vi "Oxford-1820-Main.vi"() -> ()   [LabVIEW 2016]
uses:
  <instrlib>/Mercury iXX/Public/Controls/Unit String.ctl
  <instrlib>/Mercury iXX/Public/Libraries/Heater/Controls/Heater Device (Read).ctl
  <instrlib>/Mercury iXX/Public/Controls/Manufacturing Data.ctl
  <instrlib>/Mercury iXX/Public/Libraries/Heater/Controls/Heater Signals Cluster.ctl
  <instrlib>/Mercury iXX/Public/Libraries/Level Meter/Controls/Level Meter (Read).ctl
  <instrlib>/Mercury iXX/Public/Libraries/Level Meter/Controls/Nitrogen Configuration.ctl
  <instrlib>/Mercury iXX/Public/Libraries/Level Meter/Controls/Frequency Configuration.ctl
  <instrlib>/Mercury iXX/Public/Libraries/Level Meter/Controls/Signals.ctl
  <instrlib>/Mercury iXX/Public/Libraries/Level Meter/Controls/Helium Configuration.ctl
  <instrlib>/Mercury iXX/Public/Libraries/Level Meter/Controls/Resistance Configuration.ctl
  <instrlib>/Mercury iXX/Public/Libraries/Level Meter/Controls/Pre-Pulse.ctl
  <instrlib>/Mercury iXX/Public/Libraries/Level Meter/Controls/Pulse.ctl
  <instrlib>/Mercury iXX/Public/Libraries/Auxiliary/Controls/AUX Device (Read).ctl
  <instrlib>/Mercury iXX/Public/Libraries/Auxiliary/Controls/AUX Signals (Read).ctl
  <instrlib>/Mercury iXX/Public/Libraries/Magnet/Controls/Device (Read).ctl
  <instrlib>/Mercury iXX/Public/Libraries/Magnet/Controls/Signals (Read).ctl
  <instrlib>/Mercury iXX/Public/Libraries/Magnet/Controls/Identifier.ctl
  <instrlib>/Mercury iXX/Public/Libraries/Temperature/Controls/Calibration Cluster.ctl
  <instrlib>/Mercury iXX/Public/Libraries/Temperature/Controls/Calibration Interpolation.ctl
  <instrlib>/Mercury iXX/Public/Libraries/Temperature/Controls/Excitation Cluster.ctl
  <instrlib>/Mercury iXX/Public/Libraries/Temperature/Controls/Excitation Type.ctl
  <instrlib>/Mercury iXX/Public/Libraries/Pressure/Controls/Pressure Signals Cluster.ctl
  <instrlib>/Mercury iXX/Mercury iXX.lvlib
  <instrlib>/Mercury iXX/Public/Controls/Comms Transport Layer.ctl
  <instrlib>/Mercury iXX/Public/Libraries/Pressure/Open/Open Pressure Device.vi
  <instrlib>/Mercury iXX/Public/Libraries/Pressure.lvlib
  <instrlib>/Mercury iXX/Public/Libraries/Pressure/Configuration/Read/Pressure Device (Read).vi
  <instrlib>/Mercury iXX/Public/Libraries/System/Read/Display Automatic Dimming (Read).vi
  <instrlib>/Mercury iXX/Public/Libraries/System.lvlib
  <instrlib>/Mercury iXX/Public/Libraries/System/Read/Display Automatic Dimming Time (Read).vi
  <instrlib>/Mercury iXX/Public/Libraries/System/Read/Display Brightness (Read).vi
  <instrlib>/Mercury iXX/Public/Libraries/System/Read/Mode (Read).vi
  <instrlib>/Mercury iXX/Public/Libraries/System/Read/Serial Number (Read).vi
  <instrlib>/Mercury iXX/Public/Libraries/System/Read/FVer (Read).vi
  <instrlib>/Mercury iXX/Public/Libraries/System/Read/HVer (Read).vi
  <instrlib>/Mercury iXX/Public/Libraries/System/Set/DateTime (Set).vi
  <instrlib>/Mercury iXX/Public/Libraries/Temperature/Signals/Read/Temperature (Read).vi
  <instrlib>/Mercury iXX/Public/Libraries/Temperature.lvlib
  <instrlib>/Mercury iXX/Public/Libraries/Temperature/Configuration/Read/Calibration Cold Limit (Read).vi
  <instrlib>/Mercury iXX/Public/Libraries/Temperature/Configuration/Read/Calibration Hot Limit (Read).vi
  <instrlib>/Mercury iXX/Public/Libraries/Temperature/Configuration/Read/Excitation Type (Read).vi
  <instrlib>/Mercury iXX/Public/Libraries/Temperature/Configuration/Read/Temperature Sensor (Read).vi
  <instrlib>/Mercury iXX/Public/Libraries/Temperature/Configuration/Read/Temperature Device (Read).vi
  <instrlib>/Mercury iXX/Public/Libraries/Temperature/Configuration/Read/Nickname (Read).vi
  <instrlib>/Mercury iXX/Public/Libraries/Temperature/Configuration/Read/Excitation Magnitude (Read).vi
  <instrlib>/Mercury iXX/Public/Libraries/Temperature/Configuration/Read/Serial Number (Read).vi
  <instrlib>/Mercury iXX/Public/Libraries/System/Read/Catalogue (Read).vi
  <instrlib>/Mercury iXX/Public/Libraries/System/Read/Flash Space (Read).vi
  <instrlib>/Mercury iXX/Public/Libraries/System/Read/DateTime (Read).vi
  <instrlib>/Mercury iXX/Public/Libraries/System/Read/Time (Read).vi
  <instrlib>/Mercury iXX/Public/Libraries/System/Read/Date (Read).vi
  <instrlib>/Mercury iXX/Public/Libraries/System/Open/Open System.vi
  <instrlib>/Mercury iXX/Public/Libraries/Temperature/Open/Open Temperature Device.vi
  <instrlib>/Mercury iXX/Public/Libraries/Auxiliary/Open/Open Auxiliary Device.vi
  <instrlib>/Mercury iXX/Public/Libraries/Auxiliary.lvlib
  <instrlib>/Mercury iXX/Public/Libraries/Auxiliary/Signals/Read/Percent Open (Read).vi
  <instrlib>/Mercury iXX/Public/Libraries/Magnet/Open/Open Magnet Device.vi
  <instrlib>/Mercury iXX/Public/Libraries/Magnet.lvlib
  <instrlib>/Mercury iXX/Public/Libraries/Magnet/Configuration/Read/PSU Action Status (Read).vi
  <instrlib>/Mercury iXX/Public/Libraries/Magnet/Configuration/Read/Magnet Device (Read).vi
  <instrlib>/Mercury iXX/Public/Libraries/Temperature/Signals/Read/Voltage (Read).vi
  <instrlib>/Mercury iXX/Private/Controls/Query Dynamic Reference.ctl
  <instrlib>/Mercury iXX/Public/Controls/Mercury Reference.ctl
  <instrlib>/Mercury iXX/Public/Libraries/Level Meter/Open/Open Level Meter Device.vi
  <instrlib>/Mercury iXX/Public/Libraries/Level Meter.lvlib
  <instrlib>/Mercury iXX/Public/Libraries/Level Meter/Signals/Read/Probe Level Nitrogen (Read).vi
  <instrlib>/Mercury iXX/Public/Libraries/Level Meter/Signals/Read/Probe Level Helium (Read).vi
  <instrlib>/Mercury iXX/Public/Libraries/Magnet/Signals/Read/Switch Heater Status (Read).vi
  <instrlib>/Mercury iXX/Public/Libraries/Magnet/Signals/Read/Current (Read).vi
  <instrlib>/Mercury iXX/Public/Libraries/Magnet/Configuration/Set/PSU Action Status (Set).vi
  <instrlib>/Mercury iXX/Public/Libraries/Magnet/Controls/PSU Actions.ctl
  <instrlib>/Mercury iXX/Public/Libraries/Magnet/Controls/Switch Heater.ctl
  SMOs/Instrument.Oxford1820/Instrument.Oxford1820.lvclass
  <instrlib>/Mercury iXX/Public/Libraries/Lambda/Configuration/Set/Lambda Percentage Flow (Set).vi
  <instrlib>/Mercury iXX/Public/Libraries/Lambda.lvlib
  <instrlib>/Mercury iXX/Public/Libraries/Lambda/Open/Open Lambda Device.vi
  <instrlib>/Mercury iXX/Public/Controls/Response String.ctl
  <instrlib>/Mercury iXX/Public/Libraries/Temperature/Signals/Read/Resistance (Read).vi
  <instrlib>/Mercury iXX/Public/Libraries/Temperature/Configuration/Set/Excitation Magnitude (Set).vi
  <instrlib>/Mercury iXX/Public/Libraries/Magnet/Signals/Read/Voltage (Read).vi
  SMOs/Instrument.Oxford1820/Typedefs/Status.ctl
  SMOs/Instrument.Oxford1820/Typedefs/Actions.ctl
  <instrlib>/Mercury iXX/Public/Libraries/System/Controls/User Mode.ctl
  <instrlib>/Mercury iXX/Public/Libraries/System/Set/Mode (Set).vi
  <instrlib>/Mercury iXX/Public/Libraries/Heater/Signals/Read/Power (Read).vi
  <instrlib>/Mercury iXX/Public/Libraries/Heater.lvlib
  <instrlib>/Mercury iXX/Public/Libraries/Heater/Signals/Read/Current (Read).vi
  <instrlib>/Mercury iXX/Public/Libraries/Auxiliary/Signals/Read/Position (Read).vi
  <instrlib>/Mercury iXX/Public/Libraries/Level Meter/Signals/Read/Probe Count Nitrogen (Read).vi
  <instrlib>/Mercury iXX/Public/Libraries/Magnet/Signals/Read/Current Rate (Read).vi
  <userlib>/_OpenG.lib/error/error.llb/Filter Error Codes (Array)__ogtk.vi
  <instrlib>/Mercury iXX/Public/Libraries/Heater/Configuration/Read/Nickname (Read).vi
  <instrlib>/Mercury iXX/Public/Libraries/Heater/Configuration/Read/Voltage Limit (Read).vi
  <instrlib>/Mercury iXX/Public/Libraries/Heater/Configuration/Read/Serial Number (Read).vi
  <instrlib>/Mercury iXX/Public/Libraries/Heater/Configuration/Read/Heater Device (Read).vi
  <instrlib>/Mercury iXX/Public/Libraries/Heater/Open/Open Heater Device.vi
  <instrlib>/Mercury iXX/Public/Libraries/Heater/Signals/Read/Voltage (Read).vi
  <instrlib>/Mercury iXX/Public/Libraries/Heater/Configuration/Read/Maximum Power (Read).vi
  <instrlib>/Mercury iXX/Public/Libraries/Heater/Configuration/Read/Nominal Resistance (Read).vi
  <instrlib>/Mercury iXX/Public/Libraries/Auxiliary/Configuration/Read/Stepper Speed (Read).vi
  <instrlib>/Mercury iXX/Public/Libraries/Auxiliary/Configuration/Read/Valve Gearing (Read).vi
  <instrlib>/Mercury iXX/Public/Libraries/Auxiliary/Configuration/Read/Temperature Error Voltage Sensitivity (Read).vi
  <instrlib>/Mercury iXX/Public/Libraries/Auxiliary/Configuration/Read/Temperature Error Sensitivity (Read).vi
  <instrlib>/Mercury iXX/Public/Libraries/Auxiliary/Configuration/Read/Gas Flow Scaling (Read).vi
  <instrlib>/Mercury iXX/Public/Libraries/Auxiliary/Configuration/Read/Minimum Gas Flow (Read).vi
  <instrlib>/Mercury iXX/Public/Libraries/Auxiliary/Configuration/Read/Serial Number (Read).vi
  <instrlib>/Mercury iXX/Public/Libraries/Auxiliary/Configuration/Read/Aux Device (Read).vi
  <instrlib>/Mercury iXX/Public/Libraries/Pressure/Signals/Read/Voltage (Read).vi
  <instrlib>/Mercury iXX/Public/Libraries/Pressure/Signals/Read/Current (Read).vi
  <instrlib>/Mercury iXX/Public/Libraries/Pressure/Configuration/Read/Nickname (Read).vi
  <instrlib>/Mercury iXX/Public/Libraries/Level Meter/Signals/Read/Probe Resistance Helium (Read).vi
  <instrlib>/Mercury iXX/Public/Libraries/Level Meter/Configuration/Read/Nitrogen Pulse Count Period (Read).vi
  <instrlib>/Mercury iXX/Public/Libraries/Level Meter/Configuration/Read/Nitrogen Freq at 100 (Read).vi
  <instrlib>/Mercury iXX/Public/Libraries/Level Meter/Configuration/Read/Helium Pulse Duration (Read).vi
  <instrlib>/Mercury iXX/Public/Libraries/Level Meter/Configuration/Read/Helium Pulse Mag (Read).vi
  <instrlib>/Mercury iXX/Public/Libraries/Level Meter/Configuration/Read/Helium Probe Resistance (Read).vi
  <instrlib>/Mercury iXX/Public/Libraries/Level Meter/Configuration/Read/Serial Number (Read).vi
  <instrlib>/Mercury iXX/Public/Libraries/Level Meter/Configuration/Read/Level Meter Device (Read).vi
  <instrlib>/Mercury iXX/Public/Libraries/Magnet/Configuration/Read/Software Voltage Limit (Read).vi
  <instrlib>/Mercury iXX/Public/Libraries/Magnet/Configuration/Read/Switch Present (Read).vi
  <instrlib>/Mercury iXX/Public/Libraries/Magnet/Configuration/Read/Current to Field Factor (Read).vi
  <instrlib>/Mercury iXX/Public/Libraries/Magnet/Configuration/Read/Current Limit (Read).vi
  <instrlib>/Mercury iXX/Public/Libraries/Magnet/Configuration/Read/Output Configuration (Read).vi
  <instrlib>/Mercury iXX/Public/Libraries/Magnet/Configuration/Read/Bipolar Output (Read).vi
  <instrlib>/Mercury iXX/Public/Libraries/Magnet/Configuration/Read/Serial Number (Read).vi
  <instrlib>/Mercury iXX/Public/Libraries/Magnet/Signals/Read/Target Field (Read).vi
  <instrlib>/Mercury iXX/Public/Libraries/Magnet/Signals/Read/Target Field Rate (Read).vi
  <instrlib>/Mercury iXX/Public/Libraries/Magnet/Signals/Read/Field (Read).vi
  <instrlib>/Mercury iXX/Public/Libraries/Magnet/Signals/Read/Persistant Field (Read).vi
  <instrlib>/Mercury iXX/Public/Libraries/Magnet/Configuration/Set/Switch Heater Current (Set).vi
  <instrlib>/Mercury iXX/Public/Libraries/Magnet/Signals/Read/Persistant Current (Read).vi
  <instrlib>/Mercury iXX/Public/Libraries/Magnet/Signals/Set/Switch Heater No Check (Set).vi
  <instrlib>/Mercury iXX/Public/Libraries/Magnet/Signals/Set/Target Field (Set).vi
  <instrlib>/Mercury iXX/Public/Libraries/Magnet/Signals/Set/Target Field Rate (Set).vi
  <instrlib>/Mercury iXX/Public/Libraries/Lambda/Configuration/Set/Lambda Flow Auto (Set).vi
  <instrlib>/Mercury iXX/Public/Libraries/Level Meter/Configuration/Set/Pulse Slow-Fast (Set).vi
panel:
  out "LPF ON":timestamp
  in  "Tab Control":T1(tab)
  in  "Enable RS232 Panel":bool
  out "LEDs":bool[](array[boolean])
  out "Iteration Time":dbl
  in  "Percentage Open":dbl=100.0 format="%#_13g"
  out "PS Heat on or off (sec)":dbl format="%<%H:%M:%S>t"
  out "LPF on (min)":dbl=5373.0 format="%<%H:%M:%S>t"
  out "Magnet Status 2":string
  in  "OK":bool
  out "LPF Resistance":dbl=4.2075 format="%_3f ohms"
  out "Magnet Resistance":dbl=3.8705 format="%_3f ohms"
  out "ETA":timestamp format="%<%I:%M:%S %p\n%m/%d/%y>T"
  in  "Open Needle Valve":bool
  in  "Close Needle Valve":bool
  in  "Lambda":bool
  out "LPF Pressure":dbl format="%_5f mB"
  out "LPF Needle Valve (%)":dbl format="%_6g"
  out "LPF Temperature":dbl=4.2075 format="%_2f K"
  out "Magnet Temperature":dbl=3.8705 format="%_2f K"
  out "He LVL Chart":dbl(slide)=52.0833 scale=0.0..100.0
  out "N2 LVL Chart":dbl(slide)=61.3025 scale=0.0..100.0
  in  "Remote Mode":bool
  out "Power Supply Field (T)":dbl=0.0001 format="%#.5f"
  out "Magnet Field (T)":dbl format="%.5f"
  out "Voltage (V)":dbl=-0.0003 format="%.5f"
  out "Current (A)":dbl=0.0006 format="%.5f"
  out "N2 LEVEL":dbl=61.3025 format="%.0f %"
  out "He LEVEL":dbl=52.0833 format="%.0f %"
  in  "Fast/Slow Fill":bool
  out "Magnet Field (T)":dbl(knob) caption="Voltage (V)" scale=-20.0..20.0
  out "SWITCH HEATER":bool
  in  "PS Heat":bool
  in  "Clamp":bool
  in  "To Set":bool
  in  "To Zero":bool
  in  "Hold":bool
  out "Magnet Status":string="Clamped"
  out "Target Field Rate (T/min)":dbl=1.0 format="%.5f"
  out "Target Field (T)":dbl format="%#.5f"
  in  "Target Rate (T/min)":dbl=0.1 format="%.5f"
  in  "Target Field (T)":dbl format="%#.5f"
  in  "Send to IPS":bool
  out "Voltage (V)":dbl(knob)=-0.0003 scale=-10.0..10.0
  out "Current (A)":dbl(knob)=0.0006 scale=-180.0..180.0
  in  "Mercury Functions":T2(tab)=enum."ITC: Temperature"
  out "time stamp":timestamp=timestamp(3543841780 s since 1904-01-01)
  out "Free Space":i32=166384 caption="Free Space (KB)"
  out "Set Date Response":string="VALID"
  out "String":string="NORM" caption="User Mode"
  out "Date":string="2016:04:18"
  out "Time":string="11:29:40"
  out "Hardware Version":string="65"
  out "Firmware Version":string="2.2.6.20"
  out "Serial Number":string="154650110"
  out "ITC Devices":string[](array[string])=["DB4.G1:AUX", "DB8.P1:PRES", "MB0.H1:HTR", "MB1.T1:TEMP"]
  out "S/W Version(s)":string[](array[string])=["2.2.6.20\n"]
  out "Serial Number(s)":string[](array[string])=["154650110"]
  out "# of Instruments":i32=1
  out "Automatic Dimming":string="OFF"
  out "Dimming Time":string="5"
  out "Display Brightness":string="100"
  in  "ITC IP Address":string="130.49.180.101"
  out "Excitation Magnitude":dbl=5.0
  out "Sensor Type":string="NTC"
  out "Excitation Type":string="UNIP"
  out "Hot Limit":dbl=1000.0
  out "H Unit":T3="K"
  out "Cold Limit":dbl=1000.0
  out "C Unit":T3="K"
  out "Unit":T3
  out "Voltage":dbl=0.005
  out "V Unit":T3="V"
  out "Temperature":dbl=4.2075
  out "T Unit":T3="K"
  out "Temp S/N":string="154650110"
  out "T Nickname":string="Mag_AB_MB1"
  out "ITC Calibration":T4
  out "ITC Excitation":T6
  out "ITC Manufacturing":T8
  out "Heater Device Settings":T9={"Manufacturing"={"Hardware Version"="65", "Firmware Version"="2.3", "Serial Number"="154650110"}, "Nickname"="MB0.H1", "Voltage Limit"="1", "Nominal Resistance"="10", "Maximum Power"="0.1000", "Heater Signals"={"Voltage"="0.0507V", "Current"="-0.0000A", "Power"="0.0000W"}, "Status"="2"}
  out "Htr C Unit":T3="A"
  out "Htr P Unit":T3="W"
  out "Htr V Unit":T3="V"
  out "Htr Current":dbl=-0.0
  out "Htr Power":dbl
  out "Htr Voltage":dbl=0.0507
  out "Power Unit":T3
  out "Volt Unit":T3
  out "Res Unit":T3
  out "Maximum Power":dbl=0.1
  out "Htr Resistance":dbl=10.0
  out "Htr Voltage Limit":dbl=1.0
  out "Htr S/N":string="154650110"
  out "Htr Nickname":string="MB0.H1"
  out "Nickname":string="Lam_P_DB8"
  out "Current":dbl=-0.0
  out "Voltage":dbl=-8.219999999999999e-05
  out "Manufacturing":T8
  out "Pressure Signals":T11
  out "Auxiliary Device Details":T12={"Manufacturing"={"Hardware Version"="65", "Firmware Version"="3.1", "Serial Number"="154650084"}, "Min Flow"=0.0, "Scaling Factor"=50.0, "Temp Err"=9.0, "Temp V Err"=11.0, "Gear"=2, "Speed"=2, "Signals"={"Position"=0.0, "% Open"=0.0, "I0"="ON", "I1"="OFF", "I2"="OFF", "I3"="OFF", "O0"="OFF", "O1"="OFF", "O2"="OFF", "O3"="OFF"}, "Nickname"="DB4.G1", "Status"="0"} {"Signals"."% Open" min=0.0 max=100.0 step=0.1 format="%.4f"; "Signals"."Position" max=20.0 step=1.0 format="%.4f"; "Speed" max=7 step=1; "Gear" max=7 step=1; "Temp V Err" min=0.0 max=20.0 step=0.1; "Temp Err" min=0.0 max=20.0 step=0.1; "Scaling Factor" min=0.0 max=99.0 step=0.1; "Min Flow" min=0.0 max=20.0 step=0.1}
  out "Aux S/N":string="154650084"
  out "Min Flow":dbl caption="Minimum Gas Flow" format="%#.1f"
  out "Scaling Factor":dbl=50.0 caption="Gas Flow Scaling Factor" format="%#.1f"
  out "Temp Err":dbl=9.0 caption="Temperature Error Sensitivity" format="%#.1f"
  out "Temp V Err":dbl=11.0 caption="Temperature Voltage Error Sensitivity" format="%#.1f"
  out "Gear":u32=2 caption="Valve Gearing"
  out "Speed":u32=2 caption="Stepper Speed"
  out "Unit 2":T3
  out "Unit 3":T3
  out "Unit 4":T3
  out "Unit 5":T3
  out "Unit 6":T3
  out "Unit 7":T3
  out "Position":u32
  out "% Open":dbl caption="Percentage Open (%)"
  out "Unit":T3
  out "Unit":T3="%"
  out "time stamp 2":timestamp=timestamp(3543841781 s since 1904-01-01)
  out "Free Space 2":i32=166316 caption="Free Space (KB)"
  out "Set Date Response 2":string="VALID"
  out "String 2":string="NORM" caption="User Mode"
  out "Date 2":string="2016:04:18"
  out "Time 2":string="11:29:45"
  out "Hardware Version 2":string="65"
  out "Firmware Version 2":string="2.2.6.20"
  out "Serial Number 2":string="153350063"
  out "IPS Devices":string[](array[string])=["DB3.L1:LVL", "GRPX:PSU", "GRPY:PSU", "GRPZ:PSU", "MB1.T1:TEMP", "PSU.M1:PSU", "PSU.M2:PSU", "PSU.M3:PSU"]
  out "S/W Version(s) 2":string[](array[string])=["2.2.6.20\n"]
  out "Serial Number(s) 2":string[](array[string])=["153350063"]
  out "# of Instruments 2":i32=1
  out "Automatic Dimming 2":string="OFF"
  out "Dimming Time 2":string="5"
  out "Display Brightness 2":string="100"
  in  "IPS IP Address":string="130.49.180.102"
  out "LVL Device DetailSettings":T14={"Manufacturing"={"Hardware Version"="65", "Firmware Version"="2.2", "Serial Number"="152450013"}, "Nitrogen Configuration"={"Frequency Configuration"={"Freq 0%"=0.0, "Freq 100%"=0.0}, "Pulse Period"=0.0}, "Signals"={"Helium Signals"={"Resistance"=75.5626, "Level"=52.0833}, "Nitrogen Signals"={"Count"=8800.0, "Freq"=487361.0, "Level"=61.3445}}, "Nickname"="DB3.L1", "Status"="0", "Helium Configuration"={"Resistance Configuration"={"Res 0%"=0.0, "Res 100%"=0.0}, "Pre-Pulse"={"Magnitude"=0.0, "Duration"=0.0}, "Pulse"={"Magnitude"=0.0, "Duration"=0.0, "Delay"=0.0}}}
  out "LVL S/N":string="152450013"
  out "LVL P Magnitude":dbl=125.0 caption="Pulse Magnitude (mA)"
  out "LVL P Duration":dbl=5.0 caption="Pulse Duration (s)"
  out "N Freq 100%":dbl=7880.0 caption="Frequency at 100% (Hz)"
  out "N Pulse Period":dbl=1000.0 caption="Pulse Period (ms)"
  out "He Res Config":T19={"Res 0%"=149.0, "Res 100%"=8.0}
  out "He Resistance":dbl=75.5626 caption="Resistance (Ohms)"
  out "He Level":dbl=52.0833 caption="Helium Level (%)"
  out "N Counter":u32 caption="Counter"
  out "N Level":dbl=61.3445 caption="Nitrogen Level (%)"
  out "Excitation Magnitude 2":dbl=5.0
  out "Sensor Type 2":string="NTC"
  out "Excitation Type 2":string="UNIP"
  out "Hot Limit 2":dbl=1000.0
  out "H Unit 2":T3="K"
  out "Cold Limit 2":dbl=1000.0
  out "C Unit 2":T3="K"
  out "Unit 12":T3
  out "Voltage 2":dbl=0.005
  out "V Unit 2":T3="V"
  out "Temperature 2":dbl=3.8706
  out "T Unit 2":T3="K"
  out "Temp S/N 2":string="153350063"
  out "T Nickname 2":string="MB1.T1"
  out "IPS Calibration":T4
  out "IPS Excitation":T6
  out "IPS Manufacturing":T8
  out "Magnet Device Details":T22={"Manufacturing"={"Hardware Version"="NOT_FOUND", "Firmware Version"="NOT_FOUND", "Serial Number"="NOT_FOUND"}, "Nickname"="GRPZ", "Bipolar Output"="ON", "String"="PARA", "Current Limit"=174.0, "AtoB"=8.688, "Inductance"=39.406, "Switch Present"="PSU.M1", "Swh Htr Current"=86.0, "SW VLIM"=9.0, "V Trans Time"=1000.0, "Magnet PSU Signals"={"Voltage"=-0.0002, "Current"=0.0002, "Current Rate"=100.0, "Field"=0.0001, "Field Rate"=11.5101, "Persistant Current"=0.0003, "Persistant Field"=0.0, "Target Current"=0.0, "Target Field"=0.0, "Target Current Rate"=8.688, "Target Field Rate"=1.0, "Switch Heater Status (SWHT)"="OFF", "Switch Heater Status (SWHN)"="OFF"}, "PSU Action"="CLMP", "Status"="40000000", "Level Limit"=0.0, "Temperature Limit"=999.0} {"Temperature Limit" format="%#.1f"; "Level Limit" format="%#.1f"; "V Trans Time" format="%#.1f"; "SW VLIM" format="%#.1f"; "Swh Htr Current" format="%#.1f"; "Inductance" format="%#.1f"; "AtoB" format="%#.1f"; "Current Limit" format="%#.1f"}
  out "Mag S/N":string="NOT_FOUND"
  out "Bipolar Output":string="ON"
  out "Out Config":string="PARA" caption="Output Configuration"
  out "Current Limit":dbl=174.0 caption="Current Limit (A)" format="%#.1f"
  out "AtoB":dbl=8.688 caption="Current Field Factor (A/T)" format="%#.1f"
  out "Switch Present":string="PSU.M1"
  out "SW VLIM":dbl=9.0 caption="Software Voltage Limit (V)" format="%#.1f"
  out "Unit 8":T3
  out "Unit 9":T3
  out "Unit 10":T3
  out "Current Rate":dbl=100.0
  out "PSU Act Stat":string="CLMP" caption="PSU Action Status"
  out "Unit 11":T3="A/min"
  in  "Device Identifier":T24="GRPZ"
  out "M3 Voltage":dbl
  out "M3 Current":dbl
  out "M2 Voltage":dbl
  out "M2 Current":dbl
  out "M1 Voltage":dbl
  out "M1 Current":dbl
  out "Error List":T25(array[cluster])
  out "PS ON/OFF":timestamp format="%<%I:%M:%S %p>T"
  in  "Heater Current":bool
  in  "Swh Htr Current (mA)":dbl=90.0 format="%#_13g"
  # "v2017/10/10"
  # "Voltage (V)"
  # "Magnet (T)"
  # "Current (A)"
  # "Slow Rates\nCurrent Range (A)     Field Range (T)    Rate (T/min)\n0       -- 100        0    -- 11.5       0.91\n100     -- 150        11.5 -- 17.2       0.23\n150     -- 155.467    17.2 -- 18         0.11\n155.567 -- 172.471    18   -- 20         0.11"
  # "Fast Rates\nCurrent Range (A)     Field Range (T)    Rate (T/min)\n0       -- 155.467    0    -- 18         1.0\n155.567 -- 172.471    18   -- 20         0.25"
  # "ITC: 101\nIPS: 102\nIPS VR: 67"
  # "ITC: 101\nIPS: 102\nIPS VR: 67"
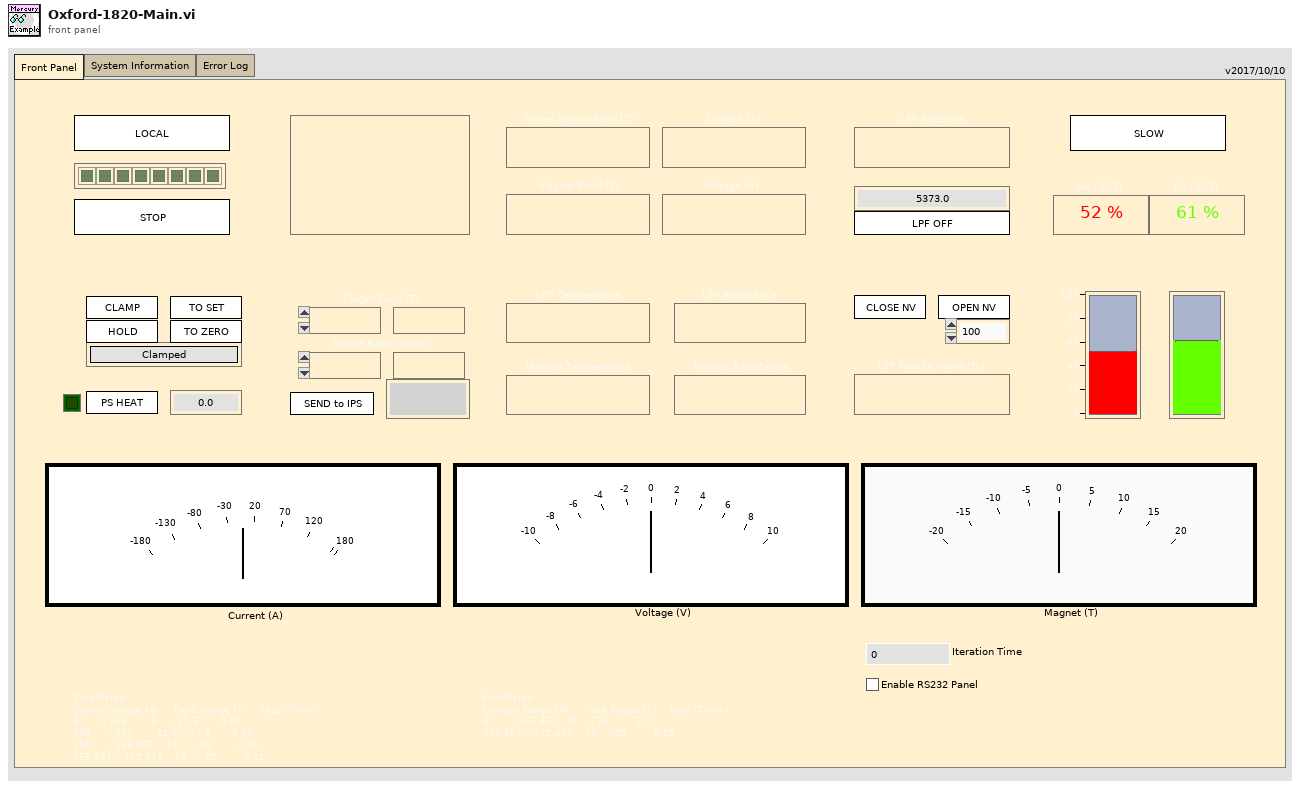
[diagram p1: front panel]
types:
  T1 = enum32{"Front Panel", "System Information", "Error Log"}
  T2 = enum32{"ITC: System", "ITC: Temperature", "ITC: Heater", "ITC: Pressure", "ITC: Auxiliary", "IPS: System", "IPS: Level Meter", "IPS: Temperature", "IPS: Magnet"}
  T3 = typedef "Mercury iXX.lvlib/Unit String.ctl" = string
  T4 = typedef "Mercury iXX.lvlib/Temperature.lvlib/Calibration Cluster.ctl" = cluster{"Filename":string, "Interpolation":T5, "Scaling Factor":string, "Offset Factor":string, "Hot Limit":string, "Cold Limit":string, "Last Calibration":string, "Reference":string}
  T5 = typedef "Mercury iXX.lvlib/Temperature.lvlib/Calibration Interpolation.ctl" = string
  T6 = typedef "Mercury iXX.lvlib/Temperature.lvlib/Excitation Cluster.ctl" = cluster{"Excitation Type":T7, "Magnitude":string}
  T7 = typedef "Mercury iXX.lvlib/Temperature.lvlib/Excitation Type.ctl" = string
  T8 = typedef "Mercury iXX.lvlib/Manufacturing Data.ctl" = cluster{"Hardware Version":string, "Firmware Version":string, "Serial Number":string}
  T9 = typedef "Mercury iXX.lvlib/Heater.lvlib/Heater Device (Read).ctl" = cluster{"Manufacturing":T8, "Nickname":string, "Voltage Limit":string, "Nominal Resistance":string, "Maximum Power":string, "Heater Signals":T10, "Status":string}
  T10 = typedef "Mercury iXX.lvlib/Heater.lvlib/Heater Signals Cluster.ctl" = cluster{"Voltage":string, "Current":string, "Power":string}
  T11 = typedef "Mercury iXX.lvlib/Pressure.lvlib/Pressure Signals Cluster.ctl" = cluster{"Voltage":string, "Current":string, "Power":string, "Pressure":string}
  T12 = typedef "Mercury iXX.lvlib/Auxiliary.lvlib/AUX Device (Read).ctl" = cluster{"Manufacturing":T8, "Min Flow":dbl, "Scaling Factor":dbl, "Temp Err":dbl, "Temp V Err":dbl, "Gear":u32, "Speed":u32, "Signals":T13, "Nickname":string, "Status":string}
  T13 = typedef "Mercury iXX.lvlib/Auxiliary.lvlib/AUX Signals (Read).ctl" = cluster{"Position":dbl, "% Open":dbl, "I0":string, "I1":string, "I2":string, "I3":string, "O0":string, "O1":string, "O2":string, "O3":string}
  T14 = typedef "Mercury iXX.lvlib/Level Meter.lvlib/Level Meter (Read).ctl" = cluster{"Manufacturing":T8, "Nitrogen Configuration":T15, "Signals":T17, "Nickname":string, "Status":string, "Helium Configuration":T18}
  T15 = typedef "Mercury iXX.lvlib/Level Meter.lvlib/Nitrogen Configuration.ctl" = cluster{"Frequency Configuration":T16, "Pulse Period":dbl}
  T16 = typedef "Mercury iXX.lvlib/Level Meter.lvlib/Frequency Configuration.ctl" = cluster{"Freq 0%":dbl, "Freq 100%":dbl}
  T17 = typedef "Mercury iXX.lvlib/Level Meter.lvlib/Signals.ctl" = cluster{"Helium Signals":cluster{"Resistance":dbl, "Level":dbl}, "Nitrogen Signals":cluster{"Count":dbl, "Freq":dbl, "Level":dbl}}
  T18 = typedef "Mercury iXX.lvlib/Level Meter.lvlib/Helium Configuration.ctl" = cluster{"Resistance Configuration":T19, "Pre-Pulse":T20, "Pulse":T21}
  T19 = typedef "Mercury iXX.lvlib/Level Meter.lvlib/Resistance Configuration.ctl" = cluster{"Res 0%":dbl, "Res 100%":dbl}
  T20 = typedef "Mercury iXX.lvlib/Level Meter.lvlib/Pre-Pulse.ctl" = cluster{"Magnitude":dbl, "Duration":dbl}
  T21 = typedef "Mercury iXX.lvlib/Level Meter.lvlib/Pulse.ctl" = cluster{"Magnitude":dbl, "Duration":dbl, "Delay":dbl}
  T22 = typedef "Mercury iXX.lvlib/Magnet.lvlib/Device (Read).ctl" = cluster{"Manufacturing":T8, "Nickname":string, "Bipolar Output":string, "String":string, "Current Limit":dbl, "AtoB":dbl, "Inductance":dbl, "Switch Present":string, "Swh Htr Current":dbl, "SW VLIM":dbl, "V Trans Time":dbl, "Magnet PSU Signals":T23, "PSU Action":string, "Status":string, "Level Limit":dbl, "Temperature Limit":dbl}
  T23 = typedef "Mercury iXX.lvlib/Magnet.lvlib/Signals (Read).ctl" = cluster{"Voltage":dbl, "Current":dbl, "Current Rate":dbl, "Field":dbl, "Field Rate":dbl, "Persistant Current":dbl, "Persistant Field":dbl, "Target Current":dbl, "Target Field":dbl, "Target Current Rate":dbl, "Target Field Rate":dbl, "Switch Heater Status (SWHT)":string, "Switch Heater Status (SWHN)":string}
  T24 = typedef "Mercury iXX.lvlib/Magnet.lvlib/Identifier.ctl" = string
  T25 = cluster{"time":timestamp, "code":i32, "source":string}[]
  T26 = enum32{"invalid app kind", "Development System", "Run Time System", "Student Edition", "Embedded LabVIEW", "Evaluation", "Custom"}
  T27 = cluster{"time":timestamp, "code":i32, "source":string}
  T28 = enum32{"Invalid", "Standard", "Closed", "Hidden", "Minimized", "Maximized"}
  T29 = typedef "Instrument.Oxford1820.lvclass/Status.ctl" = cluster{"Magnet Field":dbl, "PS Field":dbl, "Target Field":dbl, "Target Field Rate":dbl, "Voltage":dbl, "Current":dbl, "Switch":bool, "Mercury State":string}
  T30 = cluster{"Magnet Field":dbl, "PS Field":dbl, "Target Field":dbl, "Target Field Rate":dbl, "Voltage":dbl, "Current":dbl}
  T31 = typedef "Instrument.Oxford1820.lvclass/Actions.ctl" = cluster{"Hold":bool, "Clamp":bool, "To Set":bool, "To Zero":bool, "Send to IPS":bool, "PS Heat":bool, "Lambda":bool}
  T32 = typedef "Mercury iXX.lvlib/System.lvlib/User Mode.ctl" = string
  T33 = typedef "Mercury iXX.lvlib/Magnet.lvlib/Switch Heater.ctl" = string
  T34 = typedef "Mercury iXX.lvlib/Response String.ctl" = string
  T35 = typedef "Mercury iXX.lvlib/Mercury Reference.ctl" = cluster{"Comms":refnum<visa-resource-name>, "Device ID":string[], "Comms Layer":T36, "Command":string, "Query reference":T37}
  T36 = typedef "Mercury iXX.lvlib/Comms Transport Layer.ctl" = enum16{"Ethernet TCP/IP", "USB", "ISOBus - RS-232", "GPIB"}
  T37 = typedef "Mercury iXX.lvlib/Query Dynamic Reference.ctl" = refnum<vi>
  T38 = cluster{"Core":cluster{"Current VI Reference":refnum<vi>, "Close Panel on Exit?":bool}, "Mercury ITC Ref":T35, "Mercury IPS Ref":T35, "sentinel":bool, "Error Log":cluster{"time":timestamp, "code":i32, "source":string}[], "read ITC T?":bool, "counter":i32, "LEDs":bool[]}
  T39 = typedef "Filtered Error Details - Cluster__ogtk.ctl" = cluster{"code":i32, "source":string}
  T40 = cluster{"Current VI Reference":refnum<vi>, "Close Panel on Exit?":bool}
  T41 = typedef "Mercury iXX.lvlib/Temperature.lvlib/Temperature Sensor Type.ctl" = string
  T42 = typedef "Mercury iXX.lvlib/Temperature.lvlib/Temperature Device (Read).ctl" = cluster{"Manufacturing":T8, "Temperature Sensor Type":T41, "Excitation":T6, "Calibration":T4, "Control Loop":T43, "Temperature Signals":T44, "Nickname":string, "Status":string}
  T43 = typedef "Mercury iXX.lvlib/Temperature.lvlib/Loop Cluster.ctl" = cluster{"Heater":string, "Auxiliary":string, "Heater Auto":string, "Percentage Heat":string, "Temperature Set Point":string, "PID Auto (from file)":string, "P Value":string, "I Value":string, "D Value":string, "Auto PID Table Filename":string, "Flow Auto":string, "Target Heater Table":string, "Sweep mode":string, "Sweep Table Filename":string, "Percentage Flow":string}
  T44 = typedef "Mercury iXX.lvlib/Temperature.lvlib/Temperature Signals Cluster.ctl" = cluster{"Voltage":string, "Current":string, "Power":string, "Resistance":string, "Temperature":string, "Sensitivity":string, "Reference":string}
  T45 = typedef "Mercury iXX.lvlib/Pressure.lvlib/Pressure Device (Read).ctl" = cluster{"Manufacturing":T8, "Temperature Sensor Type":T46, "Calibration":T47, "Control Loop":T49, "Pressure Signals":T11, "Nickname":string, "Status":string}
  T46 = typedef "Mercury iXX.lvlib/Pressure.lvlib/Pressure Sensor Type.ctl" = string
  T47 = typedef "Mercury iXX.lvlib/Pressure.lvlib/Calibration Cluster.ctl" = cluster{"Filename":string, "Interpolation":T48, "Scaling Factor":string, "Offset Factor":string, "High Limit":string, "Low Limit":string, "Last Calibration":string}
  T48 = typedef "Mercury iXX.lvlib/Pressure.lvlib/Calibration Interpolation.ctl" = string
  T49 = typedef "Mercury iXX.lvlib/Pressure.lvlib/Loop Cluster.ctl" = cluster{"Heater":string, "Auxiliary":string, "Heater Auto":string, "Percentage Heat":string, "Pressure Set Point":string, "PID Auto (from file)":string, "P Value":string, "I Value":string, "D Value":string, "Auto PID Table Filename":string, "Flow Auto":string, "Target Heater Table":string, "Sweep mode":string, "Sweep Table Filename":string, "Percentage Flow":string}
  T50 = typedef "Mercury iXX.lvlib/Magnet.lvlib/Output Configuration.ctl" = string
  T51 = typedef "Mercury iXX.lvlib/Magnet.lvlib/PSU Actions.ctl" = string
  T52 = typedef "Instrument.Oxford1820.lvclass/Targets.ctl" = cluster{"Field (T)":dbl, "Field Rate (T/min)":dbl}
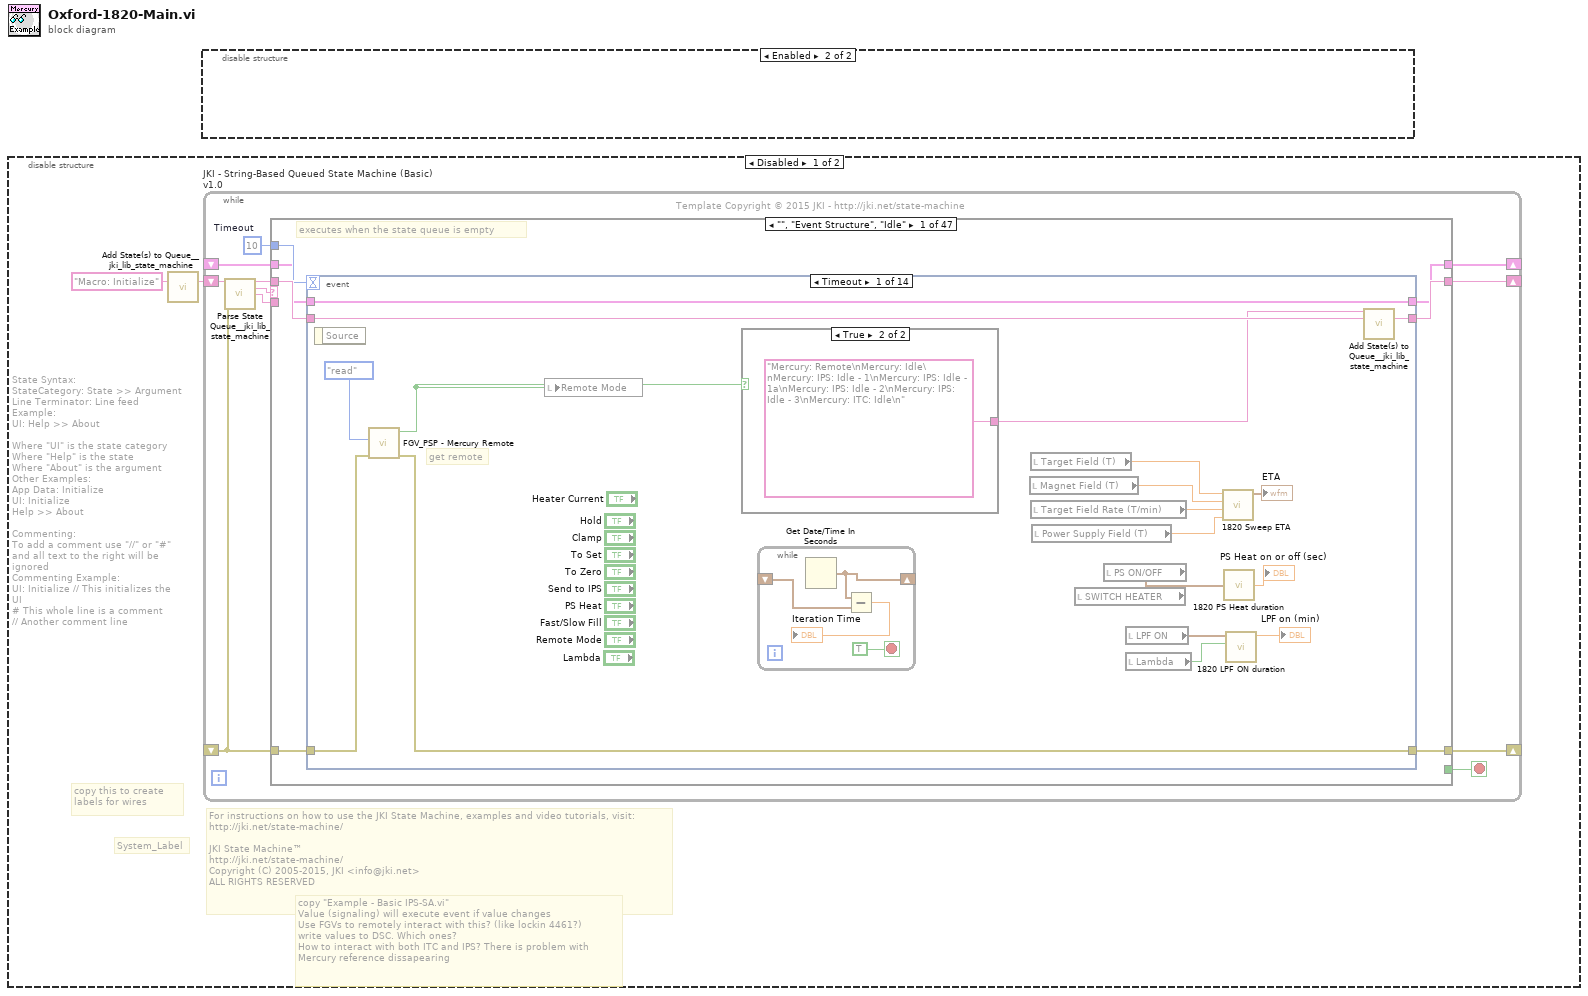
[diagram p0: block diagram]
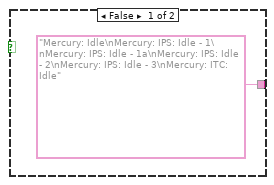
[diagram p2: hidden frame]
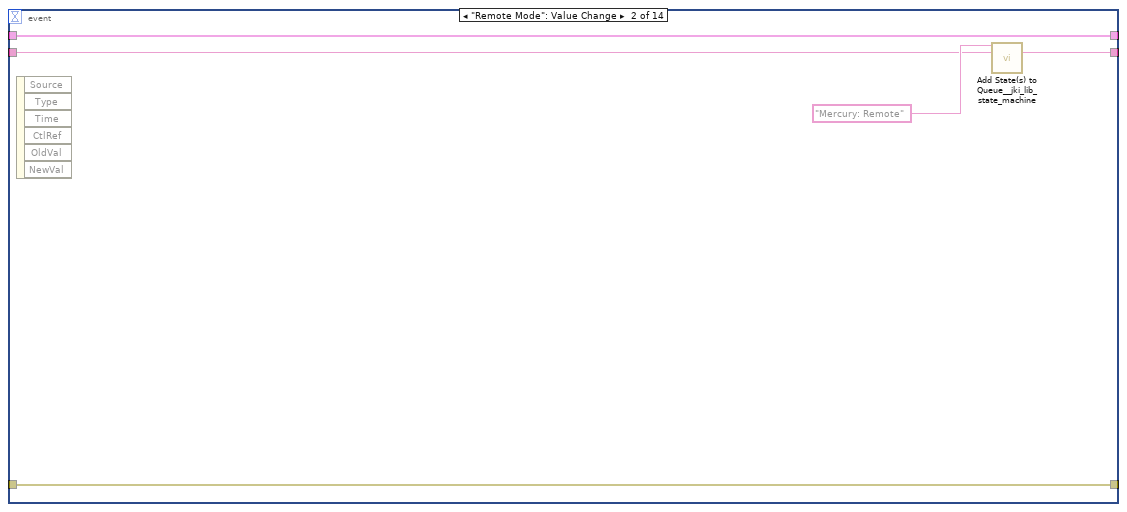
[diagram p3: hidden frame]
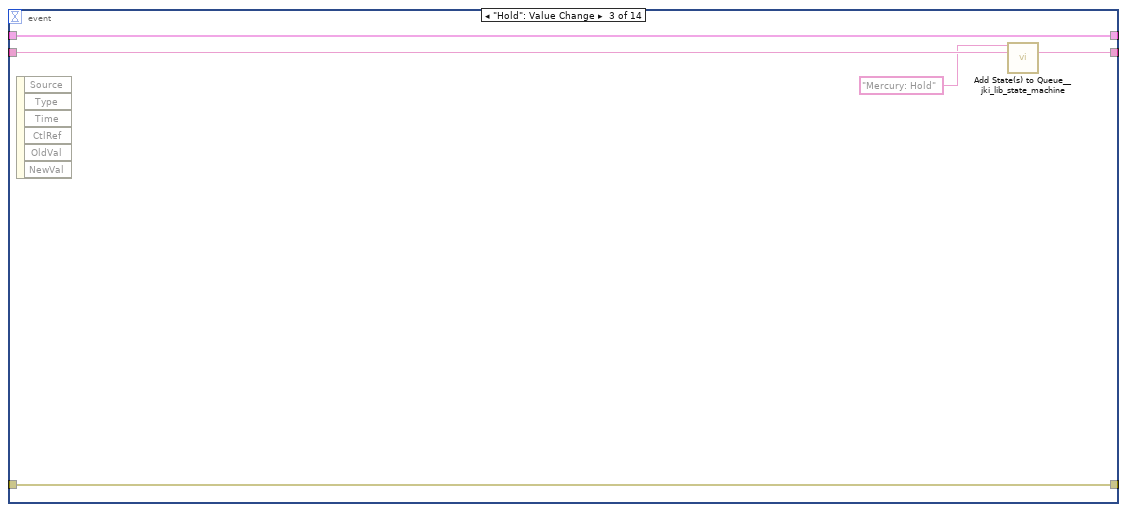
[diagram p4: hidden frame]
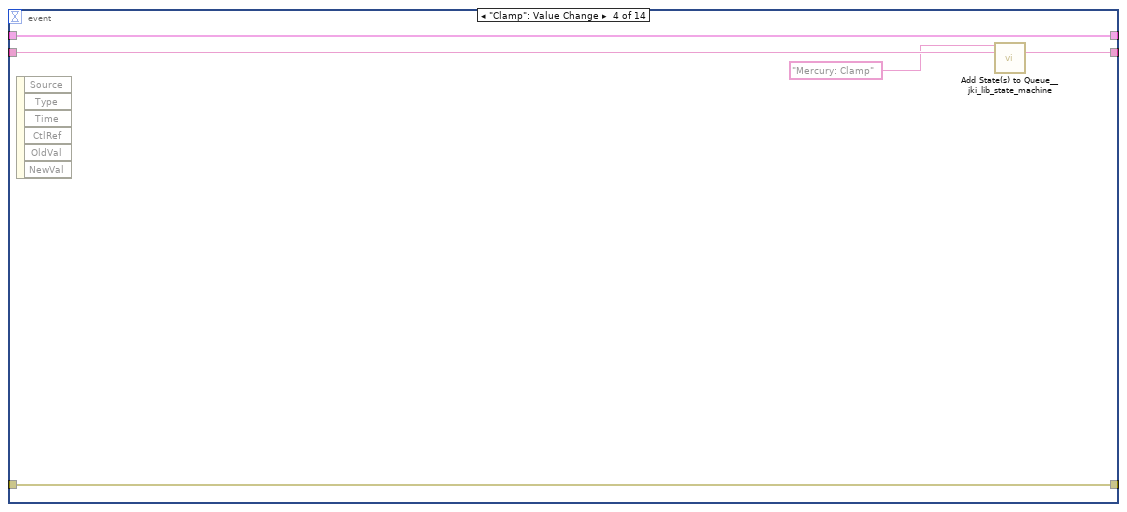
[diagram p5: hidden frame]
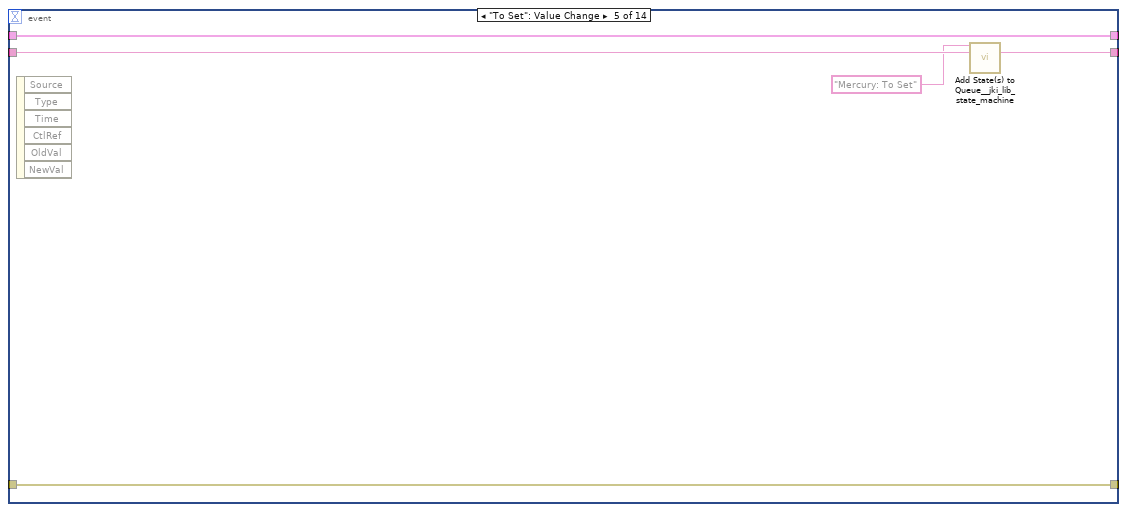
[diagram p6: hidden frame]
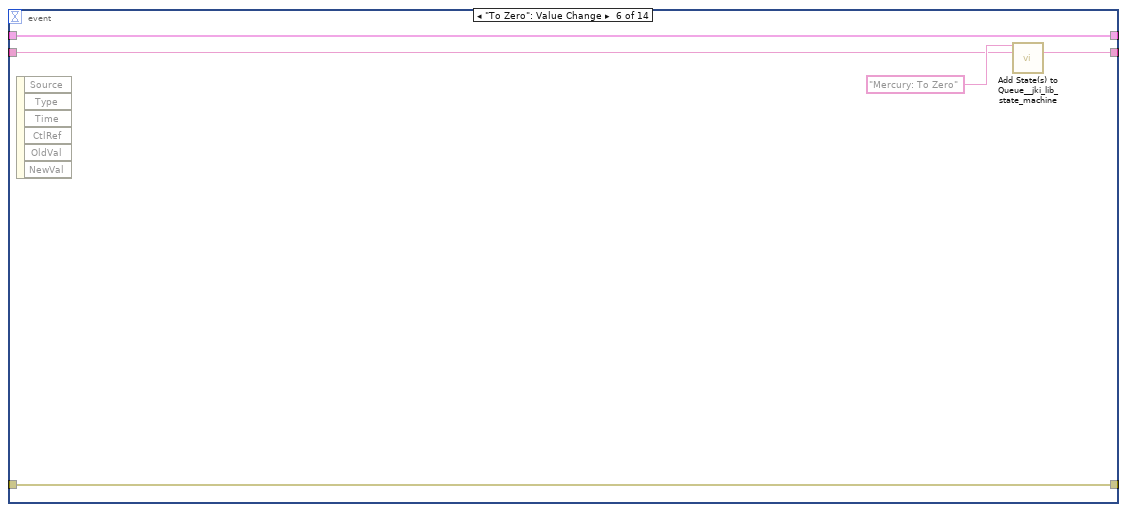
[diagram p7: hidden frame]
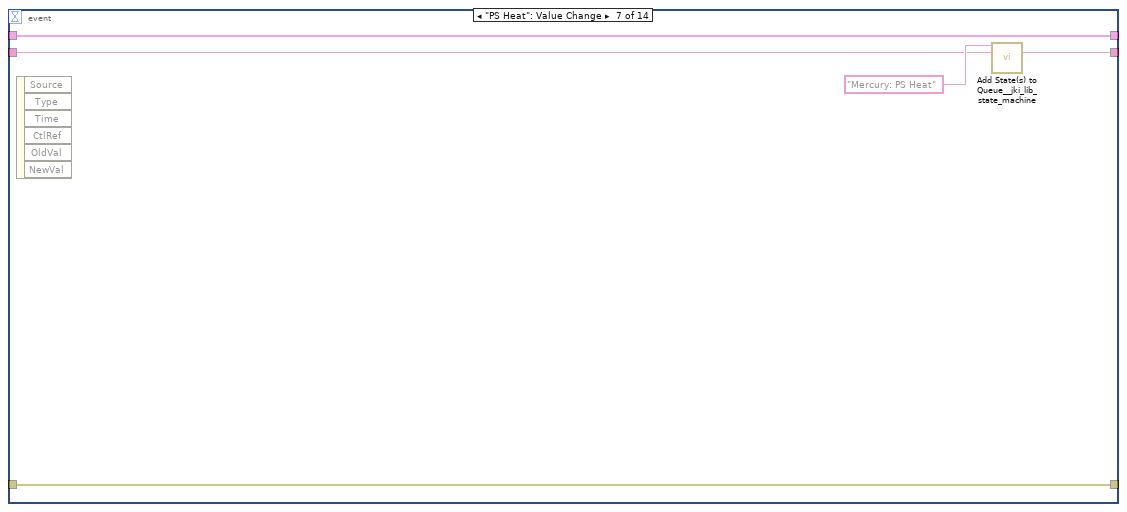
[diagram p8: hidden frame]
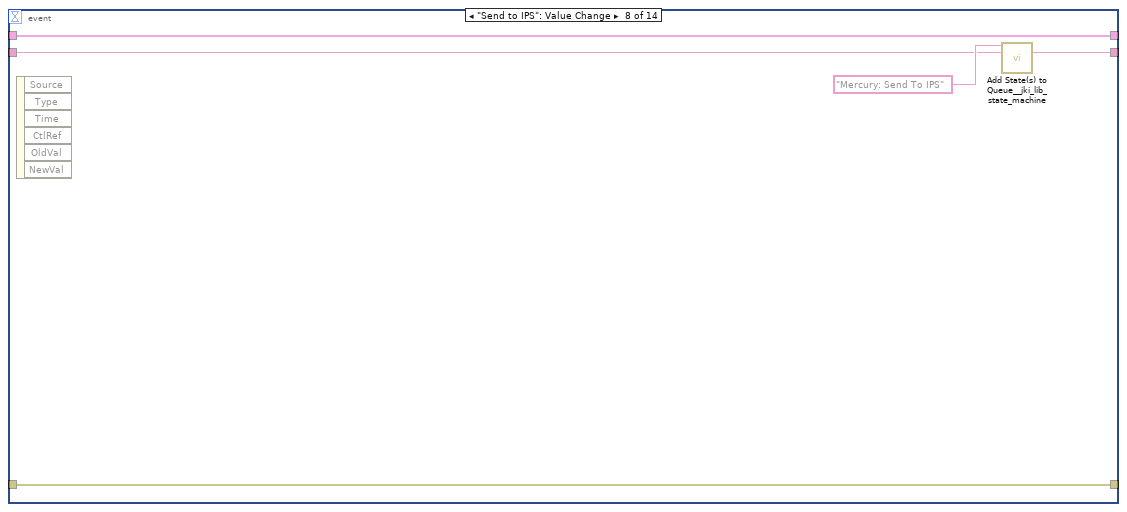
[diagram p9: hidden frame]
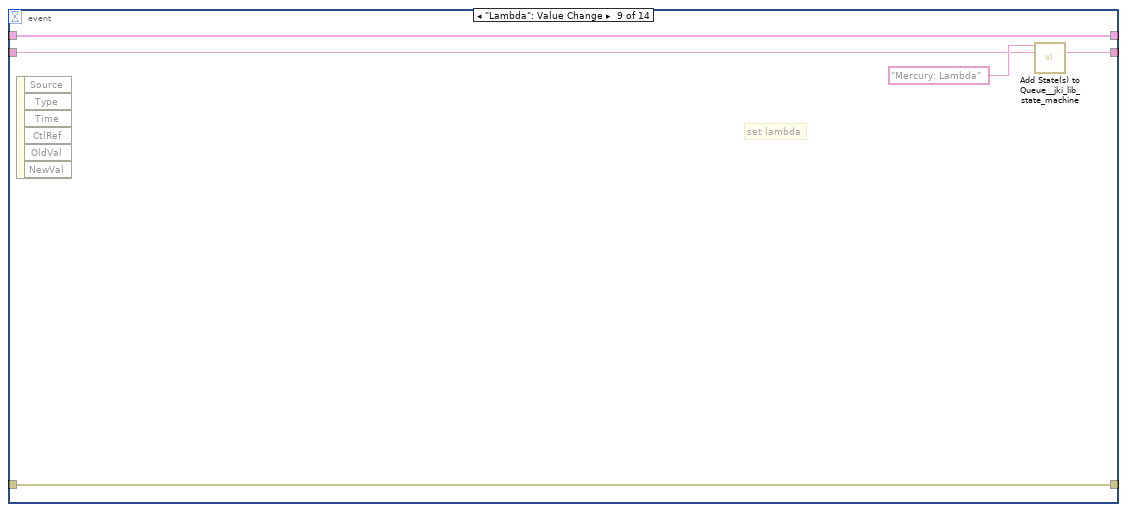
[diagram p10: hidden frame]
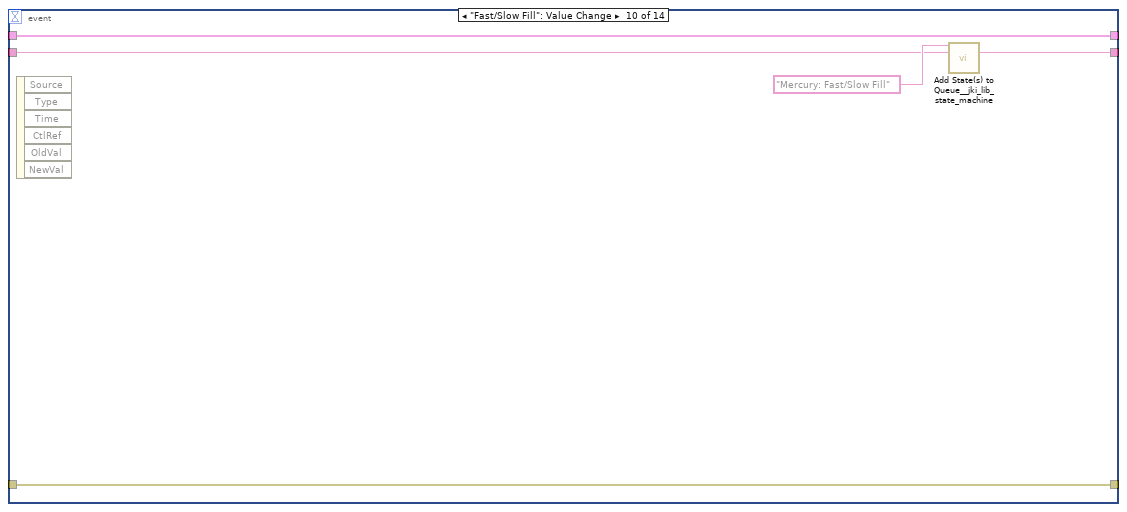
[diagram p11: hidden frame]
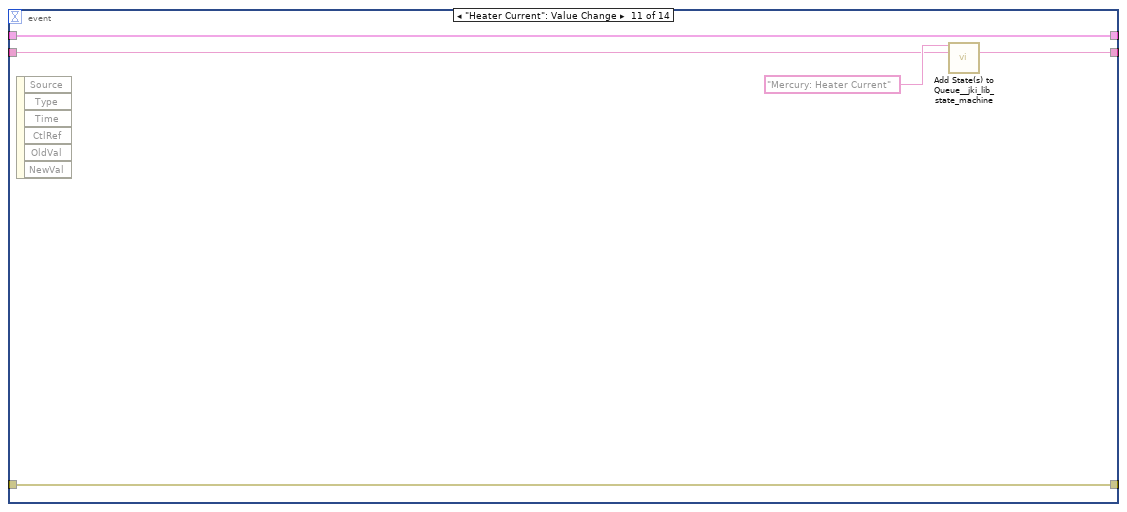
[diagram p12: hidden frame]
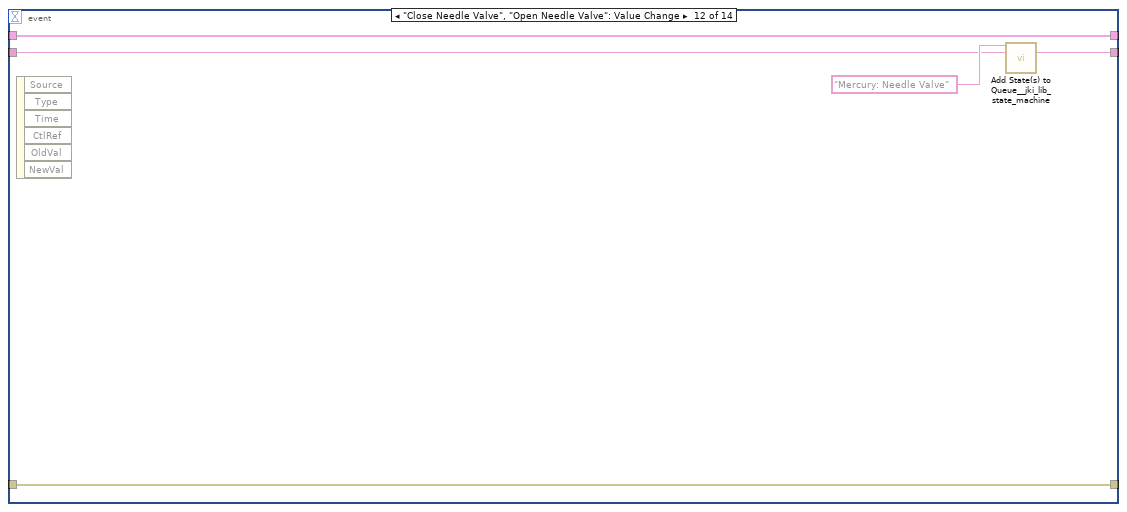
[diagram p13: hidden frame]
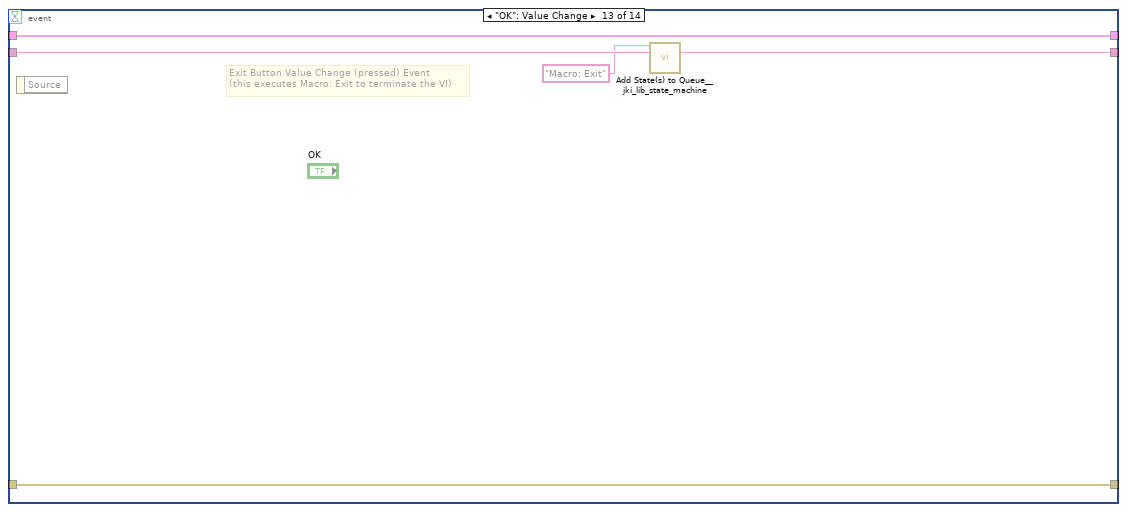
[diagram p14: hidden frame]
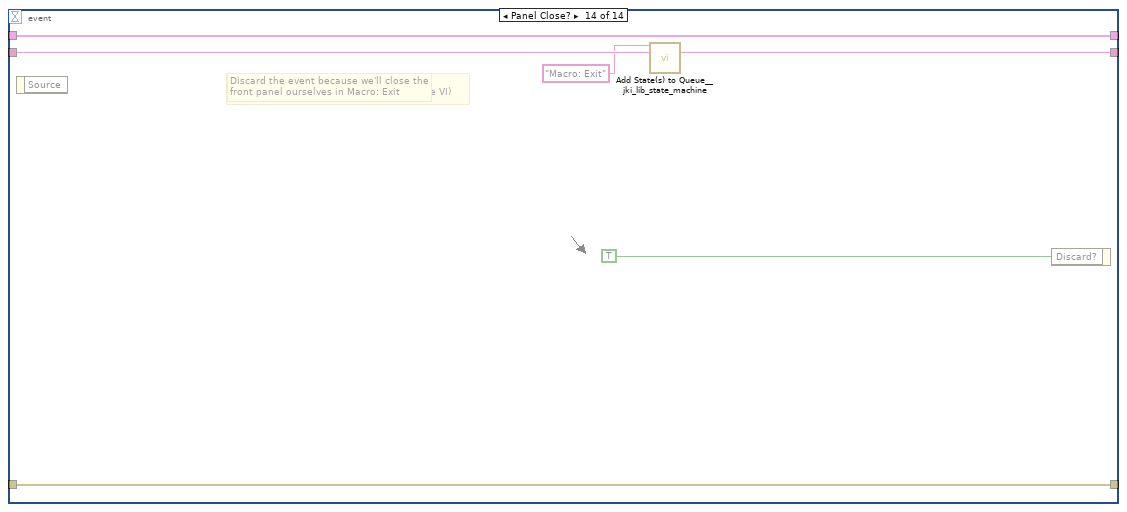
[diagram p15: hidden frame]
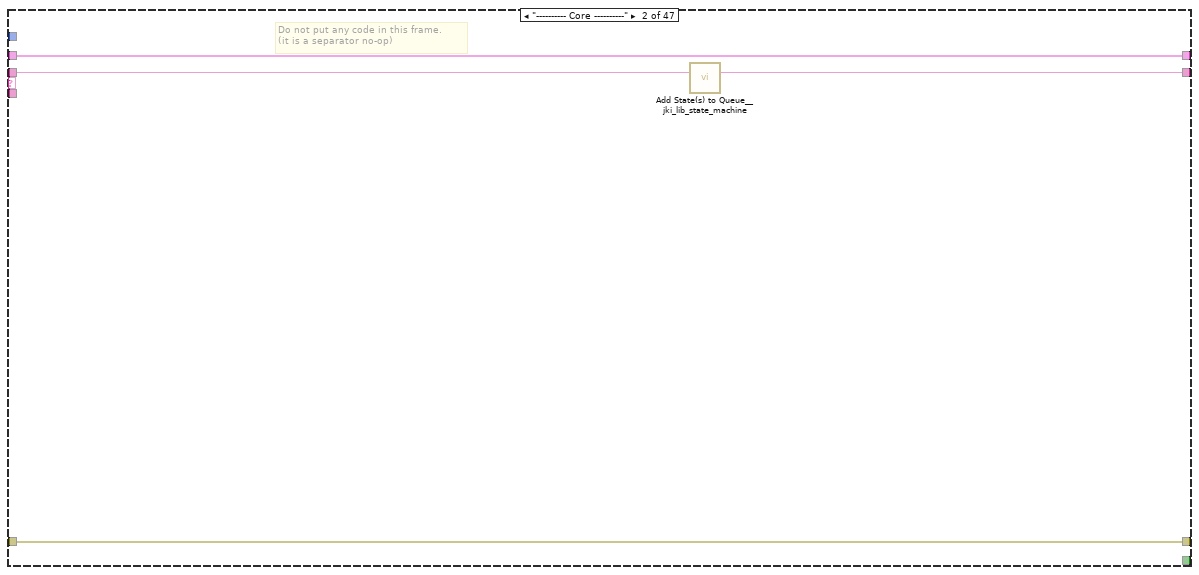
[diagram p16: hidden frame]
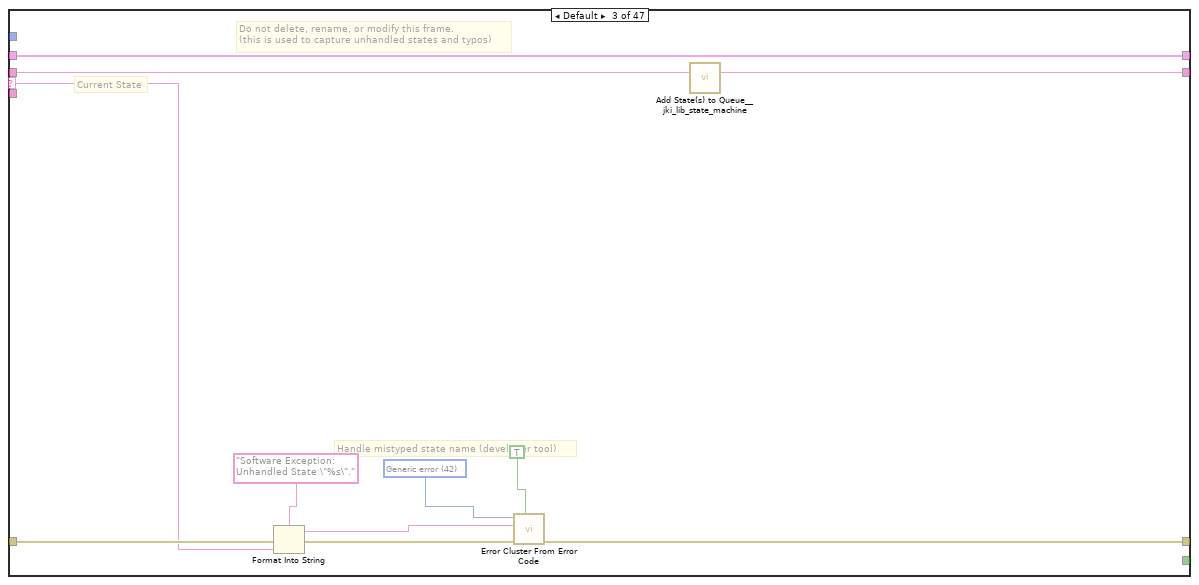
[diagram p17: hidden frame]
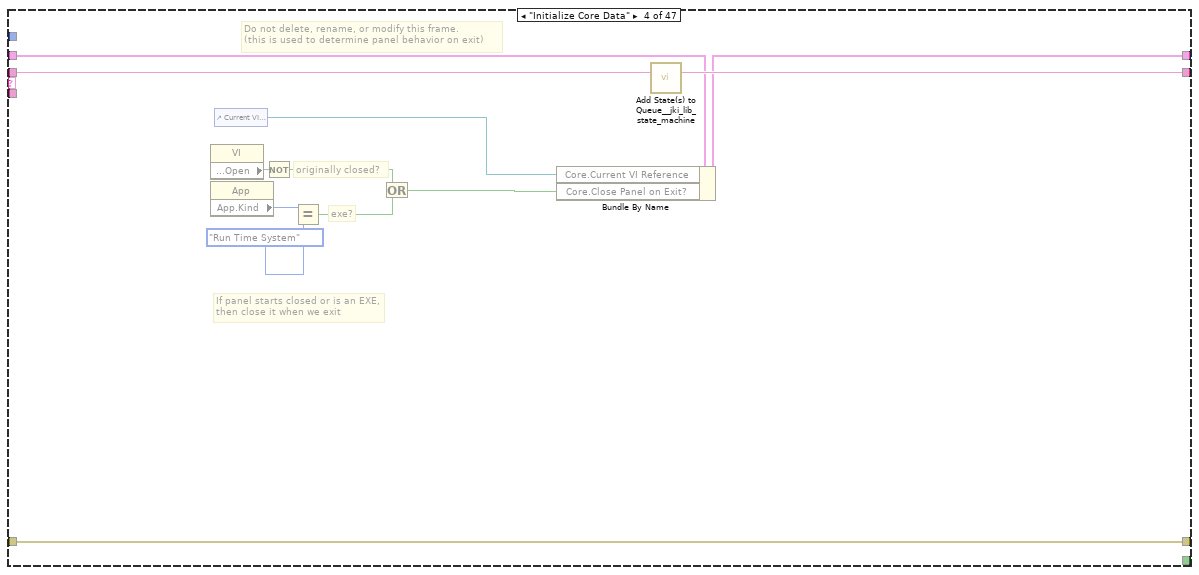
[diagram p18: hidden frame]
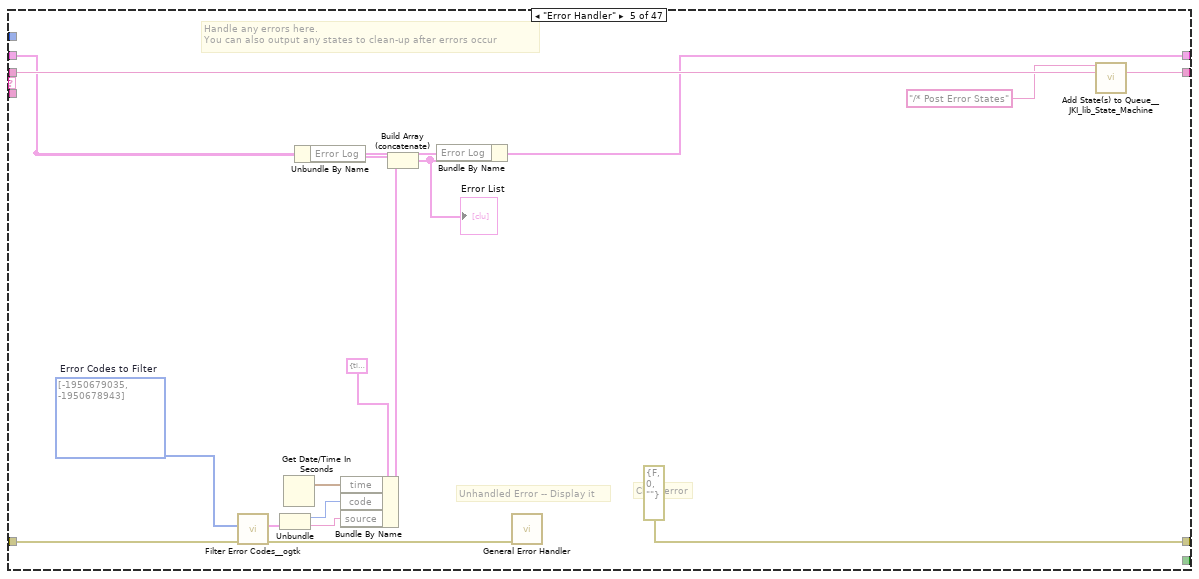
[diagram p19: hidden frame]
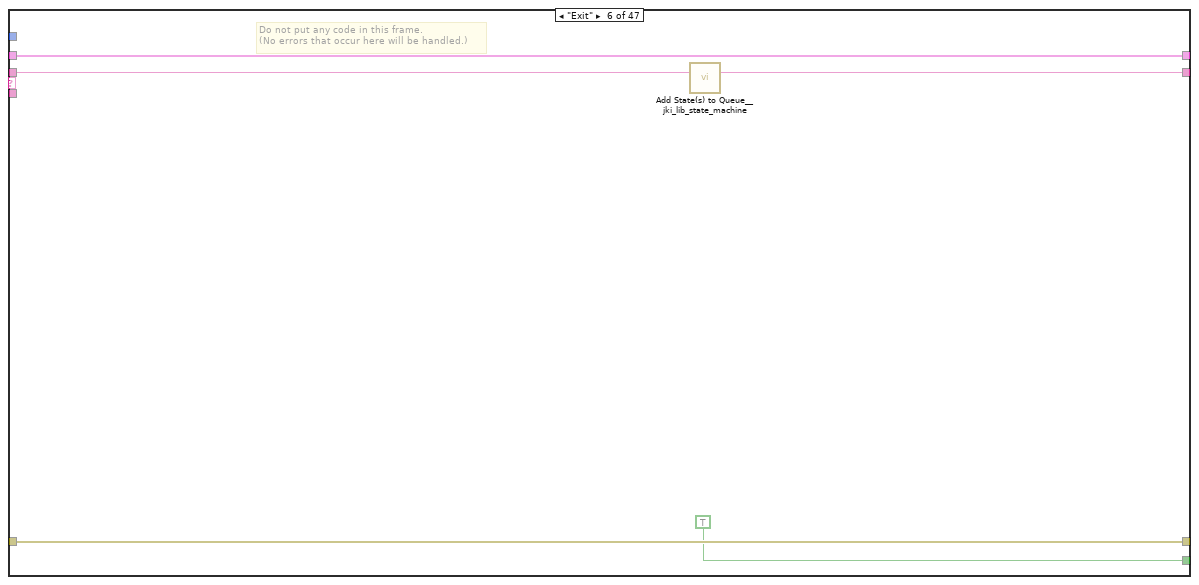
[diagram p20: hidden frame]
diagram:
  n1 = disable-structure shown="Disabled" {
    frame Disabled {
      # "copy \"Example - Basic IPS-SA.vi\"\nValue (signaling) will execute event if value changes\nUse FGVs to remotely interact with this? (like lockin 4461?)\nwrite values to DSC. Which ones?\nHow to interact with both ITC and IPS? There is problem with \nMercury reference dissapearing"
      # "For instructions on how to use the JKI State Machine, examples and video tutorials, visit:\nhttp://jki.net/state-machine/\n\nJKI State Machine™\nhttp://jki.net/state-machine/\nCopyright (C) 2005-2015, JKI <info@jki.net>\nALL RIGHTS RESERVED"
      # "State Syntax:\nStateCategory: State >> Argument\nLine Terminator: Line feed\nExample:\nUI: Help >> About\n\nWhere \"UI\" is the state category\nWhere \"Help\" is the state\nWhere \"About\" is the argument\nOther Examples:\nApp Data: Initialize\nUI: Initialize\nHelp >> About\n\nCommenting:\nTo add a comment use \"//\" or \"#\" and all text to the right will be ignored\nCommenting Example:\nUI: Initialize // This initializes the UI\n# This whole line is a comment\n// Another comment line"
      # "copy this to create labels for wires"
      # "System_Label"
      n2 = call <vilib>:"Add State(s) to Queue__jki_lib_state_machine.vi"("State(s) in (\"\")"="Macro: Initialize") -> ("States Out"=w2:string)  [unwired: 14 in]
      n3 = while "JKI - String-Based Queued State Machine (Basic) v1.0" {
        shift-right: [w6] -> _
        shift-left: _ -> [w5]
        shift-right: [w9] -> _
        shift-left: _ -> [w3]
        shift-right: [w8] -> _
        shift-left: w2 -> [w10]
        stop <- w7 stop-if-true
        w4 = 10  # Timeout
        # "Template Copyright © 2015 JKI - http://jki.net/state-machine"
        n4 = call <vilib>:"Parse State Queue__jki_lib_state_machine.vi"("State Queue"=w10, "Error In (no error)"=w3) -> ("Remaining States"=w12:string, "Current State"=w13:string, "Arguments"=w11:string)  [unwired: 11 in]
        n5 = case shown="\"\", \"Event Structure\", \"Idle\"" w13 {
          selector: w13 -> [_ _ w115 _ _ _ _ _ _ _ _ _ _ _ _ _ _ _ _ _ _ _ _ _ _ _ _ _ _ _ _ _ _ _ _ _ _ _ _ _ _ _ _ _ _ _ _]
          tunnel: w12 -> [w20 w114 w119 w137 w154 w159 w163 w176 w182 w186 w196 w206 w217 w243 w250 w265 w269 w293 w342 w388 w430 w477 w500 w545 w586 w633 w674 w679 w701 w767 w804 w862 w878 w905 w909 w914 w957 w990 w1022 w1041 w1060 w1079 w1101 w1169 w1190 w1211 w1229]
          tunnel: w11 -> [_ _ _ _ _ _ _ _ _ _ _ w201 w211 _ _ _ _ _ _ _ _ _ _ _ _ _ _ _ _ _ _ _ _ _ _ _ _ _ _ _ _ _ _ _ _ _ _]
          tunnel: w5 -> [w16 w111 w117 w128 w140 w157 w160 _ w177 w183 w187 w204 w213 w240 w248 w263 w266 w288 w340 w387 w394 w437 w486 w543 w585 w632 w673 w676 w683 w735 w803 w819 w877 w904 w908 w911 w955 w980 w1017 w1031 w1050 w1069 w1087 w1154 w1180 w1196 w1217]
          tunnel: [w14 w112 w121 w134 errorcluster {"status"=FALSE, "code"=0, "source"=""} ("error out") w156 w161 w170 w178 w184 w191 w202 w214 w241 w247 w253 w267 w271 w302 w343 w391 w440 w487 w507 w552 w605 w640 w677 w686 w736 w775 w815 w875 w889 w907 w912 w923 w974 w999 w1026 w1044 w1063 w1088 w1147 w1174 w1198 w1216] -> w9
          tunnel: [w19 w113 w118 w136 w153 w158 w162 w175 w181 w185 w195 w205 w216 w242 w249 w264 w268 w292 w341 w389 w431 w478 w501 w544 w587 w634 w675 w678 w702 w768 w805 w863 w879 w906 w910 w913 w958 w991 w1023 w1042 w1061 w1080 w1102 w1170 w1191 w1212 w1230] -> w8
          tunnel: [_ _ _ _ _ TRUE _ _ _ _ _ _ _ _ _ _ _ _ _ _ _ _ _ _ _ _ _ _ _ _ _ _ _ _ _ _ _ _ _ _ _ _ _ _ _ _ _] -> w7
          tunnel: [w18 w111 w117 w135 w139 w157 w160 w174 w177 w183 w188 w204 w213 w240 w248 w263 w266 w287 w340 w387 w394 w437 w486 w543 w585 w632 w673 w676 w682 w735 w803 w819 w877 w904 w908 w911 w955 w980 w1017 w1031 w1050 w1069 w1087 w1154 w1180 w1196 w1217] -> w6
          tunnel: w4 -> [w17 _ _ _ _ _ _ _ _ _ _ _ _ _ _ _ _ _ _ _ _ _ _ _ _ _ _ _ _ _ _ _ _ _ _ _ _ _ _ _ _ _ _ _ _ _ _]
          tunnel: w3 -> [w15 w112 w120 w134 w149 w156 w161 w170 w179 w184 w193 w203 w215 w241 w247 w255 w267 w280 w304 w354 w397 w439 w481 w509 w554 w592 w635 w677 w698 w766 w801 w852 w876 w883 w907 w912 w952 w985 w1014 w1036 w1055 w1074 w1089 w1164 w1181 w1199 w1215]
          frame "", "Event Structure", "Idle" {
            # "executes when the state queue is empty"
            n6 = event shown="[0] Timeout" {
              selector: _ -> [_ _ _ _ _ _ _ _ _ _ _ _ _ _]
              dyn-events: _ -> [_ _ _ _ _ _ _ _ _ _ _ _ _ _]
              timeout: w17 -> [_ _ _ _ _ _ _ _ _ _ _ _ _ _]
              tunnel: w20 -> [w38 w48 w54 w59 w63 w68 w73 w77 w83 w87 w92 w96 w104 w110]
              tunnel: [w37 w47 w53 w58 w62 w67 w72 w76 w82 w86 w91 w95 w103 w109] -> w19
              tunnel: [w21 w46 w50 w55 w60 w65 w70 w75 w80 w89 w94 w99 w101 w107] -> w18
              tunnel: w16 -> [w21 w46 w50 w55 w60 w65 w70 w75 w80 w89 w94 w99 w101 w107]
              tunnel: w15 -> [w24 w45 w51 w57 w64 w66 w71 w79 w81 w85 w90 w98 w102 w108]
              tunnel: [w23 w45 w51 w57 w64 w66 w71 w79 w81 w85 w90 w98 w102 w108] -> w14
              event Timeout {
                # "get remote"
                n7 = event-data() -> ()  [unwired: 1 in, 1 out]
                n8 = call "FGV_PSP - Mercury Remote.vi"("error in"=w24, "Function"=enum16{"write", "read"}."read") -> ("error out"=w23:errorcluster, "Remote"=w22:bool)  [unwired: 4 in]
                n9 = local write "Remote Mode"(w22) -> ()
                n10 = case shown="True" w22 {
                  tunnel: ["Mercury: Idle\nMercury: IPS: Idle - 1\nMercury: IPS: Idle - 1a\nMercury: IPS: Idle - 2\nMercury: IPS: Idle - 3\nMercury: ITC: Idle" ("State(s) at Back (\"\")") "Mercury: Remote\nMercury: Idle\nMercury: IPS: Idle - 1\nMercury: IPS: Idle - 1a\nMercury: IPS: Idle - 2\nMercury: IPS: Idle - 3\nMercury: ITC: Idle\n" ("State(s) at Back (\"\")")] -> w27
                  frame False {
                  }
                  frame True {
                  }
                }
                n11 = while {
                  shift-right: [w41] -> _
                  shift-left: _ -> [w42]
                  stop <- TRUE stop-if-true
                  n12 = Get Date/Time In Seconds() -> (seconds since 1Jan1904=w41:timestamp)
                  n13 = Subtract(x=w41, y=w42) -> (x-y=→"Iteration Time":dbl)
                }
                n14 = local read "Magnet Field (T)"() -> (w34:dbl)
                n15 = local read "Target Field (T)"() -> (w33:dbl)
                n16 = local read "Target Field Rate (T/min)"() -> (w36:dbl)
                n17 = local read "Power Supply Field (T)"() -> (w32:dbl)
                n18 = local read "SWITCH HEATER"() -> ()  [unwired: 1 out]
                n19 = local read "PS ON/OFF"() -> (w29:timestamp)
                n20 = local read "LPF ON"() -> (w31:timestamp)
                n21 = local read "Lambda"() -> (w26:bool)
                n22 = call "1820 Sweep ETA.vi"("Power Supply Field (T)"=w32, "Target Field Rate (T/min)"=w36, "Magnet Field (T)"=w34, "Target Field (T)"=w33) -> ("ETA timestamp"=→"ETA":timestamp)  [unwired: 5 in, 2 out]
                n23 = call "1820 PS Heat duration.vi"("time stamp"=w29) -> ("PS Heat on (HH:MM:SS)"=→"PS Heat on or off (sec)":dbl)
                n24 = call "1820 LPF ON duration.vi"("Lambda"=w26, "LPF ON"=w31) -> ("LPF on (HH:MM:SS)"=→"LPF on (min)":dbl)  [unwired: 9 in]
                n25 = call <vilib>:"Add State(s) to Queue__jki_lib_state_machine.vi"("State(s) in Front (\"\")"=w27, "State(s) in (\"\")"=w38) -> ("States Out"=w37:string)  [unwired: 13 in]
              }
              event "Remote Mode": Value Change {
                n26 = event-data() -> ()  [unwired: 1 in, 6 out]
                n27 = call <vilib>:"Add State(s) to Queue__jki_lib_state_machine.vi"("State(s) in Front (\"\")"="Mercury: Remote", "State(s) in (\"\")"=w48) -> ("States Out"=w47:string)  [unwired: 13 in]
              }
              event "Hold": Value Change {
                n28 = event-data() -> ()  [unwired: 1 in, 6 out]
                n29 = call <vilib>:"Add State(s) to Queue__jki_lib_state_machine.vi"("State(s) in Front (\"\")"="Mercury: Hold" ("State(s) in Front (\"\")"), "State(s) in (\"\")"=w54) -> ("States Out"=w53:string)  [unwired: 13 in]
              }
              event "Clamp": Value Change {
                n30 = event-data() -> ()  [unwired: 1 in, 6 out]
                n31 = call <vilib>:"Add State(s) to Queue__jki_lib_state_machine.vi"("State(s) in Front (\"\")"="Mercury: Clamp" ("State(s) in Front (\"\")"), "State(s) in (\"\")"=w59) -> ("States Out"=w58:string)  [unwired: 13 in]
              }
              event "To Set": Value Change {
                n32 = event-data() -> ()  [unwired: 1 in, 6 out]
                n33 = call <vilib>:"Add State(s) to Queue__jki_lib_state_machine.vi"("State(s) in Front (\"\")"="Mercury: To Set" ("State(s) in Front (\"\")"), "State(s) in (\"\")"=w63) -> ("States Out"=w62:string)  [unwired: 13 in]
              }
              event "To Zero": Value Change {
                n34 = event-data() -> ()  [unwired: 1 in, 6 out]
                n35 = call <vilib>:"Add State(s) to Queue__jki_lib_state_machine.vi"("State(s) in Front (\"\")"="Mercury: To Zero" ("State(s) in Front (\"\")"), "State(s) in (\"\")"=w68) -> ("States Out"=w67:string)  [unwired: 13 in]
              }
              event "PS Heat": Value Change {
                n36 = event-data() -> ()  [unwired: 1 in, 6 out]
                n37 = call <vilib>:"Add State(s) to Queue__jki_lib_state_machine.vi"("State(s) in Front (\"\")"="Mercury: PS Heat" ("State(s) in Front (\"\")"), "State(s) in (\"\")"=w73) -> ("States Out"=w72:string)  [unwired: 13 in]
              }
              event "Send to IPS": Value Change {
                n38 = event-data() -> ()  [unwired: 1 in, 6 out]
                n39 = call <vilib>:"Add State(s) to Queue__jki_lib_state_machine.vi"("State(s) in Front (\"\")"="Mercury: Send To IPS" ("State(s) in Front (\"\")"), "State(s) in (\"\")"=w77) -> ("States Out"=w76:string)  [unwired: 13 in]
              }
              event "Lambda": Value Change {
                # "set lambda"
                n40 = event-data() -> ()  [unwired: 1 in, 6 out]
                n41 = call <vilib>:"Add State(s) to Queue__jki_lib_state_machine.vi"("State(s) in Front (\"\")"="Mercury: Lambda" ("State(s) in Front (\"\")"), "State(s) in (\"\")"=w83) -> ("States Out"=w82:string)  [unwired: 13 in]
              }
              event "Fast/Slow Fill": Value Change {
                n42 = event-data() -> ()  [unwired: 1 in, 6 out]
                n43 = call <vilib>:"Add State(s) to Queue__jki_lib_state_machine.vi"("State(s) in Front (\"\")"="Mercury: Fast/Slow Fill" ("State(s) in Front (\"\")"), "State(s) in (\"\")"=w87) -> ("States Out"=w86:string)  [unwired: 13 in]
              }
              event "Heater Current": Value Change {
                n44 = event-data() -> ()  [unwired: 1 in, 6 out]
                n45 = call <vilib>:"Add State(s) to Queue__jki_lib_state_machine.vi"("State(s) in Front (\"\")"="Mercury: Heater Current" ("State(s) in Front (\"\")"), "State(s) in (\"\")"=w92) -> ("States Out"=w91:string)  [unwired: 13 in]
              }
              event "Close Needle Valve", "Open Needle Valve": Value Change {
                n46 = event-data() -> ()  [unwired: 1 in, 6 out]
                n47 = call <vilib>:"Add State(s) to Queue__jki_lib_state_machine.vi"("State(s) in Front (\"\")"="Mercury: Needle Valve" ("State(s) in Front (\"\")"), "State(s) in (\"\")"=w96) -> ("States Out"=w95:string)  [unwired: 13 in]
              }
              event "OK": Value Change {
                # "Exit Button Value Change (pressed) Event\n(this executes Macro: Exit to terminate the VI)"
                n48 = event-data() -> ()  [unwired: 1 in, 1 out]
                n49 = call <vilib>:"Add State(s) to Queue__jki_lib_state_machine.vi"("State(s) in Front (\"\")"="Macro: Exit", "State(s) in (\"\")"=w104) -> ("States Out"=w103:string)  [unwired: 13 in]
              }
              event Panel Close? {
                # "Discard the event because we'll close the front panel ourselves in Macro: Exit"
                # "Close Panel button (pressed) Event\n(this executes Macro: Exit to terminate the VI)"
                n50 = event-data() -> ()  [unwired: 1 in, 1 out]
                n51 = call <vilib>:"Add State(s) to Queue__jki_lib_state_machine.vi"("State(s) in Front (\"\")"="Macro: Exit", "State(s) in (\"\")"=w110) -> ("States Out"=w109:string)  [unwired: 13 in]
                n52 = event-data("Discard?"=TRUE) -> ()  [unwired: 1 in, 1 out]
              }
            }
          }
          frame "---------- Core ----------" {
            # "Do not put any code in this frame.\n(it is a separator no-op)"
            n53 = call <vilib>:"Add State(s) to Queue__jki_lib_state_machine.vi"("State(s) in (\"\")"=w114) -> ("States Out"=w113:string)  [unwired: 14 in]
          }
          frame Default {
            w124 = 42 items=["No error", "Argument error", "Memory is full", "Out of zone", "End of file", "File already open", "Generic file I/O error", "File not found", "File permission error", "Disk is full", "Duplicate path", "Too many files open", "System feature not enabled", "Resource file not found", "Cannot add resource", "Resource not found", "Image not found", "Image memory error", "Pen does not exist", "Config type invalid", "Config token not found", "Config parse error", "Config memory error", "Bad external code format", "Bad external code offset", "External code not present", "Null window", "Destroy window error", "Null menu", "Print aborted", "Bad print record", "Print driver error", "Windows error during printing", "Memory error during printing", "Print dialog error", "Generic print error", "Invalid device refnum", "Device not found", "Device parameter error", "Device unit error", "Cannot open device", "Device call aborted", "Generic error", "Cancelled by user", "Object ID too low", "Object ID too high", "Object not in heap", "Unknown heap", "Unknown object (invalid DefProc)", "Unknown object (DefProc not in table)", "Message out of range", "Invalid (null) method", "Unknown message", "Manager call not supported", "Bad address", "Network operation in progress", "Network operation timed out", "Connection is busy", "Network attribute not supported", "Network error", "Address in use", "System out of memory", "Connection aborted", "Connection refused", "Not connected", "Already connected", "Connection closed", "Initialization error (interapplication manager)", "Bad occurrence", "Wait on unbound occurrence handler", "Occurrence queue overflow", "Datalog type conflict", "Unused", "Unrecognized type (interapplication manager)", "Memory corrupt", "Failed to make temporary DLL", "Old CIN version", "Drag socket not found", "Failed to load drop-object", "Failed to register OLE object", "Failed to release OLE object", "Format specifier type mismatch", "Unknown format specifier", "Too few format specifiers", "Too many format specifiers", "Scan failed", "Newer CIN version", "Error converting to variant", "Runtime menu error", "Password tampered", "Variant attribute not found", "Incompatible variant data type", "Event data is not available", "Event Store is not present", "Occurrence is not found", "Event Queue is not created", "Event info is not available", "Refnum passed is NULL", "Error retrieving Class GUID", "Error retrieving CoClass GUID", "Error retrieving TypeLib GUID.", "Bad built application magic bytes.", "Specific driver is different from the specific driver associated with the Logical Name.", "There is no session opened to the class driver.", "Max Error", "MAX - Error with config objects", "MAX - Error loading configuration", "MAX - Group not supported"]
            # "Current State"
            # "Do not delete, rename, or modify this frame.\n(this is used to capture unhandled states and typos)"
            # "Handle mistyped state name (developer tool)"
            n54 = Format Into String(format string="Software Exception: Unhandled State \"%s\"." ("message"), error in=w120, w115) -> (resulting string=w123:string, error out=w122:errorcluster)  [unwired: 1 in]
            n55 = call <vilib>:"Error Cluster From Error Code.vi"("show call chain? (False)"=TRUE, "error in (no error)"=w122, "error message (\"\")"=w123, "error code (0)"=w124) -> ("error out"=w121:errorcluster)  [unwired: 5 in]
            n56 = call <vilib>:"Add State(s) to Queue__jki_lib_state_machine.vi"("State(s) in (\"\")"=w119) -> ("States Out"=w118:string)  [unwired: 14 in]
          }
          frame "Initialize Core Data" {
            # "Do not delete, rename, or modify this frame.\n(this is used to determine panel behavior on exit)"
            # "originally closed?"
            # "exe?"
            # "If panel starts closed or is an EXE, then close it when we exit"
            n57 = property class="VI"() -> ("Front Panel.Open"=w133:bool)  [unwired: 2 in, 2 out]
            n58 = property class="App"() -> ("App.Kind"=w132:T26)  [unwired: 2 in, 2 out]
            n59 = control-ref of="Current VI Reference"() -> (w126:refnum<vi>)
            n60 = Not(x=w133) -> (.not. x?=w130:bool)
            n61 = Equal?(x=w132, y=T26."Run Time System" ("Application:Kind")) -> (x = y?=w129:bool)
            n62 = Or(x=w130, y=w129) -> (x .or. y?=w127:bool)
            n63 = Bundle By Name(cluster=w128, "Core.Current VI Reference"=w126, "Core.Close Panel on Exit?"=w127) -> (w135:T38)
            n64 = call <vilib>:"Add State(s) to Queue__jki_lib_state_machine.vi"("State(s) in (\"\")"=w137) -> ("States Out"=w136:string)  [unwired: 14 in]
          }
          frame "Error Handler" {
            w148 = i32[] [-1950679035, -1950678943]  # Error Codes to Filter
            # "Unhandled Error -- Display it"
            # "Handle any errors here.\nYou can also output any states to clean-up after errors occur"
            # "Clear error"
            n65 = call-poly <userlib>:"Filter Error Codes__ogtk.vi"("Error In"=w149, "Error Codes to Filter"=w148) -> ("Error Out"=w150:errorcluster, "Filtered Error Details"=w147:T39)  [unwired: 7 in, 1 out]
            n66 = Unbundle(w147) -> ("code"=w145:i32, "source"=w146:string)
            n67 = Get Date/Time In Seconds() -> (seconds since 1Jan1904=w144:timestamp)
            n68 = Unbundle By Name(w140) -> ("Error Log"=w142:T25)
            n69 = Bundle By Name(cluster=T27 {"time"=timestamp(0 s since 1904-01-01), "code"=0, "source"=""} ("output cluster"), "time"=w144, "code"=w145, "source"=w146) -> (w141:T27)
            n70 = Build Array (concatenate)(w142, w141) -> (w138:T25)
            "Error List" <- w138
            n71 = Bundle By Name(cluster=w140, "Error Log"=w138) -> (w139:T38)
            n72 = call <vilib>:"General Error Handler.vi"("error in (no error)"=w150) -> ()  [unwired: 10 in, 5 out]
            n73 = call <vilib>:"Add State(s) to Queue__JKI_lib_State_Machine.vi"("State(s) in Front (\"\")"="/* Post Error States", "State(s) in (\"\")"=w154) -> ("States Out"=w153:string)  [unwired: 13 in]
          }
          frame "Exit" {
            # "Do not put any code in this frame.\n(No errors that occur here will be handled.)"
            n74 = call <vilib>:"Add State(s) to Queue__jki_lib_state_machine.vi"("State(s) in (\"\")"=w159) -> ("States Out"=w158:string)  [unwired: 14 in]
          }
          frame "---------- Data ----------" {
            # "Do not put any code in this frame.\n(It is a separator no-op. You can make a copy of this frame to create a new Data frame)"
            n75 = call <vilib>:"Add State(s) to Queue__jki_lib_state_machine.vi"("State(s) in (\"\")"=w163) -> ("States Out"=w162:string)  [unwired: 14 in]
          }
          frame "Data: Initialize" {
            w164 = bool[] [FALSE, FALSE, FALSE, FALSE, FALSE, FALSE, FALSE, FALSE]  # LEDs
            w165 = 0  # counter
            w167 = TRUE  # read ITC T?
            w168 = T35 {"Comms"="", "Device ID"=[], "Comms Layer"=enum."Ethernet TCP/IP", "Command"="", "Query reference"=refnum}  # Mercury ITC Ref
            w169 = T25 []  # Error Log
            w171 = TRUE  # sentinel
            w172 = T35 {"Comms"="", "Device ID"=[], "Comms Layer"=enum."Ethernet TCP/IP", "Command"="", "Query reference"=refnum}  # Mercury IPS Ref
            w173 = T40 {"Current VI Reference"=refnum, "Close Panel on Exit?"=FALSE}  # Core
            # "read FGV in timeout"
            # "do not delete - used by framework"
            # "Data names and types of shift register data are defined by this bundle."
            # "Initialize the shift-register data, here.\n(data names are defined by what you wire into the bundle function)"
            n76 = call <vilib>:"Add State(s) to Queue__jki_lib_state_machine.vi"("State(s) in (\"\")"=w176) -> ("States Out"=w175:string)  [unwired: 14 in]
            n77 = call "1820 State History.vi"("initialize?"=TRUE) -> ()  [unwired: 9 in, 2 out]
            n78 = Bundle("Core"=w173, "Mercury ITC Ref"=w168, "Mercury IPS Ref"=w172, "sentinel"=w171, "Error Log"=w169, "read ITC T?"=w167, "counter"=w165, "LEDs"=w164) -> (w174:T38)  [unwired: 1 in]
          }
          frame "Data: Cleanup" {
            # "Cleanup any data and references, here.\n(this is called automatically, by the Macro: Exit)"
            n79 = Unbundle By Name(w177) -> ("Core.Current VI Reference"=w180:refnum<vi>)
            n80 = Close Reference(reference=w180, error in (no error)=w179) -> (error out=w178:errorcluster)
            n81 = call <vilib>:"Add State(s) to Queue__jki_lib_state_machine.vi"("State(s) in (\"\")"=w182) -> ("States Out"=w181:string)  [unwired: 14 in]
          }
          frame "---------- UI ----------" {
            # "Do not put any code in this frame.\n(It is a separator no-op. You can make a copy of this frame to create a new UI frame)"
            n82 = call <vilib>:"Add State(s) to Queue__jki_lib_state_machine.vi"("State(s) in (\"\")"=w186) -> ("States Out"=w185:string)  [unwired: 14 in]
          }
          frame "UI: Initialize" {
            w189 = bool[] [TRUE, FALSE, TRUE, FALSE, TRUE, FALSE, TRUE, FALSE] ("LEDs")
            w192 = FALSE
            # "start in local mode"
            # "Initialize the User Interface, here.\n(this is called automatically, by the Macro: Init)"
            n83 = disable-structure shown="Enabled" {
              frame Disabled {
                n84 = Open Application Reference() -> (0:w198:errorcluster, 3:w197:refnum<vi>)  [unwired: 4 in]
                n85 = Open VI Reference(vi path=path "") -> ()  [unwired: 5 in, 2 out]
                n86 = property class="App"(reference=w197, error in=w198, "WebSrvr.Active"=TRUE ("Web Server:Server Active")) -> ()  [unwired: 2 out]
                n87 = call "MNK_Dashboard_v2.vi"() -> ()  [unwired: 12 in]
              }
              frame Enabled {
              }
            }
            n88 = call <userlib>:"Fit VI window to Largest Dec__ogtk.vi"("error in (no error)"=w193) -> ("error out"=w190:errorcluster)  [unwired: 5 in, 1 out]
            n89 = local write "Remote Mode"(w192) -> ()
            n90 = call <vilib>:"Add State(s) to Queue__jki_lib_state_machine.vi"("State(s) in (\"\")"=w196) -> ("States Out"=w195:string)  [unwired: 14 in]
            n91 = call "FGV_PSP - Mercury Remote.vi"("error in"=w190, "Remote"=w192) -> ("error out"=w191:errorcluster)  [unwired: 4 in, 1 out]
            n92 = local write "LEDs"(w189) -> ()
            n93 = Bundle By Name(cluster=w187, "LEDs"=w189) -> (w188:T38)
            "Magnet Status 2" <- "" ("Magnet Status 2")
          }
          frame "UI: Cursor Set" {
            # "Argument"
            # "Set and Unset Cursor Busy.\n(Usage: \"UI: Cursor Set >> Busy|Idle\")"
            n94 = case shown="\"Idle\", Default" w201 {
              tunnel: w203 -> [w208 w210]
              tunnel: [w207 w209] -> w202
              frame "Idle", Default {
                n95 = call <vilib>:"Unset Busy.vi"("error in (no error)"=w208) -> ("error out"=w207:errorcluster)  [unwired: 10 in]
              }
              frame "Busy" {
                n96 = call <vilib>:"Set Busy.vi"("error in (no error)"=w210) -> ("error out"=w209:errorcluster)  [unwired: 9 in, 1 out]
              }
            }
            n97 = call <vilib>:"Add State(s) to Queue__JKI_lib_State_Machine.vi"("State(s) in (\"\")"=w206) -> ("States Out"=w205:string)  [unwired: 14 in]
          }
          frame "UI: Front Panel State" {
            # "Argument"
            # "Set Front Panel Open or Closed\n(Usage: \"UI: Front Panel State >> Open|Close\")"
            n98 = Unbundle By Name(w213) -> ("Core.Current VI Reference"=w212:refnum<vi>)
            n99 = case shown="\"Open\", Default" w211 {
              tunnel: w215 -> [w221 w234]
              tunnel: [w223 w235] -> w214
              tunnel: w212 -> [w222 w232]
              frame "Open", Default {
                n100 = property class="VI"(reference=w222, error in=w221) -> (reference out=w219:refnum<vi>, error out=w220:errorcluster, "Front Panel.Open"=w218:bool)
                n101 = case shown="True" w218 {
                  tunnel: [w226 w229] -> w223
                  tunnel: w220 -> [w225 w229]
                  tunnel: w219 -> [w224 _]
                  frame False {
                    n102 = invoke class="VI" method="FP.Open"(reference=w224, error in=w225, "Activate"=TRUE, "State"=T28."Standard") -> (error out=w226:errorcluster)  [unwired: 1 in, 4 out]
                  }
                  frame True {
                  }
                }
              }
              frame "Close" {
                n103 = property class="VI"(reference=w232, error in=w234) -> (reference out=w231:refnum<vi>, error out=w233:errorcluster, "Front Panel.Open"=w230:bool)
                n104 = case shown="True" w230 {
                  tunnel: [w236 w239] -> w235
                  tunnel: w233 -> [w236 w238]
                  tunnel: w231 -> [_ w237]
                  frame False {
                  }
                  frame True {
                    n105 = invoke class="VI" method="FP.Close"(reference=w237, error in=w238) -> (error out=w239:errorcluster)  [unwired: 1 in, 2 out]
                  }
                }
              }
            }
            n106 = call <vilib>:"Add State(s) to Queue__JKI_lib_State_Machine.vi"("State(s) in (\"\")"=w217) -> ("States Out"=w216:string)  [unwired: 14 in]
          }
          frame "---------- Macro ----------" {
            # "Do not put any code in this frame.\n(It is a separator no-op. You can make a copy of this frame to create a new Macro frame)"
            n107 = call <vilib>:"Add State(s) to Queue__JKI_lib_State_Machine.vi"("State(s) in (\"\")"=w243) -> ("States Out"=w242:string)  [unwired: 14 in]
          }
          frame "Macro: Initialize" {
            w246 = "Data: Initialize\nInitialize Core Data\nUI: Initialize\nUI: Front Panel State >> Open"  # Data: Initialize Initialize Core Data UI: Initialize UI: Front Panel State >> Open
            # "Initialization Macro\n(This is called once, when the VI starts)"
            n108 = call <vilib>:"Add State(s) to Queue__JKI_lib_State_Machine.vi"("State(s) in Front (\"\")"=w246, "State(s) at Back (\"\")"="Mercury: Initialize") -> ("States Out"=w245:string)  [unwired: 13 in]
            n109 = call <vilib>:"Add State(s) to Queue__JKI_lib_State_Machine.vi"("State(s) in Front (\"\")"=w245, "State(s) in (\"\")"=w250) -> ("States Out"=w249:string)  [unwired: 13 in]
          }
          frame "Macro: Exit" {
            # "#Implemented in Close Instrument.vi"
            # "Exit Macro\n(This is called once, when the VI exits)"
            n110 = Unbundle By Name(w263) -> ("Core.Close Panel on Exit?"=w262:bool, "Mercury ITC Ref"=w251:T35, "Mercury IPS Ref"=w252:T35)
            n111 = call <instrlib>:"Close.vi"("error in (no error)"=w255, "Mercury Reference"=w252) -> ("error out"=w254:errorcluster)  [unwired: 9 out]
            n112 = call <instrlib>:"Close.vi"("error in (no error)"=w254, "Mercury Reference"=w251) -> ("error out"=w256:errorcluster)  [unwired: 9 out]
            n113 = call <vilib>:"Simple Error Handler.vi"("error in (no error)"=w256) -> ("error out"=w253:errorcluster)  [unwired: 1 in, 7 out]
            n114 = Select(t="UI: Front Panel State >> Close", s=w262, f="") -> (s? t:f=w259:string)
            n115 = call <vilib>:"Add State(s) to Queue__JKI_lib_State_Machine.vi"("State(s) in (\"\")"=w259, "State(s) at Back (\"\")"="Data: Cleanup\nExit") -> ("States Out"=w257:string)  [unwired: 13 in]
            n116 = call <vilib>:"Add State(s) to Queue__JKI_lib_State_Machine.vi"("State(s) in Front (\"\")"=w257, "State(s) in (\"\")"=w265) -> ("States Out"=w264:string)  [unwired: 13 in]
          }
          frame "---------- Mercury: Query ----------" {
            n117 = call <vilib>:"Add State(s) to Queue__JKI_lib_State_Machine.vi"("State(s) in (\"\")"=w269) -> ("States Out"=w268:string)  [unwired: 14 in]
          }
          frame "Mercury: Initialize" {
            w279 = Comms_Transport_Layer."Ethernet TCP/IP" ("Comms Layer")
            # "#Implemented in Open Instrument.vi"
            n118 = call-poly <instrlib>:"Open.vi"("Clear Previous Connections (False)"=TRUE ("Clear Previous Connections (True)"), "ID Query (True)"=TRUE, "IP Address"="ITC IP Address", "error in (no error)"=w280, "Comms Layer"=w279) -> ("error out"=w274:errorcluster, "# of Instruments"=→"# of Instruments":i32, "Serial Number(s)"=→"Serial Number(s)":string[], "Mercury Reference Out"=w275:T35, "S/W Version(s)"=→"S/W Version(s)":string[])  [unwired: 2 in]
            n119 = call-poly <instrlib>:"Open.vi"("Clear Previous Connections (False)"=FALSE ("Clear Previous Connections (True)"), "ID Query (True)"=TRUE, "IP Address"="IPS IP Address", "error in (no error)"=w274, "Comms Layer"=w279) -> ("error out"=w271:errorcluster, "# of Instruments"=→"# of Instruments 2":i32, "Serial Number(s)"=→"Serial Number(s) 2":string[], "Mercury Reference Out"=w273:T35, "S/W Version(s)"=→"S/W Version(s) 2":string[])  [unwired: 2 in]
            n120 = case shown="No Error" w271 {
              tunnel: ["Mercury: Query ITC: System\nMercury: Query IPS: System\nMercury: Query ITC: Temperature\nMercury: Query ITC: Heater\nMercury: Query ITC: Aux\nMercury: Query ITC: Pressure\nMercury: Query IPS: LVL\nMercury: Query IPS: Temperature\nMercury: Query IPS: Magnet" ("State(s) at Back (\"\")") "Error Handler\nMacro: Exit" ("State(s) at Back (\"\")")] -> w272
              tunnel: [bool[] [TRUE, FALSE, TRUE, FALSE, TRUE, FALSE, TRUE, FALSE] ("LEDs") w297] -> w270
              frame No Error {
                n121 = local write "LEDs"(bool[] [TRUE, TRUE, TRUE, TRUE, TRUE, TRUE, TRUE, TRUE] ("LEDs")) -> ()
              }
              frame Error {
                w297 = bool[] [FALSE, FALSE, FALSE, FALSE, FALSE, FALSE, FALSE, FALSE] ("LEDs")
                n122 = local write "LEDs"(w297) -> ()
              }
            }
            n123 = Bundle By Name(cluster=w288, "Mercury ITC Ref"=w275, "Mercury IPS Ref"=w273, "LEDs"=w270) -> (w287:T38)
            n124 = call <vilib>:"Add State(s) to Queue__JKI_lib_State_Machine.vi"("State(s) in Front (\"\")"=w272, "State(s) in (\"\")"=w293) -> ("States Out"=w292:string)  [unwired: 13 in]
          }
          frame "Mercury: Query ITC: System" {
            n125 = Unbundle By Name(w340) -> ("Mercury ITC Ref"=w300:T35)
            n126 = call-poly <instrlib>:"Configuration (Read).vi"("error in"=w304, "Mercury Reference In"=w300) -> ("error out"=w336:errorcluster, "Devices"=→"ITC Devices":string[], "Mercury Reference Out"=w337:T35)  [unwired: 1 in, 6 out]
            n127 = call-poly <instrlib>:"Configuration (Read).vi"("error in"=w336, "Mercury Reference In"=w337) -> ("error out"=w329:errorcluster, "Automatic Dimming"=→"Automatic Dimming":string, "Mercury Reference Out"=w330:T35)  [unwired: 1 in, 6 out]
            n128 = call-poly <instrlib>:"Configuration (Read).vi"("error in"=w329, "Mercury Reference In"=w330) -> ("error out"=w332:errorcluster, "Dimming Time"=→"Dimming Time":string, "Mercury Reference Out"=w331:T35)  [unwired: 1 in, 6 out]
            n129 = call-poly <instrlib>:"Configuration (Read).vi"("error in"=w332, "Mercury Reference In"=w331) -> ("error out"=w338:errorcluster, "Display Brightness"=→"Display Brightness":string, "Mercury Reference Out"=w339:T35)  [unwired: 1 in, 6 out]
            n130 = call-poly <instrlib>:"Configuration (Read).vi"("error in"=w338, "Mercury Reference In"=w339) -> ("error out"=w323:errorcluster, "Date"=→"Date":string, "Mercury Reference Out"=w322:T35)  [unwired: 1 in, 6 out]
            n131 = call-poly <instrlib>:"Configuration (Read).vi"("error in"=w323, "Mercury Reference In"=w322) -> ("error out"=w325:errorcluster, "Time"=→"Time":string, "Mercury Reference Out"=w324:T35)  [unwired: 1 in, 6 out]
            n132 = call-poly <instrlib>:"Configuration (Read).vi"("error in"=w325, "Mercury Reference In"=w324) -> ("error out"=w303:errorcluster, "time stamp"=→"time stamp":timestamp, "Mercury Reference Out"=w301:T35)  [unwired: 1 in, 6 out]
            n133 = call-poly <instrlib>:"Configuration (Read).vi"("error in"=w303, "Mercury Reference In"=w301) -> ("error out"=w321:errorcluster, "Hardware Version"=→"Hardware Version":string, "Mercury Reference Out"=w320:T35)  [unwired: 1 in, 6 out]
            n134 = call-poly <instrlib>:"Configuration (Read).vi"("error in"=w321, "Mercury Reference In"=w320) -> ("error out"=w319:errorcluster, "Firmware Version"=→"Firmware Version":string, "Mercury Reference Out"=w318:T35)  [unwired: 1 in, 6 out]
            n135 = call-poly <instrlib>:"Configuration (Read).vi"("error in"=w319, "Mercury Reference In"=w318) -> ("error out"=w306:errorcluster, "Serial Number"=→"Serial Number":string, "Mercury Reference Out"=w305:T35)  [unwired: 1 in, 6 out]
            n136 = call-poly <instrlib>:"Configuration (Read).vi"("error in"=w306, "Mercury Reference In"=w305) -> ("error out"=w312:errorcluster, "Free Space"=→"Free Space":i32, "Mercury Reference Out"=w311:T35)  [unwired: 1 in, 6 out]
            n137 = call-poly <instrlib>:"Configuration (Read).vi"("error in"=w312, "Mercury Reference In"=w311) -> ("error out"=w308:errorcluster, "Mode"=→"String":T32, "Mercury Reference Out"=w309:T35)  [unwired: 1 in, 6 out]
            n138 = Get Date/Time In Seconds() -> (seconds since 1Jan1904=w317:timestamp)
            n139 = call-poly <instrlib>:"Configuration (Set).vi"("error in"=w308, "time stamp"=w317, "Mercury Reference In"=w309) -> ("error out"=w302:errorcluster, "Response"=→"Set Date Response":T34)  [unwired: 1 in, 6 out]
            n140 = call <vilib>:"Add State(s) to Queue__JKI_lib_State_Machine.vi"("State(s) in (\"\")"=w342) -> ("States Out"=w341:string)  [unwired: 14 in]
          }
          frame "Mercury: Query ITC: Temperature" {
            # "Temperature"
            n141 = Unbundle By Name(w387) -> ("Mercury ITC Ref"=w349:T35)
            n142 = local read "ITC Devices"() -> (w348:string[])
            n143 = Index Array(array=w348, index=3) -> (element=w350:string)
            n144 = call-poly <instrlib>:"Open.vi"("error in (no error)"=w354, "Device Identifier"=w350, "Mercury Reference In"=w349) -> ("error out"=w366:errorcluster, "Mercury Reference Out"=w367:T35)  [unwired: 7 out]
            n145 = call-poly <instrlib>:"Configuration (Read).vi"("error in"=w366, "Mercury Reference In"=w367) -> ("error out"=w358:errorcluster, "Serial Number"=→"Temp S/N":string, "Mercury Reference Out"=w357:T35)  [unwired: 1 in, 6 out]
            n146 = call-poly <instrlib>:"Configuration (Read).vi"("error in"=w358, "Mercury Reference In"=w357) -> ("error out"=w360:errorcluster, "Nickname"=→"T Nickname":string, "Mercury Reference Out"=w359:T35)  [unwired: 1 in, 6 out]
            n147 = call-poly <instrlib>:"Configuration (Read).vi"("error in"=w360, "Mercury Reference In"=w359) -> ("error out"=w363:errorcluster, "Unit"=→"Unit":T3, "Excitation Magnitude"=→"Excitation Magnitude":dbl, "Mercury Reference Out"=w362:T35)  [unwired: 1 in, 5 out]
            n148 = call-poly <instrlib>:"Configuration (Read).vi"("error in"=w363, "Mercury Reference In"=w362) -> ("error out"=w353:errorcluster, "Sensor Type"=→"Sensor Type":T41, "Mercury Reference Out"=w351:T35)  [unwired: 1 in, 6 out]
            n149 = call-poly <instrlib>:"Configuration (Read).vi"("error in"=w353, "Mercury Reference In"=w351) -> ("error out"=w369:errorcluster, "Excitation Type"=→"Excitation Type":T7, "Mercury Reference Out"=w370:T35)  [unwired: 1 in, 6 out]
            n150 = call-poly <instrlib>:"Configuration (Read).vi"("error in"=w369, "Mercury Reference In"=w370) -> ("error out"=w371:errorcluster, "Unit"=→"H Unit":T3, "Hot Limit"=→"Hot Limit":dbl, "Mercury Reference Out"=w372:T35)  [unwired: 1 in, 5 out]
            n151 = call-poly <instrlib>:"Configuration (Read).vi"("error in"=w371, "Mercury Reference In"=w372) -> ("error out"=w378:errorcluster, "Unit"=→"C Unit":T3, "Cold Limit"=→"Cold Limit":dbl, "Mercury Reference Out"=w377:T35)  [unwired: 1 in, 5 out]
            n152 = call-poly <instrlib>:"Signals (Read).vi"("error in"=w378, "Mercury Reference In"=w377) -> ("error out"=w382:errorcluster, "Unit"=→"V Unit":T3, "Voltage"=→"Voltage":dbl, "Mercury Reference Out"=w381:T35)  [unwired: 1 in, 5 out]
            n153 = call-poly <instrlib>:"Signals (Read).vi"("error in"=w382, "Mercury Reference In"=w381) -> ("error out"=w383:errorcluster, "Unit"=→"T Unit":T3, "Temperature"=→"Temperature":dbl, "Mercury Reference Out"=w386:T35)  [unwired: 1 in, 5 out]
            n154 = call-poly <instrlib>:"Configuration (Read).vi"("error in"=w383, "Mercury Reference In"=w386) -> ("error out"=w343:errorcluster, "Device Details"=w344:T42)  [unwired: 1 in, 7 out]
            n155 = Unbundle By Name(w344) -> ("Manufacturing"=→"ITC Manufacturing":T8, "Excitation"=→"ITC Excitation":T6, "Calibration"=→"ITC Calibration":T4)
            n156 = call <vilib>:"Add State(s) to Queue__JKI_lib_State_Machine.vi"("State(s) in (\"\")"=w388) -> ("States Out"=w389:string)  [unwired: 14 in]
          }
          frame "Mercury: Query ITC: Heater" {
            # "Heater"
            n157 = Unbundle By Name(w394) -> ("Mercury ITC Ref"=w393:T35)
            n158 = local read "ITC Devices"() -> (w395:string[])
            n159 = Index Array(array=w395, index=2) -> (element=w390:string)
            n160 = call-poly <instrlib>:"Open.vi"("error in (no error)"=w397, "Device Identifier"=w390, "Mercury Reference In"=w393) -> ("error out"=w400:errorcluster, "Mercury Reference Out"=w399:T35)  [unwired: 7 out]
            n161 = call-poly <instrlib>:"Configuration (Read).vi"("error in"=w400, "Mercury Reference In"=w399) -> ("error out"=w407:errorcluster, "Device Details"=→"Heater Device Settings":T9, "Mercury Reference Out"=w406:T35)  [unwired: 1 in, 6 out]
            n162 = call-poly <instrlib>:"Configuration (Read).vi"("error in"=w407, "Mercury Reference In"=w406) -> ("error out"=w409:errorcluster, "Nickname"=→"Htr Nickname":string, "Mercury Reference Out"=w408:T35)  [unwired: 1 in, 6 out]
            n163 = call-poly <instrlib>:"Configuration (Read).vi"("error in"=w409, "Mercury Reference In"=w408) -> ("error out"=w402:errorcluster, "Serial Number"=→"Htr S/N":string, "Mercury Reference Out"=w401:T35)  [unwired: 1 in, 6 out]
            n164 = call-poly <instrlib>:"Configuration (Read).vi"("error in"=w402, "Mercury Reference In"=w401) -> ("error out"=w398:errorcluster, "Unit"=→"Volt Unit":T3, "Voltage Limit"=→"Htr Voltage Limit":dbl, "Mercury Reference Out"=w392:T35)  [unwired: 1 in, 5 out]
            n165 = call-poly <instrlib>:"Configuration (Read).vi"("error in"=w398, "Mercury Reference In"=w392) -> ("error out"=w412:errorcluster, "Unit"=→"Res Unit":T3, "Nominal Resistance"=→"Htr Resistance":dbl, "Mercury Reference Out"=w413:T35)  [unwired: 1 in, 5 out]
            n166 = call-poly <instrlib>:"Configuration (Read).vi"("error in"=w412, "Mercury Reference In"=w413) -> ("error out"=w419:errorcluster, "Unit"=→"Power Unit":T3, "Maximum Power"=→"Maximum Power":dbl, "Mercury Reference Out"=w418:T35)  [unwired: 1 in, 5 out]
            n167 = call-poly <instrlib>:"Signals (Read).vi"("error in"=w419, "Mercury Reference In"=w418) -> ("error out"=w421:errorcluster, "Unit"=→"Htr V Unit":T3, "Voltage"=→"Htr Voltage":dbl, "Mercury Reference Out"=w420:T35)  [unwired: 1 in, 5 out]
            n168 = call-poly <instrlib>:"Signals (Read).vi"("error in"=w421, "Mercury Reference In"=w420) -> ("error out"=w423:errorcluster, "Unit"=→"Htr P Unit":T3, "Power"=→"Htr Power":dbl, "Mercury Reference Out"=w422:T35)  [unwired: 1 in, 5 out]
            n169 = call-poly <instrlib>:"Signals (Read).vi"("error in"=w423, "Mercury Reference In"=w422) -> ("error out"=w391:errorcluster, "Unit"=→"Htr C Unit":T3, "Current"=→"Htr Current":dbl)  [unwired: 1 in, 6 out]
            n170 = call <vilib>:"Add State(s) to Queue__JKI_lib_State_Machine.vi"("State(s) in (\"\")"=w430) -> ("States Out"=w431:string)  [unwired: 14 in]
          }
          frame "Mercury: Query ITC: Aux" {
            # "Auxiliary"
            n171 = Unbundle By Name(w437) -> ("Mercury ITC Ref"=w432:T35)
            n172 = local read "ITC Devices"() -> (w435:string[])
            n173 = Index Array(array=w435, index=0) -> (element=w433:string)
            n174 = call-poly <instrlib>:"Open.vi"("error in (no error)"=w439, "Device Identifier"=w433, "Mercury Reference In"=w432) -> ("error out"=w459:errorcluster, "Mercury Reference Out"=w460:T35)  [unwired: 7 out]
            n175 = call-poly <instrlib>:"Configuration (Read).vi"("error in"=w459, "Mercury Reference In"=w460) -> ("error out"=w463:errorcluster, "Auxiliary Device Details"=→"Auxiliary Device Details":T12, "Mercury Reference Out"=w462:T35)  [unwired: 1 in, 6 out]
            n176 = call-poly <instrlib>:"Configuration (Read).vi"("error in"=w463, "Mercury Reference In"=w462) -> ("error out"=w466:errorcluster, "Serial Number"=→"Aux S/N":string, "Mercury Reference Out"=w465:T35)  [unwired: 1 in, 6 out]
            n177 = call-poly <instrlib>:"Configuration (Read).vi"("error in"=w466, "Mercury Reference In"=w465) -> ("error out"=w468:errorcluster, "Unit"=→"Unit 2":T3, "Min Flow"=→"Min Flow":dbl, "Mercury Reference Out"=w467:T35)  [unwired: 1 in, 5 out]
            n178 = call-poly <instrlib>:"Configuration (Read).vi"("error in"=w468, "Mercury Reference In"=w467) -> ("error out"=w470:errorcluster, "Unit"=→"Unit 3":T3, "Scaling Factor"=→"Scaling Factor":dbl, "Mercury Reference Out"=w469:T35)  [unwired: 1 in, 5 out]
            n179 = call-poly <instrlib>:"Configuration (Read).vi"("error in"=w470, "Mercury Reference In"=w469) -> ("error out"=w438:errorcluster, "Unit"=→"Unit 4":T3, "Temp Err"=→"Temp Err":dbl, "Mercury Reference Out"=w434:T35)  [unwired: 1 in, 5 out]
            n180 = call-poly <instrlib>:"Configuration (Read).vi"("error in"=w438, "Mercury Reference In"=w434) -> ("error out"=w442:errorcluster, "Unit"=→"Unit 5":T3, "Temp V Err"=→"Temp V Err":dbl, "Mercury Reference Out"=w441:T35)  [unwired: 1 in, 5 out]
            n181 = call-poly <instrlib>:"Configuration (Read).vi"("error in"=w442, "Mercury Reference In"=w441) -> ("error out"=w444:errorcluster, "Unit"=→"Unit 6":T3, "Gear"=→"Gear":u32, "Mercury Reference Out"=w443:T35)  [unwired: 1 in, 5 out]
            n182 = call-poly <instrlib>:"Configuration (Read).vi"("error in"=w444, "Mercury Reference In"=w443) -> ("error out"=w452:errorcluster, "Unit"=→"Unit 7":T3, "Speed"=→"Speed":u32, "Mercury Reference Out"=w451:T35)  [unwired: 1 in, 5 out]
            n183 = call-poly <instrlib>:"Signals (Read).vi"("error in"=w452, "Mercury Reference In"=w451) -> ("error out"=w454:errorcluster, "Unit"=→"Unit":T3, "Position"=→"Position":u32, "Mercury Reference Out"=w453:T35)  [unwired: 1 in, 5 out]
            n184 = call-poly <instrlib>:"Signals (Read).vi"("error in"=w454, "Mercury Reference In"=w453) -> ("error out"=w440:errorcluster, "Unit"=→"Unit":T3, "% Open"=→"% Open":dbl)  [unwired: 1 in, 6 out]
            n185 = call <vilib>:"Add State(s) to Queue__JKI_lib_State_Machine.vi"("State(s) in (\"\")"=w477) -> ("States Out"=w478:string)  [unwired: 14 in]
          }
          frame "Mercury: Query ITC: Pressure" {
            # "Pressure"
            n186 = Unbundle By Name(w486) -> ("Mercury ITC Ref"=w483:T35)
            n187 = local read "ITC Devices"() -> (w485:string[])
            n188 = Index Array(array=w485, index=1) -> (element=w482:string)
            n189 = call-poly <instrlib>:"Open.vi"("error in (no error)"=w481, "Device Identifier"=w482, "Mercury Reference In"=w483) -> ("error out"=w489:errorcluster, "Mercury Reference Out"=w490:T35)  [unwired: 7 out]
            n190 = call-poly <instrlib>:"Configuration (Read).vi"("error in"=w489, "Mercury Reference In"=w490) -> ("error out"=w491:errorcluster, "Device Details"=w488:T45, "Mercury Reference Out"=w492:T35)  [unwired: 1 in, 6 out]
            n191 = Unbundle By Name(w488) -> ("Manufacturing"=→"Manufacturing":T8, "Pressure Signals"=→"Pressure Signals":T11)
            n192 = call-poly <instrlib>:"Configuration (Read).vi"("error in"=w491, "Mercury Reference In"=w492) -> ("error out"=w496:errorcluster, "Nickname"=→"Nickname":string, "Mercury Reference Out"=w497:T35)  [unwired: 1 in, 6 out]
            n193 = call-poly <instrlib>:"Signals (Read).vi"("error in"=w496, "Mercury Reference In"=w497) -> ("error out"=w494:errorcluster, "Current"=→"Current":dbl, "Mercury Reference Out"=w495:T35)  [unwired: 1 in, 6 out]
            n194 = call-poly <instrlib>:"Signals (Read).vi"("error in"=w494, "Mercury Reference In"=w495) -> ("error out"=w487:errorcluster, "Voltage"=→"Voltage":dbl)  [unwired: 1 in, 7 out]
            n195 = call <vilib>:"Add State(s) to Queue__JKI_lib_State_Machine.vi"("State(s) in (\"\")"=w500) -> ("States Out"=w501:string)  [unwired: 14 in]
          }
          frame "Mercury: Query IPS: System" {
            # "Your code here.\n(You can make a copy of, or modify, this frame)"
            n196 = Unbundle By Name(w543) -> ("Mercury IPS Ref"=w504:T35)
            n197 = call-poly <instrlib>:"Configuration (Read).vi"("error in"=w509, "Mercury Reference In"=w504) -> ("error out"=w529:errorcluster, "Devices"=→"IPS Devices":string[], "Mercury Reference Out"=w528:T35)  [unwired: 1 in, 6 out]
            n198 = call-poly <instrlib>:"Configuration (Read).vi"("error in"=w529, "Mercury Reference In"=w528) -> ("error out"=w533:errorcluster, "Automatic Dimming"=→"Automatic Dimming 2":string, "Mercury Reference Out"=w532:T35)  [unwired: 1 in, 6 out]
            n199 = call-poly <instrlib>:"Configuration (Read).vi"("error in"=w533, "Mercury Reference In"=w532) -> ("error out"=w530:errorcluster, "Dimming Time"=→"Dimming Time 2":string, "Mercury Reference Out"=w531:T35)  [unwired: 1 in, 6 out]
            n200 = call-poly <instrlib>:"Configuration (Read).vi"("error in"=w530, "Mercury Reference In"=w531) -> ("error out"=w527:errorcluster, "Display Brightness"=→"Display Brightness 2":string, "Mercury Reference Out"=w526:T35)  [unwired: 1 in, 6 out]
            n201 = call-poly <instrlib>:"Configuration (Read).vi"("error in"=w527, "Mercury Reference In"=w526) -> ("error out"=w536:errorcluster, "Date"=→"Date 2":string, "Mercury Reference Out"=w537:T35)  [unwired: 1 in, 6 out]
            n202 = call-poly <instrlib>:"Configuration (Read).vi"("error in"=w536, "Mercury Reference In"=w537) -> ("error out"=w534:errorcluster, "Time"=→"Time 2":string, "Mercury Reference Out"=w535:T35)  [unwired: 1 in, 6 out]
            n203 = call-poly <instrlib>:"Configuration (Read).vi"("error in"=w534, "Mercury Reference In"=w535) -> ("error out"=w508:errorcluster, "time stamp"=→"time stamp 2":timestamp, "Mercury Reference Out"=w505:T35)  [unwired: 1 in, 6 out]
            n204 = call-poly <instrlib>:"Configuration (Read).vi"("error in"=w508, "Mercury Reference In"=w505) -> ("error out"=w510:errorcluster, "Hardware Version"=→"Hardware Version 2":string, "Mercury Reference Out"=w511:T35)  [unwired: 1 in, 6 out]
            n205 = call-poly <instrlib>:"Configuration (Read).vi"("error in"=w510, "Mercury Reference In"=w511) -> ("error out"=w512:errorcluster, "Firmware Version"=→"Firmware Version 2":string, "Mercury Reference Out"=w513:T35)  [unwired: 1 in, 6 out]
            n206 = call-poly <instrlib>:"Configuration (Read).vi"("error in"=w512, "Mercury Reference In"=w513) -> ("error out"=w518:errorcluster, "Serial Number"=→"Serial Number 2":string, "Mercury Reference Out"=w519:T35)  [unwired: 1 in, 6 out]
            n207 = call-poly <instrlib>:"Configuration (Read).vi"("error in"=w518, "Mercury Reference In"=w519) -> ("error out"=w514:errorcluster, "Free Space"=→"Free Space 2":i32, "Mercury Reference Out"=w515:T35)  [unwired: 1 in, 6 out]
            n208 = call-poly <instrlib>:"Configuration (Read).vi"("error in"=w514, "Mercury Reference In"=w515) -> ("error out"=w517:errorcluster, "Mode"=→"String 2":T32, "Mercury Reference Out"=w516:T35)  [unwired: 1 in, 6 out]
            n209 = Get Date/Time In Seconds() -> (seconds since 1Jan1904=w525:timestamp)
            n210 = call-poly <instrlib>:"Configuration (Set).vi"("error in"=w517, "time stamp"=w525, "Mercury Reference In"=w516) -> ("error out"=w507:errorcluster, "Response"=→"Set Date Response 2":T34)  [unwired: 1 in, 6 out]
            n211 = call <vilib>:"Add State(s) to Queue__JKI_lib_State_Machine.vi"("State(s) in (\"\")"=w545) -> ("States Out"=w544:string)  [unwired: 14 in]
          }
          frame "Mercury: Query IPS: LVL" {
            # "level"
            # "Level"
            n212 = Unbundle By Name(w585) -> ("Mercury IPS Ref"=w548:T35)
            n213 = local read "IPS Devices"() -> (w584:string[])
            n214 = Index Array(array=w584, index=0) -> (element=w547:string)
            n215 = call-poly <instrlib>:"Open.vi"("error in (no error)"=w554, "Device Identifier"=w547, "Mercury Reference In"=w548) -> ("error out"=w570:errorcluster, "Mercury Reference Out"=w569:T35)  [unwired: 7 out]
            n216 = call-poly <instrlib>:"Configuration (Read).vi"("error in"=w570, "Mercury Reference In"=w569) -> ("error out"=w575:errorcluster, "LVL Device Settings"=→"LVL Device DetailSettings":T14, "Mercury Reference Out"=w572:T35)  [unwired: 1 in, 6 out]
            n217 = call-poly <instrlib>:"Configuration (Read).vi"("error in"=w575, "Mercury Reference In"=w572) -> ("error out"=w576:errorcluster, "Serial Number"=→"LVL S/N":string, "Mercury Reference Out"=w574:T35)  [unwired: 1 in, 6 out]
            n218 = call-poly <instrlib>:"Configuration (Read).vi"("error in"=w576, "Mercury Reference In"=w574) -> ("error out"=w579:errorcluster, "Resistance Configuration"=→"He Res Config":T19, "Mercury Reference Out"=w578:T35)  [unwired: 1 in, 6 out]
            n219 = call-poly <instrlib>:"Configuration (Read).vi"("error in"=w579, "Mercury Reference In"=w578) -> ("error out"=w581:errorcluster, "Magnitude"=→"LVL P Magnitude":dbl, "Mercury Reference Out"=w580:T35)  [unwired: 1 in, 6 out]
            n220 = call-poly <instrlib>:"Configuration (Read).vi"("error in"=w581, "Mercury Reference In"=w580) -> ("error out"=w553:errorcluster, "Duration"=→"LVL P Duration":dbl, "Mercury Reference Out"=w551:T35)  [unwired: 1 in, 6 out]
            n221 = call-poly <instrlib>:"Configuration (Read).vi"("error in"=w553, "Mercury Reference In"=w551) -> ("error out"=w557:errorcluster, "Freq 100%"=→"N Freq 100%":dbl, "Mercury Reference Out"=w556:T35)  [unwired: 1 in, 6 out]
            n222 = call-poly <instrlib>:"Configuration (Read).vi"("error in"=w557, "Mercury Reference In"=w556) -> ("error out"=w560:errorcluster, "Pulse Period"=→"N Pulse Period":dbl, "Mercury Reference Out"=w559:T35)  [unwired: 1 in, 6 out]
            n223 = call-poly <instrlib>:"Signals (Read).vi"("error in"=w560, "Mercury Reference In"=w559) -> ("error out"=w562:errorcluster, "Resistance"=→"He Resistance":dbl, "Mercury Reference Out"=w561:T35)  [unwired: 1 in, 6 out]
            n224 = call-poly <instrlib>:"Signals (Read).vi"("error in"=w562, "Mercury Reference In"=w561) -> ("error out"=w564:errorcluster, "Level"=→"He Level" →"He LEVEL":dbl, "Mercury Reference Out"=w563:T35)  [unwired: 1 in, 6 out]
            n225 = call-poly <instrlib>:"Signals (Read).vi"("error in"=w564, "Mercury Reference In"=w563) -> ("error out"=w566:errorcluster, "Counter"=→"N Counter":u32, "Mercury Reference Out"=w565:T35)  [unwired: 1 in, 6 out]
            n226 = call-poly <instrlib>:"Signals (Read).vi"("error in"=w566, "Mercury Reference In"=w565) -> ("error out"=w552:errorcluster, "Level"=→"N Level" →"N2 LEVEL":dbl)  [unwired: 1 in, 7 out]
            n227 = call <vilib>:"Add State(s) to Queue__JKI_lib_State_Machine.vi"("State(s) in (\"\")"=w586) -> ("States Out"=w587:string)  [unwired: 14 in]
          }
          frame "Mercury: Query IPS: Temperature" {
            # "temperature"
            n228 = Unbundle By Name(w632) -> ("Mercury IPS Ref"=w593:T35)
            n229 = local read "IPS Devices"() -> (w631:string[])
            n230 = Index Array(array=w631, index=4) -> (element=w594:string)
            n231 = call-poly <instrlib>:"Open.vi"("error in (no error)"=w592, "Device Identifier"=w594, "Mercury Reference In"=w593) -> ("error out"=w619:errorcluster, "Mercury Reference Out"=w614:T35)  [unwired: 7 out]
            n232 = call-poly <instrlib>:"Configuration (Read).vi"("error in"=w619, "Mercury Reference In"=w614) -> ("error out"=w620:errorcluster, "Serial Number"=→"Temp S/N 2":string, "Mercury Reference Out"=w615:T35)  [unwired: 1 in, 6 out]
            n233 = call-poly <instrlib>:"Configuration (Read).vi"("error in"=w620, "Mercury Reference In"=w615) -> ("error out"=w621:errorcluster, "Nickname"=→"T Nickname 2":string, "Mercury Reference Out"=w616:T35)  [unwired: 1 in, 6 out]
            n234 = call-poly <instrlib>:"Configuration (Read).vi"("error in"=w621, "Mercury Reference In"=w616) -> ("error out"=w622:errorcluster, "Unit"=→"Unit 12":T3, "Excitation Magnitude"=→"Excitation Magnitude 2":dbl, "Mercury Reference Out"=w617:T35)  [unwired: 1 in, 5 out]
            n235 = call-poly <instrlib>:"Configuration (Read).vi"("error in"=w622, "Mercury Reference In"=w617) -> ("error out"=w623:errorcluster, "Sensor Type"=→"Sensor Type 2":T41, "Mercury Reference Out"=w618:T35)  [unwired: 1 in, 6 out]
            n236 = call-poly <instrlib>:"Configuration (Read).vi"("error in"=w623, "Mercury Reference In"=w618) -> ("error out"=w596:errorcluster, "Excitation Type"=→"Excitation Type 2":T7, "Mercury Reference Out"=w595:T35)  [unwired: 1 in, 6 out]
            n237 = call-poly <instrlib>:"Configuration (Read).vi"("error in"=w596, "Mercury Reference In"=w595) -> ("error out"=w601:errorcluster, "Unit"=→"H Unit 2":T3, "Hot Limit"=→"Hot Limit 2":dbl, "Mercury Reference Out"=w597:T35)  [unwired: 1 in, 5 out]
            n238 = call-poly <instrlib>:"Configuration (Read).vi"("error in"=w601, "Mercury Reference In"=w597) -> ("error out"=w602:errorcluster, "Unit"=→"C Unit 2":T3, "Cold Limit"=→"Cold Limit 2":dbl, "Mercury Reference Out"=w598:T35)  [unwired: 1 in, 5 out]
            n239 = call-poly <instrlib>:"Signals (Read).vi"("error in"=w602, "Mercury Reference In"=w598) -> ("error out"=w603:errorcluster, "Unit"=→"V Unit 2":T3, "Voltage"=→"Voltage 2":dbl, "Mercury Reference Out"=w599:T35)  [unwired: 1 in, 5 out]
            n240 = call-poly <instrlib>:"Signals (Read).vi"("error in"=w603, "Mercury Reference In"=w599) -> ("error out"=w604:errorcluster, "Unit"=→"T Unit 2":T3, "Temperature"=→"Temperature 2":dbl, "Mercury Reference Out"=w600:T35)  [unwired: 1 in, 5 out]
            n241 = call-poly <instrlib>:"Configuration (Read).vi"("error in"=w604, "Mercury Reference In"=w600) -> ("error out"=w605:errorcluster, "Device Details"=w588:T42)  [unwired: 1 in, 7 out]
            n242 = Unbundle By Name(w588) -> ("Manufacturing"=→"IPS Manufacturing":T8, "Excitation"=→"IPS Excitation":T6, "Calibration"=→"IPS Calibration":T4)
            n243 = call <vilib>:"Add State(s) to Queue__JKI_lib_State_Machine.vi"("State(s) in (\"\")"=w633) -> ("States Out"=w634:string)  [unwired: 14 in]
          }
          frame "Mercury: Query IPS: Magnet" {
            n244 = Unbundle By Name(w673) -> ("Mercury IPS Ref"=w639:T35)
            n245 = call-poly <instrlib>:"Open.vi"("error in (no error)"=w635, "Device Identifier"="Device Identifier", "Mercury Reference In"=w639) -> ("error out"=w658:errorcluster, "Mercury Reference Out"=w657:T35)  [unwired: 7 out]
            n246 = call-poly <instrlib>:"Configuration (Read).vi"("error in"=w658, "Mercury Reference In"=w657) -> ("error out"=w661:errorcluster, "Magnet Device Details"=→"Magnet Device Details":T22, "Mercury Reference Out"=w660:T35)  [unwired: 1 in, 6 out]
            n247 = call-poly <instrlib>:"Configuration (Read).vi"("error in"=w661, "Mercury Reference In"=w660) -> ("error out"=w664:errorcluster, "Serial Number"=→"Mag S/N":string, "Mercury Reference Out"=w663:T35)  [unwired: 1 in, 6 out]
            n248 = call-poly <instrlib>:"Configuration (Read).vi"("error in"=w664, "Mercury Reference In"=w663) -> ("error out"=w667:errorcluster, "Bipolar Output"=→"Bipolar Output":string, "Mercury Reference Out"=w666:T35)  [unwired: 1 in, 6 out]
            n249 = call-poly <instrlib>:"Configuration (Read).vi"("error in"=w667, "Mercury Reference In"=w666) -> ("error out"=w670:errorcluster, "Out Config"=→"Out Config":T50, "Mercury Reference Out"=w669:T35)  [unwired: 1 in, 6 out]
            n250 = call-poly <instrlib>:"Configuration (Read).vi"("error in"=w670, "Mercury Reference In"=w669) -> ("error out"=w641:errorcluster, "Unit"=→"Unit 8":T3, "Current Limit"=→"Current Limit":dbl, "Mercury Reference Out"=w638:T35)  [unwired: 1 in, 5 out]
            n251 = call-poly <instrlib>:"Configuration (Read).vi"("error in"=w641, "Mercury Reference In"=w638) -> ("error out"=w644:errorcluster, "Unit"=→"Unit 9":T3, "AtoB"=→"AtoB":dbl, "Mercury Reference Out"=w643:T35)  [unwired: 1 in, 5 out]
            n252 = call-poly <instrlib>:"Configuration (Read).vi"("error in"=w644, "Mercury Reference In"=w643) -> ("error out"=w647:errorcluster, "Switch Present"=→"Switch Present":string, "Mercury Reference Out"=w646:T35)  [unwired: 1 in, 6 out]
            n253 = call-poly <instrlib>:"Configuration (Read).vi"("error in"=w647, "Mercury Reference In"=w646) -> ("error out"=w652:errorcluster, "Unit"=→"Unit 10":T3, "SW VLIM"=→"SW VLIM":dbl, "Mercury Reference Out"=w651:T35)  [unwired: 1 in, 5 out]
            n254 = call-poly <instrlib>:"Signals (Read).vi"("error in"=w652, "Mercury Reference In"=w651) -> ("error out"=w654:errorcluster, "Unit"=→"Unit 11":T3, "Current Rate"=→"Current Rate":dbl, "Mercury Reference Out"=w653:T35)  [unwired: 1 in, 5 out]
            n255 = call-poly <instrlib>:"Signals (Read).vi"("error in"=w654, "Mercury Reference In"=w653) -> ("error out"=w640:errorcluster, "PSU Act Stat"=→"PSU Act Stat":T51)  [unwired: 1 in, 7 out]
            n256 = call <vilib>:"Add State(s) to Queue__JKI_lib_State_Machine.vi"("State(s) in (\"\")"=w674) -> ("States Out"=w675:string)  [unwired: 14 in]
          }
          frame "---------- Mercury: Idle ----------" {
            n257 = call <vilib>:"Add State(s) to Queue__JKI_lib_State_Machine.vi"("State(s) in (\"\")"=w679) -> ("States Out"=w678:string)  [unwired: 14 in]
          }
          frame "Mercury: Idle" {
            # "#Implemented: Get IPS Magnet Temperature.vi"
            n258 = Unbundle By Name(w683) -> ("LEDs"=w681:bool[], "Mercury IPS Ref"=w700:T35, "Mercury ITC Ref"=w699:T35)
            n259 = Not(x=w681) -> (.not. x?=w680:bool[])
            "LEDs" <- w680
            n260 = disable-structure shown="Enabled" {
              disable-tunnel: w699 -> [w719 _]
              disable-tunnel: w698 -> [w718 w721]
              disable-tunnel: [w705 w721] -> w694
              frame Disabled {
                n261 = local read "ITC Devices"() -> (w716:string[])
                n262 = Index Array(array=w716, index=3) -> (element=w709:string)
                n263 = call-poly <instrlib>:"Open.vi"("error in (no error)"=w718, "Device Identifier"=w709, "Mercury Reference In"=w719) -> ("error out"=w715:errorcluster, "Mercury Reference Out"=w713:T35)  [unwired: 7 out]
                n264 = call-poly <instrlib>:"Signals (Read).vi"("error in"=w715, "Mercury Reference In"=w713) -> ("error out"=w712:errorcluster, "Temperature"=→"LPF Temperature":dbl, "Mercury Reference Out"=w711:T35)  [unwired: 1 in, 6 out]
                n265 = call-poly <instrlib>:"Signals (Read).vi"("error in"=w712, "Mercury Reference In"=w711) -> ("error out"=w708:errorcluster, "Resistance"=→"LPF Resistance":dbl, "Mercury Reference Out"=w707:T35)  [unwired: 1 in, 6 out]
                n266 = call-poly <instrlib>:"Configuration (Set).vi"("error in"=w708, "Excitation Magnitude"=0.0, "Mercury Reference In"=w707) -> ("error out"=w705:errorcluster, "Response"=w704:T34)  [unwired: 5 in, 2 out]
                n267 = call "1820 State History.vi"("Current State in"=w704) -> ("delimited string"=w703:string)  [unwired: 9 in, 1 out]
                n268 = local write "Magnet Status 2"(w703) -> ()
              }
              frame Enabled {
                w720 = -1.0 ("LPF Temperature")
                n269 = local write "LPF Temperature"(w720) -> ()
                n270 = local write "LPF Resistance"(w720) -> ()
              }
            }
            n271 = local read "IPS Devices"() -> (w697:string[])
            n272 = Index Array(array=w697, index=5) -> (element=w695:string)
            n273 = Bundle By Name(cluster=w683, "LEDs"=w680) -> (w682:T38)
            n274 = call-poly <instrlib>:"Open.vi"("error in (no error)"=w694, "Device Identifier"=w695, "Mercury Reference In"=w700) -> ("error out"=w691:errorcluster, "Mercury Reference Out"=w692:T35)  [unwired: 7 out]
            n275 = call-poly <instrlib>:"Signals (Read).vi"("error in"=w691, "Mercury Reference In"=w692) -> ("error out"=w684:errorcluster, "Temperature"=→"Magnet Temperature":dbl, "Mercury Reference Out"=w693:T35)  [unwired: 1 in, 6 out]
            n276 = call "Read IPS Temperature.vi"() -> ()  [unwired: 8 in, 4 out]
            n277 = call-poly <instrlib>:"Signals (Read).vi"("error in"=w684, "Mercury Reference In"=w693) -> ("error out"=w687:errorcluster, "Resistance"=→"Magnet Resistance":dbl, "Mercury Reference Out"=w688:T35)  [unwired: 1 in, 6 out]
            n278 = First Call?() -> (First Call?: T/F=w685:bool)
            n279 = case shown="True" w685 {
              tunnel: [w722 w725] -> w686
              tunnel: w688 -> [_ w724]
              tunnel: w687 -> [w722 w723]
              frame False {
              }
              frame True {
                n280 = disable-structure shown="Disabled" {
                  disable-tunnel: [w731 _] -> w725
                  disable-tunnel: w724 -> [w727 _]
                  disable-tunnel: w723 -> [w726 _]
                  frame Disabled {
                    n281 = call-poly <instrlib>:"Configuration (Set).vi"("error in"=w726, "Excitation Magnitude"=20.0, "Mercury Reference In"=w727) -> ("error out"=w731:errorcluster, "Response"=w729:T34)  [unwired: 5 in, 2 out]
                    n282 = call "1820 State History.vi"("Current State in"=w729) -> ("delimited string"=w728:string)  [unwired: 9 in, 1 out]
                    n283 = local write "Magnet Status 2"(w728) -> ()
                  }
                  frame Enabled {
                  }
                }
              }
            }
            n284 = call <vilib>:"Add State(s) to Queue__JKI_lib_State_Machine.vi"("State(s) in (\"\")"=w701) -> ("States Out"=w702:string)  [unwired: 14 in]
          }
          frame "Mercury: IPS: Idle - 1" {
            # "#Implemented: Read IPS Status"
            # "#Implemented: Read IPS Magnet Field"
            # "#Implemented: Read IPS Targets"
            # "#Implemented: Read IPS PSU Field"
            # "#Implemented: Read IPS PSU Current Voltage"
            # "#Implemented: Read IPS Switch Heater"
            # "Magnet"
            # "set switch status"
            n285 = Unbundle By Name(w735) -> ("Mercury IPS Ref"=w738:T35)
            n286 = local read "Device Identifier"() -> (w751:T24)
            n287 = call-poly <instrlib>:"Configuration (Read).vi"("error in"=w766, "Mercury Reference In"=w738) -> ("error out"=w758:errorcluster, "Time"=w761:string, "Mercury Reference Out"=w759:T35)  [unwired: 1 in, 6 out]
            n288 = local write "Time 2"(w761) -> ()
            n289 = call-poly <instrlib>:"Open.vi"("error in (no error)"=w758, "Device Identifier"=w751, "Mercury Reference In"=w759) -> ("error out"=w757:errorcluster, "Mercury Reference Out"=w756:T35)  [unwired: 7 out]
            n290 = call-poly <instrlib>:"Signals (Read).vi"("error in"=w757, "Mercury Reference In"=w756) -> ("error out"=w733:errorcluster, "Switch Heater Status"=w737:string, "Mercury Reference Out"=w732:T35)  [unwired: 1 in, 6 out]
            n291 = call "Read IPS Switch Heater.vi"() -> ()  [unwired: 8 in, 4 out]
            n292 = Equal?(x=w737, y="ON") -> (x = y?=→"SWITCH HEATER":bool)
            n293 = call-poly <instrlib>:"Signals (Read).vi"("error in"=w733, "Mercury Reference In"=w732) -> ("error out"=w765:errorcluster, "Current"=→"Current (A)" →"Current (A)":dbl, "Mercury Reference Out"=w763:T35)  [unwired: 1 in, 6 out]
            n294 = call "Read IPS PSU Current Voltage.vi"() -> ()  [unwired: 8 in, 4 out]
            n295 = call-poly <instrlib>:"Signals (Read).vi"("error in"=w765, "Mercury Reference In"=w763) -> ("error out"=w750:errorcluster, "Voltage"=→"Voltage (V)" →"Voltage (V)":dbl, "Mercury Reference Out"=w749:T35)  [unwired: 1 in, 6 out]
            n296 = call-poly <instrlib>:"Signals (Read).vi"("error in"=w750, "Mercury Reference In"=w749) -> ("error out"=w752:errorcluster, "Field"=→"Power Supply Field (T)":dbl, "Mercury Reference Out"=w755:T35)  [unwired: 1 in, 6 out]
            n297 = call-poly <instrlib>:"Signals (Read).vi"("error in"=w752, "Mercury Reference In"=w755) -> ("error out"=w753:errorcluster, "Target Field Rate"=→"Target Field Rate (T/min)":dbl, "Mercury Reference Out"=w754:T35)  [unwired: 1 in, 6 out]
            n298 = call "Read IPS PSU Targets.vi"() -> ()  [unwired: 8 in, 4 out]
            n299 = call-poly <instrlib>:"Signals (Read).vi"("error in"=w753, "Mercury Reference In"=w754) -> ("error out"=w748:errorcluster, "Target Field"=→"Target Field (T)":dbl, "Mercury Reference Out"=w747:T35)  [unwired: 1 in, 6 out]
            n300 = call-poly <instrlib>:"Signals (Read).vi"("error in"=w748, "Mercury Reference In"=w747) -> ("error out"=w764:errorcluster, "Persistant Field"=→"Magnet Field (T)" →"Magnet Field (T)":dbl, "Mercury Reference Out"=w762:T35)  [unwired: 1 in, 6 out]
            n301 = call "Read IPS PSU Field.vi"() -> ()  [unwired: 9 in, 3 out]
            n302 = call "Read IPS Magnet Field.vi"() -> ()  [unwired: 9 in, 3 out]
            n303 = call-poly <instrlib>:"Signals (Read).vi"("error in"=w764, "Mercury Reference In"=w762) -> ("error out"=w736:errorcluster, "PSU Act Stat"=w739:T51)  [unwired: 1 in, 7 out]
            n304 = local write "PSU Act Stat"(w739) -> ()
            n305 = call "Read IPS Status.vi"() -> ()  [unwired: 9 in, 3 out]
            n306 = case shown="\"RTOZ\"" w739 {
              selector: w739 -> [w769 _ _ _ _]
              tunnel: [w769 "Holding" "Ramping to Setpoint" "Ramping to Zero" "Clamped"] -> w746
              frame Default {
              }
              frame "HOLD" {
              }
              frame "RTOS" {
              }
              frame "RTOZ" {
              }
              frame "CLMP" {
              }
            }
            "Magnet Status" <- w746
            n307 = call <vilib>:"Add State(s) to Queue__JKI_lib_State_Machine.vi"("State(s) in (\"\")"=w767) -> ("States Out"=w768:string)  [unwired: 14 in]
          }
          frame "Mercury: IPS: Idle - 1a" {
            # "#implemented: Read IPS PSU1/2/3 Current Voltage"
            n308 = local read "IPS Devices"() -> (w799:string[])
            n309 = Unbundle By Name(w803) -> ("Mercury IPS Ref"=w802:T35)
            n310 = for {
              tunnel: w799 -> [w807] mode=indexing
              tunnel: [w806] -> w798 mode=indexing
              n311 = Match Pattern(string=w807, regular expression=":PSU") -> (before substring=w806:string)  [unwired: 1 in, 3 out]
            }
            n312 = Index Array(array=w798, index #1=6 ("index")) -> (element #1=w800:string, element #2=w796:string, element #3=w797:string)  [unwired: 2 in]
            n313 = call-poly <instrlib>:"Open.vi"("error in (no error)"=w801, "Device Identifier"=w800, "Mercury Reference In"=w802) -> ("error out"=w778:errorcluster, "Mercury Reference Out"=w782:T35)  [unwired: 7 out]
            n314 = call-poly <instrlib>:"Signals (Read).vi"("error in"=w778, "Mercury Reference In"=w782) -> ("error out"=w784:errorcluster, "Current"=→"M1 Current":dbl, "Mercury Reference Out"=w783:T35)  [unwired: 1 in, 6 out]
            n315 = call-poly <instrlib>:"Signals (Read).vi"("error in"=w784, "Mercury Reference In"=w783) -> ("error out"=w776:errorcluster, "Voltage"=→"M1 Voltage":dbl)  [unwired: 1 in, 7 out]
            n316 = call-poly <instrlib>:"Open.vi"("error in (no error)"=w776, "Device Identifier"=w796, "Mercury Reference In"=w802) -> ("error out"=w779:errorcluster, "Mercury Reference Out"=w781:T35)  [unwired: 7 out]
            n317 = call "Read IPS PSU1 Current Voltage.vi"() -> ()  [unwired: 8 in, 4 out]
            n318 = call-poly <instrlib>:"Signals (Read).vi"("error in"=w779, "Mercury Reference In"=w781) -> ("error out"=w787:errorcluster, "Current"=→"M2 Current":dbl, "Mercury Reference Out"=w785:T35)  [unwired: 1 in, 6 out]
            n319 = call "Read IPS PSU2 Current Voltage.vi"() -> ()  [unwired: 8 in, 4 out]
            n320 = call-poly <instrlib>:"Signals (Read).vi"("error in"=w787, "Mercury Reference In"=w785) -> ("error out"=w774:errorcluster, "Voltage"=→"M2 Voltage":dbl)  [unwired: 1 in, 7 out]
            n321 = call "Read IPS PSU3 Current Voltage.vi"() -> ()  [unwired: 8 in, 4 out]
            n322 = call-poly <instrlib>:"Open.vi"("error in (no error)"=w774, "Device Identifier"=w797, "Mercury Reference In"=w802) -> ("error out"=w777:errorcluster, "Mercury Reference Out"=w780:T35)  [unwired: 7 out]
            n323 = call-poly <instrlib>:"Signals (Read).vi"("error in"=w777, "Mercury Reference In"=w780) -> ("error out"=w788:errorcluster, "Current"=→"M3 Current":dbl, "Mercury Reference Out"=w786:T35)  [unwired: 1 in, 6 out]
            n324 = call-poly <instrlib>:"Signals (Read).vi"("error in"=w788, "Mercury Reference In"=w786) -> ("error out"=w775:errorcluster, "Voltage"=→"M3 Voltage":dbl)  [unwired: 1 in, 7 out]
            n325 = call <vilib>:"Add State(s) to Queue__JKI_lib_State_Machine.vi"("State(s) in (\"\")"=w804) -> ("States Out"=w805:string)  [unwired: 14 in]
          }
          frame "Mercury: IPS: Idle - 2" {
            w811 = enum16{"write", "read"}."write" ("Function")
            # "#implemented: Read IPS Level"
            # "set all of these things"
            n326 = Unbundle By Name(w819) -> ("Mercury IPS Ref"=w831:T35)
            n327 = local read "IPS Devices"() -> (w856:string[])
            n328 = Index Array(array=w856, index=0) -> (element=w855:string)
            n329 = call-poly <instrlib>:"Open.vi"("error in (no error)"=w852, "Device Identifier"=w855, "Mercury Reference In"=w831) -> ("error out"=w858:errorcluster, "Mercury Reference Out"=w859:T35)  [unwired: 7 out]
            n330 = call-poly <instrlib>:"Signals (Read).vi"("error in"=w858, "Mercury Reference In"=w859) -> ("error out"=w860:errorcluster, "Level"=w843:dbl, "Mercury Reference Out"=w861:T35)  [unwired: 1 in, 6 out]
            "He LVL Chart" <- w843
            n331 = call "Read IPS Level.vi"() -> ()  [unwired: 8 in, 4 out]
            n332 = Greater?(x=w843, y=20.0) -> (0:w850:bool)
            n333 = Greater?(x=w843, y=50.0) -> (0:w851:bool)
            n334 = call-poly <instrlib>:"Signals (Read).vi"("error in"=w860, "Mercury Reference In"=w861) -> ("error out"=w809:errorcluster, "Level"=w842:dbl)  [unwired: 1 in, 7 out]
            "N2 LVL Chart" <- w842
            n335 = case shown="False" w850 {
              tunnel: [w869 u32 6618880] -> w840
              tunnel: w851 -> [w870 _]
              frame False {
                n336 = case shown="False" w870 {
                  tunnel: [u32 16711680 u32 16776704] -> w869
                  frame False {
                  }
                  frame True {
                  }
                }
              }
              frame True {
              }
            }
            n337 = local write "He LEVEL"(w843) -> ()
            n338 = property on="He LVL Chart" class="Slide (strict)"("Fill Color"=w840) -> ()  [unwired: 2 in, 2 out]
            n339 = property on="He LEVEL" class="DigNum (strict)"("NumText.TextColor"=w840) -> ()  [unwired: 2 in, 2 out]
            n340 = local write "N2 LEVEL"(w842) -> ()
            n341 = local read "Target Field Rate (T/min)"() -> (w836:dbl)
            n342 = local read "Power Supply Field (T)"() -> (w834:dbl)
            n343 = Greater?(x=w842, y=20.0) -> (0:w845:bool)
            n344 = Greater?(x=w842, y=50.0) -> (0:w844:bool)
            n345 = local read "Magnet Field (T)"() -> (w833:dbl)
            n346 = local read "Target Field (T)"() -> (w835:dbl)
            n347 = local read "Current (A)"() -> (w838:dbl)
            n348 = local read "Voltage (V)"() -> (w837:dbl)
            n349 = local read "SWITCH HEATER"() -> (w820:bool)
            n350 = local read "PSU Act Stat"() -> (w812:string)
            n351 = case shown="True" w845 {
              tunnel: [w864 u32 6618880] -> w841
              tunnel: w844 -> [w865 _]
              frame False {
                n352 = case shown="False" w865 {
                  tunnel: [u32 16711680 u32 16776704] -> w864
                  frame False {
                  }
                  frame True {
                  }
                }
              }
              frame True {
              }
            }
            n353 = local read "Magnet Temperature"() -> (w829:dbl)
            n354 = property on="N2 LVL Chart" class="Slide (strict)"("Fill Color"=w841) -> ()  [unwired: 2 in, 2 out]
            n355 = property on="N2 LEVEL" class="DigNum (strict)"("NumText.TextColor"=w841) -> ()  [unwired: 2 in, 2 out]
            n356 = Bundle By Name(cluster=T29 {"Magnet Field"=0.0, "PS Field"=0.0, "Target Field"=0.0, "Target Field Rate"=0.0, "Voltage"=0.0, "Current"=0.0, "Switch"=FALSE, "Mercury State"=""} ("Status"), "Magnet Field"=w833, "PS Field"=w834, "Target Field"=w835, "Target Field Rate"=w836, "Voltage"=w837, "Current"=w838, "Switch"=w820, "Mercury State"=w812) -> (w817:T29)
            n357 = local read "Magnet Resistance"() -> (w830:dbl)
            n358 = Select(t="ON", s=w820, f="OFF") -> (s? t:f=w810:string)
            n359 = local read "M1 Current"() -> (w828:dbl)
            n360 = local read "M1 Voltage"() -> (w827:dbl)
            n361 = local read "M2 Current"() -> (w826:dbl)
            n362 = local read "M2 Voltage"() -> (w825:dbl)
            n363 = local read "M3 Current"() -> (w824:dbl)
            n364 = local read "M3 Voltage"() -> (w823:dbl)
            n365 = call "FGV_PSP - Mercury Status.vi"("error in"=w809, "Function"=w811, "Status"=w817) -> ("error out"=w816:errorcluster)  [unwired: 3 in, 1 out]
            n366 = Bundle(cluster=T30 {"Magnet Field"=0.0, "PS Field"=0.0, "Target Field"=0.0, "Target Field Rate"=0.0, "Voltage"=0.0, "Current"=0.0}, "Magnet Field"=w833, "PS Field"=w834, "Target Field"=w835, "Target Field Rate"=w836, "Voltage"=w837, "Current"=w838) -> (w839:T30)
            n367 = call "FGV_PSP - Mercury Action Status.vi"("error in"=w816, "Function"=w811, "Mercury Status"=w812) -> ("error out"=w815:errorcluster)  [unwired: 3 in, 1 out]
            n368 = Cluster To Array(cluster=w839) -> (array=w814:dbl[])
            n369 = Build Array(w828, w827, w826, w825, w824, w823) -> (w813:dbl[])
            n370 = Build Array (concatenate)(w814, w842, w843, w829, w830, w813) -> (w854:dbl[])
            n371 = Build Array(w812, w810) -> (w853:string[])
            n372 = call "1820_IPS_to_DSC.vi"("str"=w853, "dbl"=w854) -> ()  [unwired: 2 in]
            n373 = call <vilib>:"Add State(s) to Queue__JKI_lib_State_Machine.vi"("State(s) in (\"\")"=w862) -> ("States Out"=w863:string)  [unwired: 14 in]
          }
          frame "Mercury: IPS: Idle - 3" {
            n374 = case shown="True" "Enable RS232 Panel" {
              tunnel: w876 -> [w880 w882]
              tunnel: [w880 w881] -> w875
              frame False {
              }
              frame True {
                n375 = call "Oxford_MNK_Omega_Sign.vi"("error in (no error)"=w882) -> ("error out"=w881:errorcluster)  [unwired: 10 in]
              }
            }
            n376 = call <vilib>:"Add State(s) to Queue__JKI_lib_State_Machine.vi"("State(s) in (\"\")"=w878) -> ("States Out"=w879:string)  [unwired: 14 in]
          }
          frame "Mercury: ITC: Idle" {
            # "#implemented: Read ITC LPF Needle Valve"
            # "#implemented: Read ITC LPF Pressure"
            # "needle valve motor"
            # "pressure sensor"
            n377 = Unbundle By Name(w904) -> ("Mercury ITC Ref"=w888:T35)
            n378 = local read "ITC Devices"() -> (w903:string[])
            n379 = call "Read ITC LPF Pressure.vi"() -> ()  [unwired: 9 in, 3 out]
            n380 = Index Array(array=w903, index=1) -> (element=w901:string)
            n381 = call-poly <instrlib>:"Open.vi"("error in (no error)"=w883, "Device Identifier"=w901, "Mercury Reference In"=w888) -> ("error out"=w900:errorcluster, "Mercury Reference Out"=w899:T35)  [unwired: 7 out]
            n382 = call-poly <instrlib>:"Configuration (Read).vi"("error in"=w900, "Mercury Reference In"=w899) -> ("error out"=w897:errorcluster, "Device Details"=w898:T45)  [unwired: 1 in, 7 out]
            n383 = local read "ITC Devices"() -> (w895:string[])
            n384 = Unbundle By Name(w898) -> ("Pressure Signals.Pressure"=w887:string)
            n385 = Index Array(array=w895, index=0) -> (element=w894:string)
            n386 = Fract/Exp String To Number(string=w887) -> (number=w886:dbl)  [unwired: 3 in, 1 out]
            "LPF Pressure" <- w886
            n387 = call-poly <instrlib>:"Open.vi"("error in (no error)"=w897, "Device Identifier"=w894, "Mercury Reference In"=w888) -> ("error out"=w893:errorcluster, "Mercury Reference Out"=w892:T35)  [unwired: 7 out]
            n388 = call "Read ITC LPF Needle Valve.vi"() -> ()  [unwired: 9 in, 3 out]
            n389 = local read "LPF Temperature"() -> (w885:dbl)
            n390 = local read "LPF Resistance"() -> (w884:dbl)
            n391 = call-poly <instrlib>:"Signals (Read).vi"("error in"=w893, "Mercury Reference In"=w892) -> ("error out"=w889:errorcluster, "% Open"=w890:dbl)  [unwired: 1 in, 7 out]
            "LPF Needle Valve (%)" <- w890
            n392 = Build Array(w885, w886, w890, w884) -> (w891:dbl[])
            n393 = call "1820_ITC_to_DSC.vi"("dbl"=w891) -> ()  [unwired: 3 in]
            n394 = call <vilib>:"Add State(s) to Queue__JKI_lib_State_Machine.vi"("State(s) in (\"\")"=w905) -> ("States Out"=w906:string)  [unwired: 14 in]
          }
          frame "Mercury: Empty" {
            n395 = call <vilib>:"Add State(s) to Queue__JKI_lib_State_Machine.vi"("State(s) in (\"\")"=w909) -> ("States Out"=w910:string)  [unwired: 14 in]
          }
          frame "---------- Mercury: Action ----------" {
            n396 = call <vilib>:"Add State(s) to Queue__JKI_lib_State_Machine.vi"("State(s) in (\"\")"=w914) -> ("States Out"=w913:string)  [unwired: 14 in]
          }
          frame "Mercury: Remote" {
            w929 = "\n"
            w922 = enum16{"write", "read"}."read" ("Function")
            n397 = call "FGV_PSP - Mercury Remote.vi"("error in"=w952, "Function"=enum16{"write", "read"}."write", "Remote"=TRUE ("Mercury FGV.Remote")) -> ("error out"=w951:errorcluster)  [unwired: 3 in, 1 out]
            n398 = call "FGV_PSP - Mercury Actions.vi"("error in"=w951, "Function"=w922) -> ("error out"=w927:errorcluster, "Actions"=w928:T31)  [unwired: 4 in]
            n399 = call "FGV_PSP - Mercury Targets.vi"("error in"=w927, "Function"=w922) -> ("error out"=w923:errorcluster, "Targets"=w926:T52)  [unwired: 4 in]
            n400 = Unbundle By Name(w926) -> ("Field (T)"=w925:dbl, "Field Rate (T/min)"=w924:dbl)
            n401 = Unbundle By Name(w928) -> ("Hold"=w921:bool, "Clamp"=w916:bool, "To Set"=w917:bool, "To Zero"=w918:bool, "PS Heat"=w919:bool, "Lambda"=w915:bool, "Send to IPS"=w920:bool)
            n402 = local read "Send to IPS"() -> (w943:bool)
            n403 = local read "Lambda"() -> (w942:bool)
            n404 = local read "To Zero"() -> (w940:bool)
            n405 = local read "PS Heat"() -> (w941:bool)
            n406 = local read "Clamp"() -> (w938:bool)
            n407 = local read "To Set"() -> (w939:bool)
            n408 = local read "Hold"() -> (w937:bool)
            n409 = local write "Send to IPS"(w920) -> ()
            n410 = local write "Lambda"(w915) -> ()
            n411 = local write "To Zero"(w918) -> ()
            n412 = local write "PS Heat"(w919) -> ()
            n413 = local write "Clamp"(w916) -> ()
            n414 = Not Equal?(x=w937, y=w921) -> (x != y?=w950:bool)
            n415 = Not Equal?(x=w938, y=w916) -> (x != y?=w949:bool)
            n416 = Not Equal?(x=w939, y=w917) -> (x != y?=w948:bool)
            n417 = local write "To Set"(w917) -> ()
            n418 = Not Equal?(x=w940, y=w918) -> (x != y?=w947:bool)
            n419 = Not Equal?(x=w941, y=w919) -> (x != y?=w946:bool)
            n420 = Not Equal?(x=w942, y=w915) -> (x != y?=w945:bool)
            n421 = Not Equal?(x=w943, y=w920) -> (x != y?=w944:bool)
            n422 = local write "Hold"(w921) -> ()
            n423 = local write "Target Field (T)"(w925) -> ()
            n424 = local write "Target Rate (T/min)"(w924) -> ()
            n425 = case shown="True" w950 {
              tunnel: ["" ("State(s) in Front (\"\")") "Mercury: Hold" ("State(s) in Front (\"\")")] -> w936
              frame False {
              }
              frame True {
              }
            }
            n426 = case shown="True" w948 {
              tunnel: ["" ("State(s) in Front (\"\")") "Mercury: To Set" ("State(s) in Front (\"\")")] -> w934
              frame False {
              }
              frame True {
              }
            }
            n427 = case shown="True" w946 {
              tunnel: ["" ("State(s) in Front (\"\")") "Mercury: PS Heat" ("State(s) in Front (\"\")")] -> w932
              frame False {
              }
              frame True {
              }
            }
            n428 = case shown="True" w945 {
              tunnel: ["" ("State(s) in Front (\"\")") "Mercury: Lambda" ("State(s) in Front (\"\")")] -> w931
              frame False {
              }
              frame True {
              }
            }
            n429 = case shown="True" w944 {
              tunnel: ["" ("State(s) in Front (\"\")") "Mercury: Send To IPS" ("State(s) in Front (\"\")")] -> w930
              frame False {
              }
              frame True {
              }
            }
            n430 = case shown="True" w949 {
              tunnel: ["" ("State(s) in Front (\"\")") "Mercury: Clamp" ("State(s) in Front (\"\")")] -> w935
              frame False {
              }
              frame True {
              }
            }
            n431 = case shown="True" w947 {
              tunnel: ["" ("State(s) in Front (\"\")") "Mercury: To Zero" ("State(s) in Front (\"\")")] -> w933
              frame False {
              }
              frame True {
              }
            }
            n432 = Concatenate Strings(w936, w929, w935, w929, w934, w929, w933, w929, w932, w929, w931, w929, w930, w929) -> (w956:string)
            n433 = call <vilib>:"Add State(s) to Queue__JKI_lib_State_Machine.vi"("State(s) in Front (\"\")"=w956, "State(s) in (\"\")"=w957) -> ("States Out"=w958:string)  [unwired: 13 in]
          }
          frame "Mercury: Hold" {
            w975 = FALSE ("Hold")
            w973 = T51 "HOLD" ("PSU Act Stat")
            # "#implemented: Set IPS Action"
            # "log action to remote variable server"
            # "keep history of commands"
            # "log reply to DSC"
            # "action set"
            # "open connection"
            n434 = Unbundle By Name(w980) -> ("Mercury IPS Ref"=w987:T35)
            n435 = local read "Device Identifier"() -> (w988:T24)
            n436 = call-poly <instrlib>:"Open.vi"("error in (no error)"=w985, "Device Identifier"=w988, "Mercury Reference In"=w987) -> ("error out"=w989:errorcluster, "Mercury Reference Out"=w986:T35)  [unwired: 7 out]
            n437 = call-poly <instrlib>:"Signals (Set).vi"("error in"=w989, "PSU Act Stat"=w973, "Mercury Reference In"=w986) -> ("error out"=w983:errorcluster, "Response"=w981:T34)  [unwired: 1 in, 6 out]
            n438 = call "IPS Reply to PGSQL.vi"("error in (no error)"=w983, "Response"=w981) -> ("error out"=w976:errorcluster)  [unwired: 9 in]
            n439 = call "Set IPS Action.vi"("PSU Act Stat"=w973) -> ()  [unwired: 8 in, 3 out]
            n440 = call "1820 State History.vi"("initialize?"=FALSE, "Current State in"=w981) -> ("delimited string"=w984:string)  [unwired: 8 in, 1 out]
            n441 = local write "Magnet Status 2"(w984) -> ()
            n442 = local write "Hold"(w975) -> ()
            n443 = Bundle By Name(cluster=T31 {"Hold"=FALSE, "Clamp"=FALSE, "To Set"=FALSE, "To Zero"=FALSE, "Send to IPS"=FALSE, "PS Heat"=FALSE, "Lambda"=FALSE} ("Actions"), "Hold"=w975) -> (w978:T31)
            n444 = call "FGV_PSP - Mercury Actions.vi"("error in"=w976, "Function"=enum16{"write", "read"}."write", "Actions"=w978) -> ("error out"=w974:errorcluster)  [unwired: 3 in, 1 out]
            n445 = call <vilib>:"Add State(s) to Queue__JKI_lib_State_Machine.vi"("State(s) in (\"\")"=w990) -> ("States Out"=w991:string)  [unwired: 14 in]
          }
          frame "Mercury: Heater Current" {
            n446 = Unbundle By Name(w1017) -> ("Mercury IPS Ref"=w1020:T35)
            n447 = local read "Device Identifier"() -> (w1021:T24)
            n448 = call-poly <instrlib>:"Open.vi"("error in (no error)"=w1014, "Device Identifier"=w1021, "Mercury Reference In"=w1020) -> ("Mercury Reference Out"=w1013:T35)  [unwired: 8 out]
            n449 = call-poly <instrlib>:"Configuration (Set).vi"("error in"=w1014, "Password"="abc123", "Mode"=T32 "ENG", "Mercury Reference In"=w1013) -> ("error out"=w1011:errorcluster, "Response"=w1012:T34, "Mercury Reference Out"=w1009:T35)  [unwired: 4 in, 1 out]
            n450 = call "IPS Reply to PGSQL.vi"("error in (no error)"=w1011, "Response"=w1012) -> ("error out"=w1007:errorcluster)  [unwired: 9 in]
            n451 = call "1820 State History.vi"("initialize?"=FALSE, "Current State in"=w1012) -> ("delimited string"=w1019:string)  [unwired: 8 in, 1 out]
            n452 = local write "Magnet Status 2"(w1019) -> ()
            n453 = call <userlib>:"Wait (ms)__ogtk.vi"("error in (no error)"=w1007, "milliseconds to wait"=u32 1000) -> ("error out"=w1008:errorcluster)  [unwired: 8 in, 1 out]
            n454 = call-poly <instrlib>:"Configuration (Set).vi"("error in"=w1008, "Swh Htr Current"="Swh Htr Current (mA)", "Mercury Reference In"=w1009) -> ("error out"=w1003:errorcluster, "Response"=w993:T34, "Mercury Reference Out"=w998:T35)  [unwired: 5 in, 1 out]
            n455 = call "IPS Reply to PGSQL.vi"("error in (no error)"=w1003, "Response"=w993) -> ("error out"=w1002:errorcluster)  [unwired: 9 in]
            n456 = call "1820 State History.vi"("initialize?"=FALSE, "Current State in"=w993) -> ("delimited string"=w996:string)  [unwired: 8 in, 1 out]
            n457 = local write "Magnet Status 2"(w996) -> ()
            n458 = call <userlib>:"Wait (ms)__ogtk.vi"("error in (no error)"=w1002, "milliseconds to wait"=u32 1000) -> ("error out"=w1001:errorcluster)  [unwired: 8 in, 1 out]
            n459 = call-poly <instrlib>:"Configuration (Set).vi"("error in"=w1001, "Mode"=T32 "NORM", "Mercury Reference In"=w998) -> ("error out"=w1000:errorcluster, "Response"=w992:T34)  [unwired: 5 in, 2 out]
            n460 = call "IPS Reply to PGSQL.vi"("error in (no error)"=w1000, "Response"=w992) -> ("error out"=w999:errorcluster)  [unwired: 9 in]
            n461 = call "1820 State History.vi"("initialize?"=FALSE, "Current State in"=w992) -> ("delimited string"=w995:string)  [unwired: 8 in, 1 out]
            n462 = local write "Magnet Status 2"(w995) -> ()
            n463 = call <vilib>:"Add State(s) to Queue__JKI_lib_State_Machine.vi"("State(s) in (\"\")"=w1022) -> ("States Out"=w1023:string)  [unwired: 14 in]
          }
          frame "Mercury: Clamp" {
            w1025 = FALSE
            w1024 = T51 "CLMP" ("PSU Act Stat")
            # "#implemented: Set IPS Action"
            n464 = Unbundle By Name(w1031) -> ("Mercury IPS Ref"=w1037:T35)
            n465 = local read "Device Identifier"() -> (w1040:T24)
            n466 = call-poly <instrlib>:"Open.vi"("error in (no error)"=w1036, "Device Identifier"=w1040, "Mercury Reference In"=w1037) -> ("error out"=w1039:errorcluster, "Mercury Reference Out"=w1038:T35)  [unwired: 7 out]
            n467 = call-poly <instrlib>:"Signals (Set).vi"("error in"=w1039, "PSU Act Stat"=w1024, "Mercury Reference In"=w1038) -> ("error out"=w1035:errorcluster, "Response"=w1032:T34)  [unwired: 1 in, 6 out]
            n468 = call "Set IPS Action.vi"("PSU Act Stat"=w1024) -> ()  [unwired: 8 in, 3 out]
            n469 = call "IPS Reply to PGSQL.vi"("error in (no error)"=w1035, "Response"=w1032) -> ("error out"=w1027:errorcluster)  [unwired: 9 in]
            n470 = call "1820 State History.vi"("initialize?"=FALSE, "Current State in"=w1032) -> ("delimited string"=w1033:string)  [unwired: 8 in, 1 out]
            n471 = local write "Magnet Status 2"(w1033) -> ()
            n472 = local write "Clamp"(w1025) -> ()
            n473 = Bundle By Name(cluster=T31 {"Hold"=FALSE, "Clamp"=FALSE, "To Set"=FALSE, "To Zero"=FALSE, "Send to IPS"=FALSE, "PS Heat"=FALSE, "Lambda"=FALSE} ("Actions"), "Clamp"=w1025) -> (w1029:T31)
            n474 = call "FGV_PSP - Mercury Actions.vi"("error in"=w1027, "Function"=enum16{"write", "read"}."write", "Actions"=w1029) -> ("error out"=w1026:errorcluster)  [unwired: 3 in, 1 out]
            n475 = call <vilib>:"Add State(s) to Queue__JKI_lib_State_Machine.vi"("State(s) in (\"\")"=w1041) -> ("States Out"=w1042:string)  [unwired: 14 in]
          }
          frame "Mercury: To Set" {
            w1046 = FALSE
            w1043 = T51 "RTOS" ("PSU Act Stat")
            # "#implemented: Set IPS Action"
            n476 = Unbundle By Name(w1050) -> ("Mercury IPS Ref"=w1057:T35)
            n477 = local read "Device Identifier"() -> (w1056:T24)
            n478 = call-poly <instrlib>:"Open.vi"("error in (no error)"=w1055, "Device Identifier"=w1056, "Mercury Reference In"=w1057) -> ("error out"=w1058:errorcluster, "Mercury Reference Out"=w1059:T35)  [unwired: 7 out]
            n479 = call-poly <instrlib>:"Signals (Set).vi"("error in"=w1058, "PSU Act Stat"=w1043, "Mercury Reference In"=w1059) -> ("error out"=w1053:errorcluster, "Response"=w1052:T34)  [unwired: 1 in, 6 out]
            n480 = call "Set IPS Action.vi"("PSU Act Stat"=w1043) -> ()  [unwired: 8 in, 3 out]
            n481 = call "IPS Reply to PGSQL.vi"("error in (no error)"=w1053, "Response"=w1052) -> ("error out"=w1045:errorcluster)  [unwired: 9 in]
            n482 = call "1820 State History.vi"("initialize?"=FALSE, "Current State in"=w1052) -> ("delimited string"=w1054:string)  [unwired: 8 in, 1 out]
            n483 = local write "Magnet Status 2"(w1054) -> ()
            n484 = local write "To Set"(w1046) -> ()
            n485 = Bundle By Name(cluster=T31 {"Hold"=FALSE, "Clamp"=FALSE, "To Set"=FALSE, "To Zero"=FALSE, "Send to IPS"=FALSE, "PS Heat"=FALSE, "Lambda"=FALSE} ("Actions"), "To Set"=w1046) -> (w1048:T31)
            n486 = call "FGV_PSP - Mercury Actions.vi"("error in"=w1045, "Function"=enum16{"write", "read"}."write", "Actions"=w1048) -> ("error out"=w1044:errorcluster)  [unwired: 3 in, 1 out]
            n487 = call <vilib>:"Add State(s) to Queue__JKI_lib_State_Machine.vi"("State(s) in (\"\")"=w1060) -> ("States Out"=w1061:string)  [unwired: 14 in]
          }
          frame "Mercury: To Zero" {
            w1065 = FALSE
            w1062 = T51 "RTOZ" ("PSU Act Stat")
            # "#implemented: Set IPS Action"
            n488 = Unbundle By Name(w1069) -> ("Mercury IPS Ref"=w1076:T35)
            n489 = local read "Device Identifier"() -> (w1075:T24)
            n490 = call-poly <instrlib>:"Open.vi"("error in (no error)"=w1074, "Device Identifier"=w1075, "Mercury Reference In"=w1076) -> ("error out"=w1077:errorcluster, "Mercury Reference Out"=w1078:T35)  [unwired: 7 out]
            n491 = call-poly <instrlib>:"Signals (Set).vi"("error in"=w1077, "PSU Act Stat"=w1062, "Mercury Reference In"=w1078) -> ("error out"=w1072:errorcluster, "Response"=w1070:T34)  [unwired: 1 in, 6 out]
            n492 = call "Set IPS Action.vi"("PSU Act Stat"=w1062) -> ()  [unwired: 8 in, 3 out]
            n493 = call "IPS Reply to PGSQL.vi"("error in (no error)"=w1072, "Response"=w1070) -> ("error out"=w1064:errorcluster)  [unwired: 9 in]
            n494 = call "1820 State History.vi"("initialize?"=FALSE, "Current State in"=w1070) -> ("delimited string"=w1073:string)  [unwired: 8 in, 1 out]
            n495 = local write "Magnet Status 2"(w1073) -> ()
            n496 = local write "To Zero"(w1065) -> ()
            n497 = Bundle By Name(cluster=T31 {"Hold"=FALSE, "Clamp"=FALSE, "To Set"=FALSE, "To Zero"=FALSE, "Send to IPS"=FALSE, "PS Heat"=FALSE, "Lambda"=FALSE} ("Actions"), "To Zero"=w1065) -> (w1067:T31)
            n498 = call "FGV_PSP - Mercury Actions.vi"("error in"=w1064, "Function"=enum16{"write", "read"}."write", "Actions"=w1067) -> ("error out"=w1063:errorcluster)  [unwired: 3 in, 1 out]
            n499 = call <vilib>:"Add State(s) to Queue__JKI_lib_State_Machine.vi"("State(s) in (\"\")"=w1079) -> ("States Out"=w1080:string)  [unwired: 14 in]
          }
          frame "Mercury: PS Heat" {
            # "#implement: Set IPS Switch Heater"
            # "set switch action to F because we\nalready changed it"
            # "set the status of the switch\nT = ON\nF = OFF"
            n500 = local read "Device Identifier"() -> (w1092:T24)
            n501 = Unbundle By Name(w1087) -> ("Mercury IPS Ref"=w1093:T35)
            n502 = call-poly <instrlib>:"Open.vi"("error in (no error)"=w1089, "Device Identifier"=w1092, "Mercury Reference In"=w1093) -> ("error out"=w1090:errorcluster, "Mercury Reference Out"=w1091:T35)  [unwired: 7 out]
            n503 = call-poly <instrlib>:"Signals (Read).vi"("error in"=w1090, "Mercury Reference In"=w1091) -> ("error out"=w1095:errorcluster, "Current"=w1084:dbl, "Mercury Reference Out"=w1094:T35)  [unwired: 1 in, 6 out]
            n504 = call-poly <instrlib>:"Signals (Read).vi"("error in"=w1095, "Mercury Reference In"=w1094) -> ("error out"=w1081:errorcluster, "Persistant Current"=w1083:dbl, "Mercury Reference Out"=w1096:T35)  [unwired: 1 in, 6 out]
            n505 = Subtract(x=w1083, y=w1084) -> (x-y=w1097:dbl)
            n506 = Absolute Value(x=w1097) -> (abs(x)=w1098:dbl)
            n507 = Less?(x=w1098, y=0.1) -> (x < y?=w1100:bool)
            n508 = case shown="False" w1100 {
              selector: w1100 -> [_ w1105]
              tunnel: [w1104 w1105] -> w1082
              frame False {
                n509 = Two Button Dialog(message="The magnet current is more\nthan 0.1A different to the\nPSU output current.  It is not\nadvisable to switch on the\nswitch heater unless these\ncurrents are equal!") -> (T button?=w1104:bool)  [unwired: 2 out]
              }
              frame True {
              }
            }
            n510 = call "Set IPS Switch Heater.vi"() -> ()  [unwired: 9 in, 3 out]
            n511 = local read "PS Heat"() -> (w1086:bool)
            n512 = Or(x=w1082, y=w1086) -> (x .or. y?=w1085:bool)
            n513 = case shown="True" w1085 {
              tunnel: w1096 -> [_ w1135]
              tunnel: w1081 -> [w1106 w1134]
              tunnel: [w1106 w1121] -> w1088
              frame False {
              }
              frame True {
                w1107 = FALSE ("PS Heat")
                n514 = Get Date/Time In Seconds() -> (seconds since 1Jan1904=→"PS ON/OFF":timestamp)
                n515 = call-poly <instrlib>:"Signals (Read).vi"("error in"=w1134, "Mercury Reference In"=w1135) -> ("error out"=w1136:errorcluster, "Switch Heater Status"=w1117:string, "Mercury Reference Out"=w1118:T35)  [unwired: 1 in, 6 out]
                n516 = Equal?(x=w1117, y="ON") -> (x = y?=w1115:bool)
                n517 = call <userlib>:"Wait (ms)__ogtk.vi"("error in (no error)"=w1136, "milliseconds to wait"=u32 100 ("millisecond multiple")) -> ("error out"=w1133:errorcluster)  [unwired: 8 in, 1 out]
                n518 = Select(t=T33 "OFF" ("Set Switch Heater"), s=w1115, f=T33 "ON" ("Set Switch Heater")) -> (s? t:f=w1110:T33)
                n519 = call-poly <instrlib>:"Signals (Set).vi"("error in"=w1133, "Set Switch Heater"=w1110, "Mercury Reference In"=w1118) -> ("error out"=w1127:errorcluster, "Response"=w1125:T34, "Mercury Reference Out"=w1114:T35)  [unwired: 1 in, 5 out]
                n520 = call "1820 State History.vi"("initialize?"=FALSE, "Current State in"=w1125) -> ("delimited string"=w1129:string)  [unwired: 8 in, 1 out]
                n521 = local write "Magnet Status 2"(w1129) -> ()
                n522 = call "IPS Reply to PGSQL.vi"("error in (no error)"=w1127, "Response"=w1125) -> ("error out"=w1124:errorcluster)  [unwired: 9 in]
                n523 = while {
                  tunnel: [w1144] -> w1119
                  tunnel: w1124 -> [w1142]
                  tunnel: w1110 -> [w1140]
                  tunnel: w1114 -> [w1138]
                  tunnel: [w1137] -> w1109
                  stop <- w1139 stop-if-true
                  # "wait here while setting"
                  n524 = call-poly <instrlib>:"Signals (Read).vi"("error in"=w1142, "Mercury Reference In"=w1138) -> ("error out"=w1144:errorcluster, "Switch Heater Status"=w1141:string)  [unwired: 1 in, 7 out]
                  n525 = Equal?(x=w1141, y=w1140) -> (x = y?=w1139:bool)
                  n526 = Equal?(x=w1141, y="ON") -> (x = y?=w1137:bool)
                }
                n527 = Bundle By Name(cluster=T29 {"Magnet Field"=0.0, "PS Field"=0.0, "Target Field"=0.0, "Target Field Rate"=0.0, "Voltage"=0.0, "Current"=0.0, "Switch"=FALSE, "Mercury State"=""} ("Status"), "Switch"=w1109) -> (w1112:T29)
                n528 = call "FGV_PSP - Mercury Status.vi"("error in"=w1119, "Function"=enum16{"write", "read"}."write", "Status"=w1112) -> ("error out"=w1120:errorcluster)  [unwired: 3 in, 1 out]
                n529 = local write "PS Heat"(w1107) -> ()
                n530 = Bundle By Name(cluster=T31 {"Hold"=FALSE, "Clamp"=FALSE, "To Set"=FALSE, "To Zero"=FALSE, "Send to IPS"=FALSE, "PS Heat"=FALSE, "Lambda"=FALSE} ("Actions"), "PS Heat"=w1107) -> (w1122:T31)
                n531 = call "FGV_PSP - Mercury Actions.vi"("error in"=w1120, "Function"=enum16{"write", "read"}."write", "Actions"=w1122) -> ("error out"=w1121:errorcluster)  [unwired: 3 in, 1 out]
              }
            }
            n532 = call <vilib>:"Add State(s) to Queue__JKI_lib_State_Machine.vi"("State(s) in (\"\")"=w1101) -> ("States Out"=w1102:string)  [unwired: 14 in]
          }
          frame "Mercury: Send To IPS" {
            w1148 = FALSE
            # "#implemented: Set IPS Targets"
            n533 = local read "Device Identifier"() -> (w1167:T24)
            n534 = Unbundle By Name(w1154) -> ("Mercury IPS Ref"=w1166:T35)
            n535 = call-poly <instrlib>:"Open.vi"("error in (no error)"=w1164, "Device Identifier"=w1167, "Mercury Reference In"=w1166) -> ("error out"=w1168:errorcluster, "Mercury Reference Out"=w1165:T35)  [unwired: 7 out]
            n536 = call-poly <instrlib>:"Signals (Set).vi"("error in"=w1168, "Target Field Rate"="Target Rate (T/min)", "Mercury Reference In"=w1165) -> ("error out"=w1162:errorcluster, "Response"=w1160:T34, "Mercury Reference Out"=w1153:T35)  [unwired: 2 in, 4 out]
            n537 = call "Set IPS PSU Targets.vi"("Target Field Rate (T/min)"="Target Rate (T/min)", "Target Field (T)"="Target Field (T)") -> ()  [unwired: 7 in, 3 out]
            n538 = call "1820 State History.vi"("initialize?"=FALSE, "Current State in"=w1160) -> ("delimited string"=w1156:string)  [unwired: 8 in, 1 out]
            n539 = call "IPS Reply to PGSQL.vi"("error in (no error)"=w1162, "Response"=w1160) -> ("error out"=w1161:errorcluster)  [unwired: 9 in]
            n540 = local write "Magnet Status 2"(w1156) -> ()
            n541 = call-poly <instrlib>:"Signals (Set).vi"("error in"=w1161, "Target Field"="Target Field (T)", "Mercury Reference In"=w1153) -> ("error out"=w1163:errorcluster, "Response"=w1155:T34)  [unwired: 2 in, 5 out]
            n542 = local write "Send to IPS"(w1148) -> ()
            n543 = call "IPS Reply to PGSQL.vi"("error in (no error)"=w1163, "Response"=w1155) -> ("error out"=w1149:errorcluster)  [unwired: 9 in]
            n544 = call "1820 State History.vi"("initialize?"=FALSE, "Current State in"=w1155) -> ("delimited string"=w1157:string)  [unwired: 8 in, 1 out]
            n545 = local write "Magnet Status 2"(w1157) -> ()
            n546 = Bundle By Name(cluster=T31 {"Hold"=FALSE, "Clamp"=FALSE, "To Set"=FALSE, "To Zero"=FALSE, "Send to IPS"=FALSE, "PS Heat"=FALSE, "Lambda"=FALSE} ("Actions"), "Send to IPS"=w1148) -> (w1151:T31)
            n547 = call "FGV_PSP - Mercury Actions.vi"("error in"=w1149, "Function"=enum16{"write", "read"}."write", "Actions"=w1151) -> ("error out"=w1147:errorcluster)  [unwired: 3 in, 1 out]
            n548 = call <vilib>:"Add State(s) to Queue__JKI_lib_State_Machine.vi"("State(s) in (\"\")"=w1169) -> ("States Out"=w1170:string)  [unwired: 14 in]
          }
          frame "Mercury: Lambda" {
            # "#implemented: Set ITC LPF State"
            # "Lambda device"
            # "AUX\nPRES\nHTR\nTEMP"
            n549 = Unbundle By Name(w1180) -> ("Mercury ITC Ref"=w1189:T35)
            n550 = local read "Lambda"() -> (w1175:bool)
            n551 = call-poly <instrlib>:"Open.vi"("error in (no error)"=w1181, "Device Identifier"="lambda:LPC", "Mercury Reference In"=w1189) -> ("error out"=w1188:errorcluster, "Mercury Reference Out"=w1187:T35)  [unwired: 7 out]
            n552 = Select(t="ON" ("Sweep Mode"), s=w1175, f="OFF" ("Sweep Mode")) -> (s? t:f=w1171:string)
            n553 = case shown="False" w1175 {
              frame False {
                n554 = disable-structure shown="Disabled" {
                  frame Disabled {
                    n555 = property on="Close Needle Valve" class="Bool (strict)"("Val(Sgnl)"=TRUE ("Value (Signaling)")) -> ()  [unwired: 2 in, 2 out]
                  }
                  frame Enabled {
                  }
                }
              }
              frame True {
              }
            }
            n556 = case shown="False" w1175 {
              frame False {
                n557 = local write "LPF ON"(timestamp(0 s since 1904-01-01) ("LPF ON")) -> ()
              }
              frame True {
                n558 = Get Date/Time In Seconds() -> (seconds since 1Jan1904=w1194:timestamp)
                n559 = local write "LPF ON"(w1194) -> ()
              }
            }
            n560 = call-poly <instrlib>:"Configuration (Set).vi"("error in"=w1188, "Lambda Auto"=w1171, "Mercury Reference In"=w1187) -> ("error out"=w1185:errorcluster, "Response"=w1184:T34)  [unwired: 5 in, 2 out]
            n561 = call "Set ITC LPF State.vi"("LPF State"=w1171) -> ()  [unwired: 8 in, 3 out]
            n562 = call "ITC Reply to PGSQL.vi"("error in (no error)"=w1185, "Response"=w1184) -> ("error out"=w1176:errorcluster)  [unwired: 9 in]
            n563 = call "1820 State History.vi"("initialize?"=FALSE, "Current State in"=w1184) -> ("delimited string"=w1182:string)  [unwired: 8 in, 1 out]
            n564 = local write "Magnet Status 2"(w1182) -> ()
            n565 = Bundle By Name(cluster=T31 {"Hold"=FALSE, "Clamp"=FALSE, "To Set"=FALSE, "To Zero"=FALSE, "Send to IPS"=FALSE, "PS Heat"=FALSE, "Lambda"=FALSE} ("Actions"), "Lambda"=w1175) -> (w1178:T31)
            n566 = call "FGV_PSP - Mercury Actions.vi"("error in"=w1176, "Function"=enum16{"write", "read"}."write", "Actions"=w1178) -> ("error out"=w1174:errorcluster)  [unwired: 3 in, 1 out]
            n567 = call <vilib>:"Add State(s) to Queue__JKI_lib_State_Machine.vi"("State(s) in (\"\")"=w1190) -> ("States Out"=w1191:string)  [unwired: 14 in]
          }
          frame "Mercury: Fast/Slow Fill" {
            # "#implemented: Set IPS Fill Mode"
            # "He level sensor"
            n568 = local read "IPS Devices"() -> (w1208:string[])
            n569 = Unbundle By Name(w1196) -> ("Mercury IPS Ref"=w1210:T35)
            n570 = local read "Fast/Slow Fill"() -> (w1197:bool)
            n571 = Index Array(array=w1208, index=0) -> (element=w1205:string)
            n572 = call-poly <instrlib>:"Open.vi"("error in (no error)"=w1199, "Device Identifier"=w1205, "Mercury Reference In"=w1210) -> ("error out"=w1206:errorcluster, "Mercury Reference Out"=w1207:T35)  [unwired: 7 out]
            n573 = Select(t="OFF" ("Temperature setpoint"), s=w1197, f="ON" ("Temperature setpoint")) -> (s? t:f=w1195:string)
            n574 = call "Set IPS Fill Mode.vi"("Fill Mode"=w1195) -> ()  [unwired: 8 in, 3 out]
            n575 = call-poly <instrlib>:"Configuration (Set).vi"("error in"=w1206, "Delay"=w1195, "Mercury Reference In"=w1207) -> ("error out"=w1201:errorcluster, "Response"=w1200:T34)  [unwired: 5 in, 2 out]
            n576 = call "IPS Reply to PGSQL.vi"("error in (no error)"=w1201, "Response"=w1200) -> ("error out"=w1198:errorcluster)  [unwired: 9 in]
            n577 = call "1820 State History.vi"("Current State in"=w1200) -> ("delimited string"=w1202:string)  [unwired: 9 in, 1 out]
            n578 = local write "Magnet Status 2"(w1202) -> ()
            n579 = call <vilib>:"Add State(s) to Queue__JKI_lib_State_Machine.vi"("State(s) in (\"\")"=w1211) -> ("States Out"=w1212:string)  [unwired: 14 in]
          }
          frame "Mercury: Needle Valve" {
            # "2=open"
            # "1=closed"
            # "#implemented: Set ITC LPF Needle Valve"
            n580 = Unbundle By Name(w1217) -> ("Mercury ITC Ref"=w1214:T35)
            n581 = Build Array("Close Needle Valve", "Open Needle Valve") -> (w1225:bool[])
            n582 = call-poly <instrlib>:"Open.vi"("error in (no error)"=w1215, "Device Identifier"="lambda:LPC", "Mercury Reference In"=w1214) -> ("error out"=w1224:errorcluster, "Mercury Reference Out"=w1223:T35)  [unwired: 7 out]
            n583 = Boolean Array To Number(Boolean array=w1225) -> (number=w1222:u32)
            n584 = call "Set ITC LPF Needle Valve.vi"("Percentage Open (%)"="Percentage Open") -> ()  [unwired: 8 in, 3 out]
            n585 = case shown="0, Default" w1222 {
              tunnel: w1224 -> [w1233 w1238 w1245]
              tunnel: w1223 -> [_ w1239 w1244]
              tunnel: [w1233 w1237 w1243] -> w1219
              tunnel: [T34 "" ("Response") w1236 w1242] -> w1218
              tunnel: [FALSE ("Close Needle Valve") FALSE ("Close Needle Valve") FALSE ("Close Needle Valve")] -> w1221
              tunnel: "Percentage Open" -> [_ _ w1240]
              frame 0, Default {
              }
              frame 1 {
                n586 = call-poly <instrlib>:"Configuration (Set).vi"("error in"=w1238, "Percentage Open"=0.0, "Mercury Reference In"=w1239) -> ("error out"=w1237:errorcluster, "Response"=w1236:T34)  [unwired: 5 in, 2 out]
              }
              frame 2 {
                n587 = call-poly <instrlib>:"Configuration (Set).vi"("error in"=w1245, "Percentage Open"=w1240, "Mercury Reference In"=w1244) -> ("error out"=w1243:errorcluster, "Response"=w1242:T34)  [unwired: 5 in, 2 out]
              }
            }
            n588 = local write "Close Needle Valve"(w1221) -> ()
            n589 = local write "Open Needle Valve"(w1221) -> ()
            n590 = call "ITC Reply to PGSQL.vi"("error in (no error)"=w1219, "Response"=w1218) -> ("error out"=w1216:errorcluster)  [unwired: 9 in]
            n591 = call "1820 State History.vi"("Current State in"=w1218) -> ("delimited string"=w1220:string)  [unwired: 9 in, 1 out]
            n592 = local write "Magnet Status 2"(w1220) -> ()
            n593 = call <vilib>:"Add State(s) to Queue__JKI_lib_State_Machine.vi"("State(s) in (\"\")"=w1229) -> ("States Out"=w1230:string)  [unwired: 14 in]
          }
        }
      }
    }
    frame Enabled {
    }
  }
  n594 = disable-structure shown="Enabled" {
    frame Disabled {
      (unwired) FALSE
      n595 = call-poly <instrlib>:"Configuration (Read).vi"() -> ()  [unwired: 3 in, 9 out]
      n596 = disable-structure shown="Disabled" {
        frame Disabled {
          n597 = property on="Fast/Slow Fill" class="Bool (strict)" props=["Val(Sgnl)"]() -> ()  [unwired: 3 in, 2 out]
        }
        frame Enabled {
        }
      }
      n598 = local read "PS Heat"() -> ()  [unwired: 1 in]
      n599 = local read "Lambda"() -> ()  [unwired: 1 in]
      n600 = call-poly <instrlib>:"Signals (Read).vi"() -> ()  [unwired: 3 in, 9 out]
    }
    frame Enabled {
    }
  }
